vi "FPGA Beam Scanning V3.vi"(1 "Detectors":T1, 3 "Image Acquisition Parameters":T2={"Scan Type"=enum."Sample Scanning", "Scan Mode"=enum."XY", "Fast Axis Frequency (Hz)"=100.0, "Image Format"=128, "Line Accumulations"=1, "Frames Per Capture"=1, "Frames Accumulations"=1, "Image Dimension (um)"=[], "Number of Z Steps"=1, "Z Steps Size (um)"=1.0, "Pixel Size (nm)"=[], "Customized Image Format"=[]} {"Z Steps Size (um)" min=0.0; "Number of Z Steps" min=1; "Frames Accumulations" min=1; "Frames Per Capture" min=1; "Line Accumulations" min=1; "Image Format" items=["64 x 64"=64, "128 x 128"=128, "256 x 256"=256, "512 x 512"=512, "1024 x 1024"=1024, "2048 x 2048"=2048, "Customized..."=0]}) -> ()   [LabVIEW 2014]
uses:
  Type Defs/Image Acquisition Parameters v2.ctl
  Detectors.ctl
  <vilib>/vision/Image Controls.llb/IMAQ Image.ctl
  FPGA-7842R-Reference.ctl
  Focus Lock/Controls/Counter Action.ctl
  <vilib>/FPGAPlugInAG/PCIe-7852R/niLvFpga_Open_PCIe-7852R.vi
  <vilib>/FPGAPlugInAG/PCIe-7852R/niLvFpga_Reset_PCIe-7852R.vi
  <vilib>/Utility/error.llb/Error Cluster From Error Code.vi
  <vilib>/rvi/errors/niLvFpgaAdjustHostInterfaceError.vi
  <vilib>/rvi/interface/common/niFpgaWaitOnOcc.vi
  <vilib>/FPGAPlugInAG/PCIe-7852R/niLvFpga_Run_PCIe-7852R.vi
  <vilib>/FPGAPlugInAG/PCIe-7852R/niLvFpga_Close_PCIe-7852R.vi
  <vilib>/rvi/interface/nirviOpenFPGA/nirviOpenFPGA.xnode
  FPGA Bitfiles/MainSTEDFPGAProj_FPGATarget2_BeamScanningCamb_cWDGwb0YZ5k.lvbitx
  FPGA Target VIs/FPGA-7852R/Beam Scanning Cambridge V1.vi
  <vilib>/rvi/interface/nirviMethod/nirviMethod.xnode
  <vilib>/rvi/interface/nirviReadWriteControl/nirviReadWriteControl.xnode
  <vilib>/rvi/interface/nirviCloseFPGA/nirviCloseFPGA.xnode
  <vilib>/rvi/errors/niLvFpgaMergeErrorWithErrorCode.vi
  <vilib>/vision/NI_Vision_Development_Module.lvlib
  NiFpgaLv.dll
  <vilib>/FPGAPlugInAG/PCIe-7852R/niLvFpga_ReadFifo_PCIe-7852R.vi
  <vilib>/FPGAPlugInAG/PCIe-7852R/niLvFpga_ConfigureFifo_PCIe-7852R.vi
  <vilib>/FPGAPlugInAG/PCIe-7852R/niLvFpga_StartFifo_PCIe-7852R.vi
panel:
  # "Fast Axis"
  # "Slow Axis"
  # "XY"
  # "Z"
  # "Length"
  # "Height"
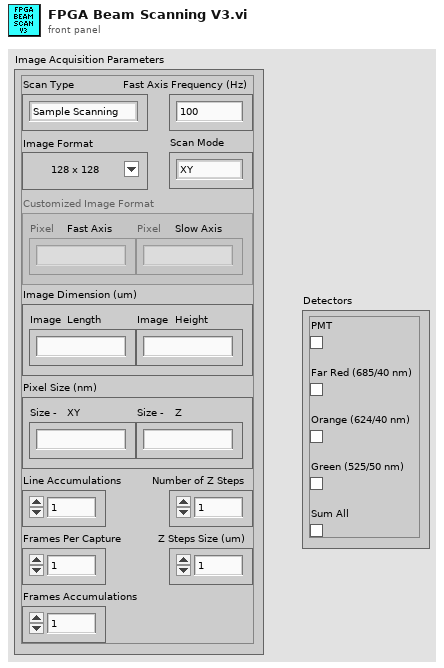
[diagram p1: front panel]
types:
  T1 = typedef "Detectors.ctl" = cluster{"PMT":bool, "Far Red (685/40 nm)":bool, "Orange (624/40 nm)":bool, "Green (525/50 nm)":bool, "Sum All":bool}
  T2 = typedef "Image Acquisition Parameters v2.ctl" = cluster{"Scan Type":enum16{"Sample Scanning", "Beam Scanning"}, "Scan Mode":enum16{"XY", "XZ", "YZ", "XYZ"}, "Fast Axis Frequency (Hz)":dbl, "Image Format":u16, "Line Accumulations":u16, "Frames Per Capture":u16, "Frames Accumulations":u16, "Image Dimension (um)":dbl[], "Number of Z Steps":u8, "Z Steps Size (um)":dbl, "Pixel Size (nm)":dbl[], "Customized Image Format":dbl[]}
  T3 = typedef "IMAQ Image.ctl" = refnum<image>
  T4 = enum16{"big-endian, network order", "native, host order", "little-endian"}
  T5 = typedef "Image Acquisition Parameters.ctl" = cluster{"Scan Type":enum16{"Sample Scanning", "Beam Scanning"}, "Scan Mode":enum16{"XY", "XZ", "YZ", "XYZ"}, "Fast Axis Frequency (Hz)":dbl, "Image Format":u16, "Line Accumulations":u16, "Frames Per Capture":u16, "Frames Accumulations":u16, "Image Dimension (um)":dbl[], "Number of Z Steps":u8, "Z Steps Size (um)":dbl, "Pixel Size (nm)":dbl[]}
  T6 = cluster{"FPGA Sampling Period (ns)":dbl, "Counting Period (us)":dbl, "Samples Per Counting Period":i32, "Start Time (us)":dbl, "Stop Time (us)":dbl, "Normalized Scan End Position":dbl, "Normalized Scan Start Position":dbl}
  T7 = typedef "Scan Parameters.ctl" = cluster{"Fast_Ax_Amp_V":dbl, "Fast_Ax_Off_V":dbl, "Slow_Ax_Amp_V":dbl, "Slow_Ax_Off_V ":dbl, "Slow_Ax_Max_V_VperS":dbl, "Slow_Ax1_Del25ns":i32, "Slow_Ax2_Del25ns":i32, "Stage_X_Off_V":dbl, "Stage_Y_Off_V":dbl, "Stage_Z_Off_V":dbl, "Galvo1_Off_V":dbl, "Galvo2_Off_V":dbl, "Last_Scan_Mode":enum16{"XY", "XZ", "YZ", "XYZ"}, "Current_Scan_Mode":enum16{"XY", "XZ", "YZ", "XYZ"}, "Fly_Back_Lines":u16, "Linear_Ramp_End":u32, "Z_Step_I16":i16, "Z_Start_I16":i16, "Laser_States _U32":u32, "590_Voltage_I16":i16, "775_AOM_Volt_I16":i16, "Blanking OFF":bool, "Unused_Axis_I16":i16}
  T8 = typedef "FPGA-7842R-Reference.ctl" = enum16{"Stage Control", "Laser Control", "Unused Axis I16", "Exit", "Set Res Mirror", "Set Galvo", "Current Frame for Capture", "Default", "Close FPGA", "Stop Waveforms", "Start Waveforms", "Shutter Control", "Initialize"}
  T9 = typedef "Counter Action.ctl" = enum16{"Zero", "Plus One", "Read"}
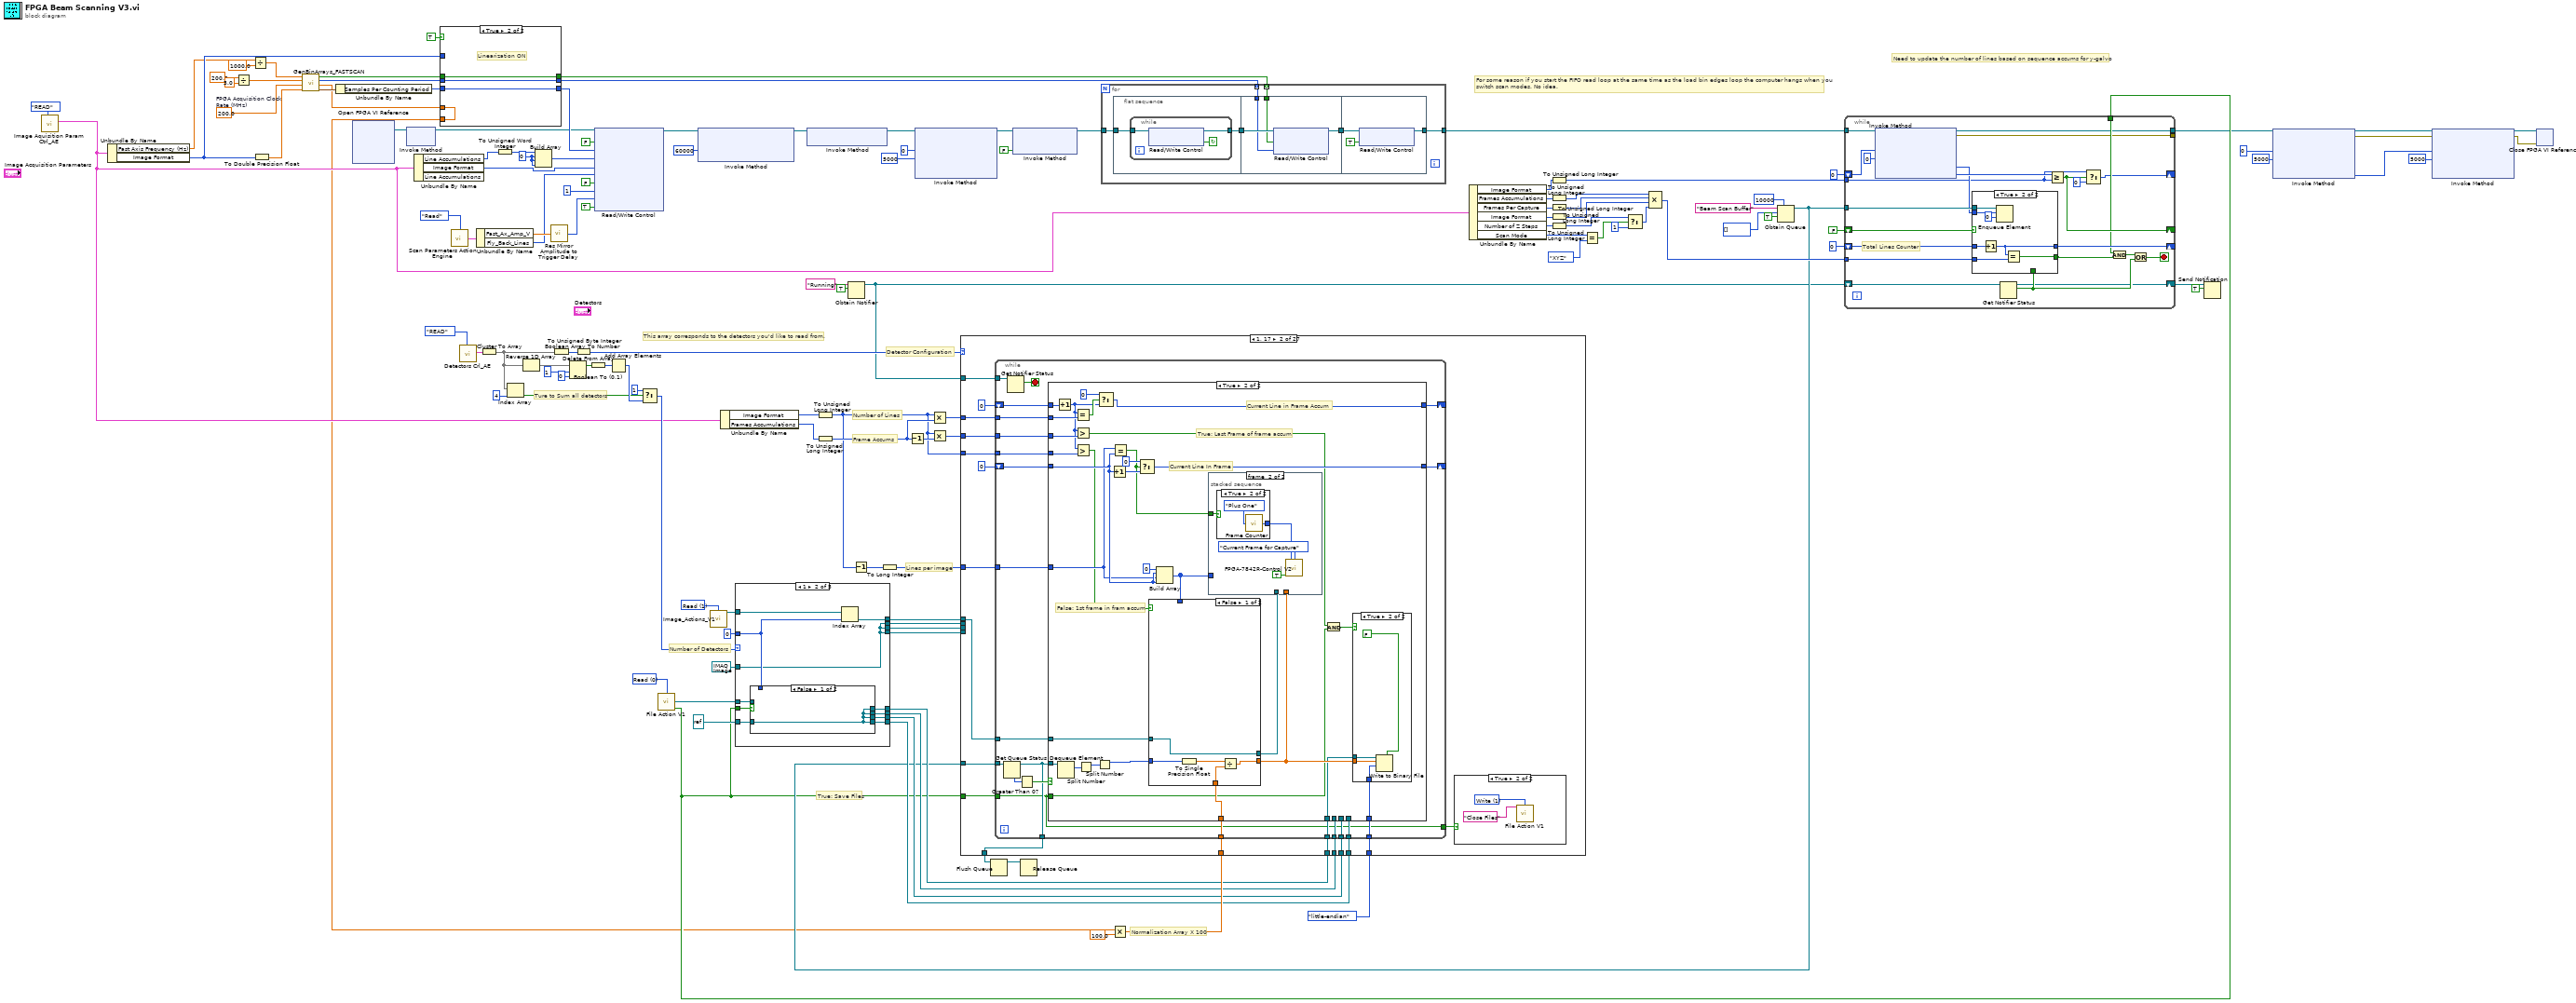
[diagram p0: block diagram]
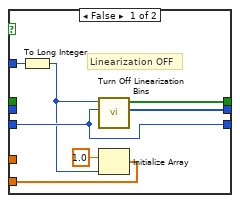
[diagram p2: hidden frame]
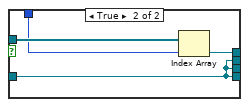
[diagram p4: hidden frame]
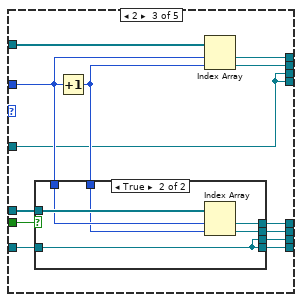
[diagram p5: hidden frame]
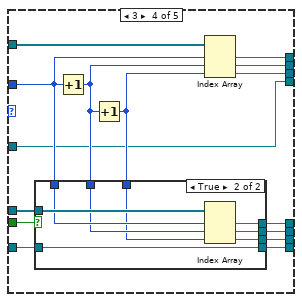
[diagram p7: hidden frame]
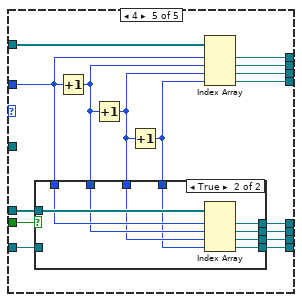
[diagram p9: hidden frame]
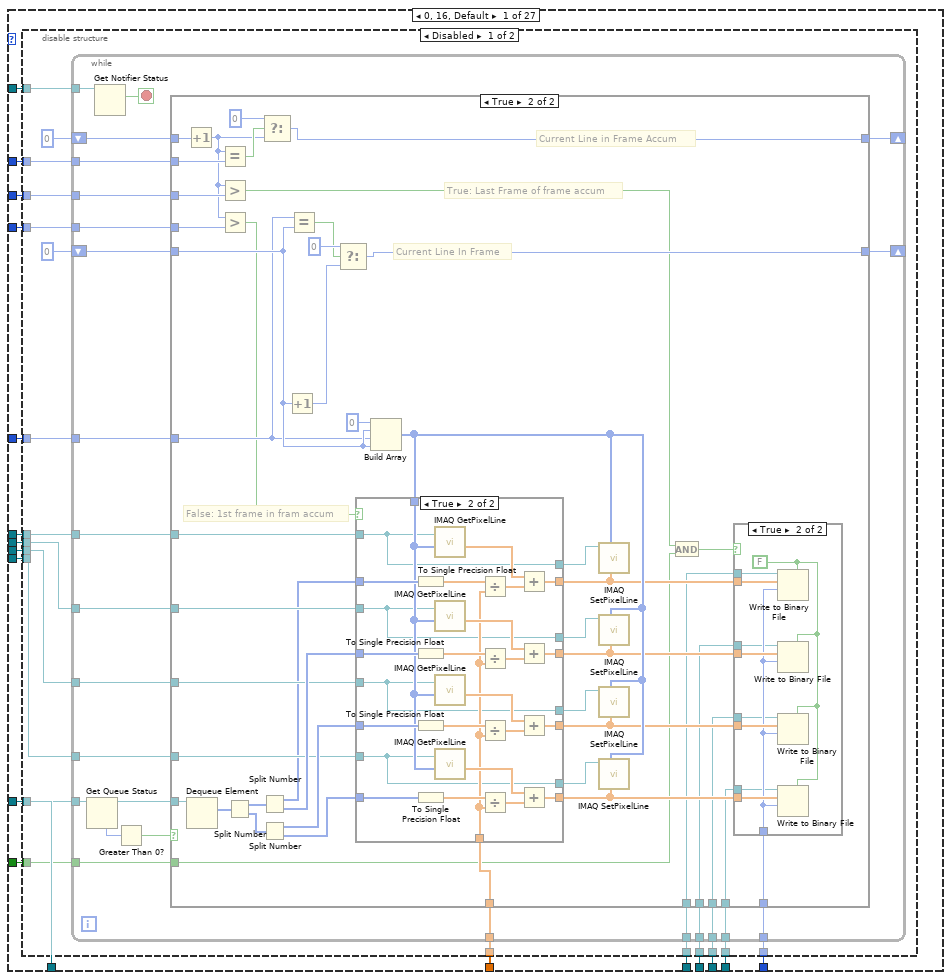
[diagram p11: hidden frame]
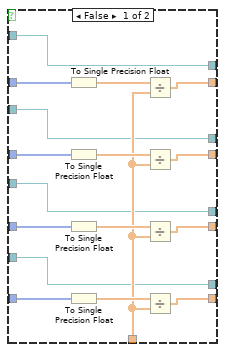
[diagram p14: hidden frame]
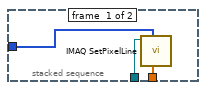
[diagram p18: hidden frame]
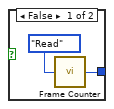
[diagram p19: hidden frame]
diagram:
  w44 = u16 0 items=["Read", "Write"] ("Mode")
  w45 = u16 0 ("element")
  w84 = u16 1 items=["Write", "Read"] ("Mode")
  w128 = 200.0  # FPGA Acquisition Clock Rate (MHz)
  # "Normalization Array X 100"
  # "This array corresponds to the detectors you'd like to read from."
  # "Ture to Sum all detectors"
  # "Number of Detectors"
  # "Detector Configuration"
  # "Frame Accums"
  # "Number of Lines"
  # "True: Save Files"
  # "Lines per image"
  # "For some reason if you start the FIFO read loop at the same time as the load bin edges loop the computer hangs when you\nswitch scan modes. No idea."
  # "Need to update the number of lines based on sequence accums for y-galvo"
  n1 = call "Image Aquisition Param Ctrl_AE.vi"("Action"=enum16{"READ", "WRITE"}."READ") -> ("Image Acquisition Parameters Out"=w33:T5)  [unwired: 10 in]
  n2 = Unbundle By Name(w33) -> ("Fast Axis Frequency (Hz)"=w18:dbl, "Image Format"=w24:u16)
  n3 = Divide(x=200.0, y=3.0) -> (x/y=w125:dbl)
  n4 = Divide(x=w18, y=1000.0) -> (x/y=w19:dbl)
  n5 = To Double Precision Float(number=w24) -> (double precision float=w111:dbl)
  n6 = call "GenBinArrays_FASTSCAN.vi"("Pixels Per Line"=w111, "FPGA Acquisition Clock Rate (MHz)"=w128, "Collection Percent (%)"=w125, "Scan Rate (kHz)"=w19) -> ("Reported Parameters"=w31:T6, "Normalization Array"=w23:sgl[], "Pre Binned Counts (x100)"=w28:u32[], "FPGA Bin Edges"=w30:bool[])
  n7 = Unbundle By Name(w31) -> ("Samples Per Counting Period"=w26:i32)
  n8 = xnode "Open FPGA VI Reference"() -> ("FPGA VI Reference Out"=w6:refnum<k20>)  [unwired: 2 in, 1 out]
  n9 = xnode "Invoke Method"("FPGA VI Reference In"=w6) -> ("FPGA VI Reference Out"=w5:refnum<k20>)  [unwired: 1 in, 1 out]
  n10 = Unbundle By Name(w33) -> ("Line Accumulations"=w53:u16, "Image Format"=w51:u16)  [unwired: 1 out]
  n11 = case shown="True" TRUE {
    tunnel: w30 -> [_ w141]
    tunnel: [w137 w141] -> w29
    tunnel: w28 -> [_ w140]
    tunnel: [w136 w140] -> w27
    tunnel: w26 -> [w135 w139]
    tunnel: [w135 w139] -> w25
    tunnel: w24 -> [w134 _]
    tunnel: w23 -> [_ w138]
    tunnel: [w131 w138] -> w22
    frame False {
      # "Linearization OFF"
      n12 = To Long Integer(number=w134) -> (32bit integer=w132:i32)
      n13 = call "Turn Off Linearization Bins.vi"("Number of Samples"=w135, "Number of Pixels"=w132) -> ("Pre Binned Values"=w136:u32[], "Equal Edges Array"=w137:bool[])  [unwired: 8 in]
      n14 = Initialize Array(sgl 1.0 ("element"), w132) -> (w131:sgl[])
    }
    frame True {
      # "Linearization ON"
    }
  }
  n15 = call "Scan Parameters Action Engine.vi"("Action"=enum16{"Read", "Write"}."Read") -> ("Scan Parameters OUT"=w49:T7)  [unwired: 14 in]
  n16 = call "Detectors Crl_AE.vi"("Action"=enum16{"READ", "WRITE"}."READ") -> ("Detectors Parameters Out"=w34:T1)  [unwired: 10 in]
  n17 = Unbundle By Name(w49) -> ("Fast_Ax_Amp_V"=w42:dbl, "Fly_Back_Lines"=w2:u16)
  n18 = Cluster To Array(cluster=w34) -> (array=w39:bool[])
  n19 = To Unsigned Word Integer(number=w53) -> (unsigned 16bit integer=w52:u16)
  n20 = Index Array(array=w39, index=4) -> (element=w37:bool)
  n21 = Reverse 1D Array(array=w39) -> (reversed array=w67:bool[])
  n22 = Build Array(w52, w45, w45, w45) -> (w8:u16[])
  n23 = call "Res Mirror Amplitude to Trigger Delay.vi"("Amplitude (V)"=w42) -> ("Trigger Delay (Ticks)"=w1:u16)
  n24 = Boolean Array To Number(Boolean array=w39) -> (number=w41:u32)
  n25 = Delete From Array(array=w67, length=1, index=0) -> (array with subset deleted=w71:bool[])  [unwired: 1 out]
  n26 = To Unsigned Byte Integer(number=w41) -> (unsigned 8bit integer=w40:u8)
  n27 = Boolean To (0,1)(Boolean=w71) -> (0, 1=w70:i16[])
  n28 = xnode "Read/Write Control"("FPGA VI Reference In"=w5, "Ready For Write"=FALSE, "FPGA Samples"=w25, "Accums Per Line"=w8, "Lines Per Image"=w51, "Dead Lines"=w2, "Line Trigger"=FALSE, "Sequences"=u8 1, "Trigger Delay (Ticks)"=w1, "Stop Acquisition"=TRUE) -> ("FPGA VI Reference Out"=w130:refnum<k20>)  [unwired: 1 in, 1 out]
  n29 = Add Array Elements(numeric array=w70) -> (sum=w69:i16)
  n30 = Select(t=i16 1, s=w37, f=w69) -> (s? t:f=w64:i16)
  n31 = call "File Action V1.vi"("Mode"=w44) -> ("File REFs"=w81:refnum<file>[], "Files Open"=w43:bool)  [unwired: 12 in, 1 out]
  n32 = xnode "Invoke Method"("FPGA VI Reference In"=w130, "Requested Depth"=u32 60000) -> ("FPGA VI Reference Out"=w109:refnum<k20>)  [unwired: 1 in, 2 out]
  n33 = call "Image_Actions_V1.vi"("Mode"=w84) -> ("Image REFs OUT"=w83:T3[])  [unwired: 13 in, 1 out]
  n34 = Unbundle By Name(w33) -> ("Image Format"=w102:u16, "Frames Accumulations"=w101:u16)
  n35 = case shown="1" w64 {
    tunnel: [w143 w144 w160 w180 w219] -> w76
    tunnel: [w143 w144 w160 w194 w218] -> w77
    tunnel: [w143 w144 w172 w193 w217] -> w78
    tunnel: [w143 w154 w171 w192 w216] -> w79
    tunnel: 0 ("Offset") -> [_ w150 w167 w188 w212]
    tunnel: w83 -> [_ w153 w170 w191 w215]
    tunnel: T3 refnum ("New Image") -> [w143 w144 w160 w180 _]
    tunnel: w81 -> [_ w151 w168 w189 w213]
    tunnel: w43 -> [_ w152 w169 w190 w214]
    tunnel: [w142 w149 w165 w185 w208] -> w75
    tunnel: [w142 w148 w164 w184 w207] -> w74
    tunnel: [w142 w147 w163 w183 w206] -> w73
    tunnel: [w142 w146 w162 w182 w205] -> w72
    tunnel: refnum<file> refnum ("element") -> [w142 w145 w161 w181 w204]
    frame 0, Default {
    }
    frame 1 {
      n36 = case shown="False" w152 {
        tunnel: w151 -> [_ w159]
        tunnel: w150 -> [_ w158]
        tunnel: [w155 w157] -> w149
        tunnel: [w155 w156] -> w148
        tunnel: [w155 w156] -> w147
        tunnel: [w155 w156] -> w146
        tunnel: w145 -> [w155 w156]
        frame False {
        }
        frame True {
          n37 = Index Array(array=w159, index=w158) -> (element=w157:refnum<file>)
        }
      }
      n38 = Index Array(array=w153, index=w150) -> (element=w154:T3)
    }
    frame 2 {
      n39 = Increment(x=w167) -> (x+1=w166:i32)
      n40 = case shown="True" w169 {
        tunnel: w168 -> [_ w179]
        tunnel: w167 -> [_ w178]
        tunnel: w166 -> [_ w177]
        tunnel: [w173 w176] -> w165
        tunnel: [w173 w175] -> w164
        tunnel: [w173 w174] -> w163
        tunnel: [w173 w174] -> w162
        tunnel: w161 -> [w173 w174]
        frame False {
        }
        frame True {
          n41 = Index Array(array=w179, index #1=w178, index #2=w177) -> (element #1=w176:refnum<file>, element #2=w175:refnum<file>)
        }
      }
      n42 = Index Array(array=w170, index #1=w167, index #2=w166) -> (element #1=w171:T3, element #2=w172:T3)
    }
    frame 3 {
      n43 = Increment(x=w188) -> (x+1=w187:i32)
      n44 = Increment(x=w187) -> (x+1=w186:i32)
      n45 = case shown="True" w190 {
        tunnel: w189 -> [_ w203]
        tunnel: w188 -> [_ w202]
        tunnel: w187 -> [_ w201]
        tunnel: w186 -> [_ w200]
        tunnel: [w195 w199] -> w185
        tunnel: [w195 w198] -> w184
        tunnel: [w195 w197] -> w183
        tunnel: [w195 w196] -> w182
        tunnel: w181 -> [w195 w196]
        frame False {
        }
        frame True {
          n46 = Index Array(array=w203, index #1=w202, index #2=w201, index #3=w200) -> (element #1=w199:refnum<file>, element #2=w198:refnum<file>, element #3=w197:refnum<file>)
        }
      }
      n47 = Index Array(array=w191, index #1=w188, index #2=w187, index #3=w186) -> (element #1=w192:T3, element #2=w193:T3, element #3=w194:T3)
    }
    frame 4 {
      n48 = Increment(x=w212) -> (x+1=w211:i32)
      n49 = Increment(x=w211) -> (x+1=w210:i32)
      n50 = Increment(x=w210) -> (x+1=w209:i32)
      n51 = case shown="True" w214 {
        tunnel: w213 -> [_ w229]
        tunnel: w212 -> [_ w228]
        tunnel: w211 -> [_ w227]
        tunnel: w210 -> [_ w226]
        tunnel: w209 -> [_ w225]
        tunnel: [w220 w224] -> w208
        tunnel: [w220 w223] -> w207
        tunnel: [w220 w222] -> w206
        tunnel: [w220 w221] -> w205
        tunnel: w204 -> [w220 _]
        frame False {
        }
        frame True {
          n52 = Index Array(array=w229, index #1=w228, index #2=w227, index #3=w226, index #4=w225) -> (element #1=w224:refnum<file>, element #2=w223:refnum<file>, element #3=w222:refnum<file>, element #4=w221:refnum<file>)
        }
      }
      n53 = Index Array(array=w215, index #1=w212, index #2=w211, index #3=w210, index #4=w209) -> (element #1=w216:T3, element #2=w217:T3, element #3=w218:T3, element #4=w219:T3)
    }
  }
  n54 = xnode "Invoke Method"("FPGA VI Reference In"=w109) -> ("FPGA VI Reference Out"=w110:refnum<k20>)  [unwired: 1 in, 1 out]
  n55 = To Unsigned Long Integer(number=w102) -> (unsigned 32bit integer=w87:u32)
  n56 = To Unsigned Long Integer(number=w101) -> (unsigned 32bit integer=w88:u32)
  n57 = Obtain Notifier(name (unnamed)="Running", notification data type=TRUE) -> (notifier out=w32:refnum<notifier>)  [unwired: 2 in, 2 out]
  n58 = Decrement(x=w87) -> (x-1=w85:u32)
  n59 = To Long Integer(number=w85) -> (32bit integer=w93:i32)
  n60 = Decrement(x=w88) -> (x-1=w91:u32)
  n61 = xnode "Invoke Method"("FPGA VI Reference In"=w110, "Number of Elements"=u32 0, "Timeout (ms)"=5000) -> ("FPGA VI Reference Out"=w129:refnum<k20>)  [unwired: 1 in, 3 out]
  n62 = Multiply(x=w87, y=w88) -> (x*y=w89:u32)
  n63 = Multiply(x=w87, y=w91) -> (x*y=w90:u32)
  n64 = xnode "Invoke Method"("FPGA VI Reference In"=w129, "Wait Until Done (F)"=FALSE) -> ("FPGA VI Reference Out"=w124:refnum<k20>)  [unwired: 1 in, 1 out]
  n65 = for {
    tunnel: [w233] -> w99
    tunnel: w124 -> [w232]
    tunnel: w29 -> [w231] mode=indexing
    tunnel: w27 -> [w230] mode=indexing
    n66 = flat-sequence {
      tunnel: [w237] -> w235
      tunnel: w232 -> [w236]
      tunnel: w235 -> [w244]
      tunnel: [w243] -> w234
      tunnel: w231 -> [w242]
      tunnel: w230 -> [w241]
      tunnel: w234 -> [w247]
      tunnel: [w246] -> w233
      frame #0 {
        n67 = while {
          tunnel: [w240] -> w237
          tunnel: w236 -> [w239]
          stop <- w238 continue-if-true
          n68 = xnode "Read/Write Control"("FPGA VI Reference In"=w239) -> ("FPGA VI Reference Out"=w240:refnum<k20>, "Ready For Write"=w238:bool)  [unwired: 1 in, 1 out]
        }
      }
      frame #1 {
        n69 = xnode "Read/Write Control"("FPGA VI Reference In"=w244, "BinEdge"=w242, "PreBinnedValue"=w241) -> ("FPGA VI Reference Out"=w243:refnum<k20>)  [unwired: 1 in, 1 out]
      }
      frame #2 {
        n70 = xnode "Read/Write Control"("FPGA VI Reference In"=w247, "Ready For Write"=TRUE) -> ("FPGA VI Reference Out"=w246:refnum<k20>)  [unwired: 1 in, 1 out]
      }
    }
  }
  n71 = Multiply(x=w22, y=sgl 100.0) -> (x*y=w100:sgl[])
  n72 = Unbundle By Name(w33) -> ("Image Format"=w116:u16, "Frames Accumulations"=w61:u16, "Frames Per Capture"=w117:u16, "Image Format"=w62:u16, "Number of Z Steps"=w58:u8, "Scan Mode"=w59:enum16{"XY", "XZ", "YZ", "XYZ"})
  n73 = To Unsigned Long Integer(number=w116) -> (unsigned 32bit integer=w123:u32)
  n74 = To Unsigned Long Integer(number=w61) -> (unsigned 32bit integer=w57:u32)
  n75 = To Unsigned Long Integer(number=w117) -> (unsigned 32bit integer=w56:u32)
  n76 = To Unsigned Long Integer(number=w62) -> (unsigned 32bit integer=w55:u32)
  n77 = To Unsigned Long Integer(number=w58) -> (unsigned 32bit integer=w54:u32)
  n78 = Equal?(x=w59, y=enum16{"XY", "XZ", "YZ", "XYZ"}."XYZ") -> (x = y?=w105:bool)
  n79 = Select(t=w54, s=w105, f=u32 1) -> (s? t:f=w104:u32)
  n80 = Compound Arithmetic op=MULTIPLY(w57, w56, w55, w104) -> (w118:u32)
  n81 = Obtain Queue(max queue size (-1, unlimited)=10000, name (unnamed)="Beam Scan Buffer", element data type=u64[] [], create if not found? (T)=TRUE) -> (queue out=w47:refnum<queue>)  [unwired: 1 in, 2 out]
  n82 = case shown="1, 17" w40 {
    tunnel: w93 -> [w264 w426 w526 w626 w743 w842 w961 w1081 w1217 w1316 w1435 w1555 w1692 w1811 w1949 w2088 w2242 w2342 w2443 w2544 w2647 w2748 w2849 w2952 w3052 w3155 w3258]
    tunnel: w43 -> [w261 w423 w523 w623 w740 w839 w958 w1078 w1214 w1313 w1432 w1552 w1689 w1808 w1946 w2085 w2239 w2339 w2440 w2541 w2644 w2745 w2846 w2949 w3049 w3152 w3255]
    tunnel: T4."little-endian" ("byte order (0:big-endian, network order)") -> [w263 w425 w525 w625 w742 w841 w960 w1080 w1216 w1315 w1434 w1554 w1691 w1810 w1948 w2087 w2241 w2341 w2442 w2543 w2646 w2747 w2848 w2951 w3051 w3154 w3257]
    tunnel: w100 -> [w262 w424 w524 w624 w741 w840 w959 w1079 w1215 w1314 w1433 w1553 w1690 w1809 w1947 w2086 w2240 w2340 w2441 w2542 w2645 w2746 w2847 w2950 w3050 w3153 w3256]
    tunnel: w90 -> [w260 w421 w521 w621 w738 w837 w956 w1076 w1212 w1311 w1430 w1550 w1687 w1806 w1944 w2083 w2237 w2337 w2438 w2539 w2642 w2743 w2844 w2947 w3047 w3150 w3253]
    tunnel: w89 -> [w259 w420 w520 w620 w737 w836 w955 w1075 w1211 w1310 w1429 w1549 w1686 w1805 w1943 w2082 w2236 w2336 w2437 w2538 w2641 w2742 w2843 w2946 w3046 w3149 w3252]
    tunnel: w87 -> [w258 w419 w519 w619 w736 w835 w954 w1074 w1210 w1309 w1428 w1548 w1685 w1804 w1942 w2081 w2235 w2335 w2436 w2537 w2640 w2741 w2842 w2945 w3045 w3148 w3251]
    tunnel: w47 -> [w257 w418 w518 w612 w735 w834 w953 w1073 w1209 w1308 w1427 w1547 w1684 w1803 w1941 w2080 w2234 w2334 w2435 w2536 w2639 w2740 w2841 w2944 w3044 w3147 w3250]
    tunnel: w79 -> [w252 w413 w513 w614 w730 w829 w948 w1068 w1204 w1303 w1422 w1542 w1679 w1798 w1936 w2075 w2229 w2329 w2430 w2531 w2634 w2735 w2836 w2939 w3039 w3142 w3245]
    tunnel: w78 -> [w251 _ _ w613 _ w828 w947 w1067 _ w1302 w1421 w1541 w1678 w1797 w1935 w2074 _ _ _ _ _ _ _ _ _ _ _]
    tunnel: w77 -> [w250 _ _ _ _ _ _ w1066 _ _ _ w1540 _ w1796 w1934 w2073 _ _ _ _ _ _ _ _ _ _ _]
    tunnel: w76 -> [w249 _ _ _ _ _ _ _ _ _ _ _ _ _ _ w2072 _ _ _ _ _ _ _ _ _ _ _]
    tunnel: [w257 w412 w518 w611 w735 w834 w953 w1073 w1209 w1308 w1427 w1547 w1684 w1803 w1941 w2080 w2234 w2334 w2435 w2536 w2639 w2740 w2841 w2944 w3044 w3147 w3250] -> w46
    tunnel: w75 -> [w256 w417 w517 w618 w734 w833 w952 w1072 w1208 w1307 w1426 w1546 w1683 w1802 w1940 w2079 w2233 w2333 w2434 w2535 w2638 w2739 w2840 w2943 w3043 w3146 w3249]
    tunnel: w74 -> [w255 w416 w516 w617 w733 w832 w951 w1071 w1207 w1306 w1425 w1545 w1682 w1801 w1939 w2078 w2232 w2332 w2433 w2534 w2637 w2738 w2839 w2942 w3042 w3145 w3248]
    tunnel: w73 -> [w254 w415 w515 w616 w732 w831 w950 w1070 w1206 w1305 w1424 w1544 w1681 w1800 w1938 w2077 w2231 w2331 w2432 w2533 w2636 w2737 w2838 w2941 w3041 w3144 w3247]
    tunnel: w72 -> [w253 w414 w514 w615 w731 w830 w949 w1069 w1205 w1304 w1423 w1543 w1680 w1799 w1937 w2076 w2230 w2330 w2431 w2532 w2635 w2736 w2837 w2940 w3040 w3143 w3246]
    tunnel: w32 -> [w248 w410 w512 w610 w729 w827 w946 w1065 w1203 w1301 w1420 w1539 w1677 w1795 w1933 w2071 w2228 w2328 w2429 w2530 w2633 w2734 w2835 w2938 w3038 w3141 w3244]
    frame 0, 16, Default {
      n83 = disable-structure shown="Disabled" {
        disable-tunnel: w264 -> [w282 _]
        disable-tunnel: w263 -> [w281 _]
        disable-tunnel: w262 -> [w280 _]
        disable-tunnel: w261 -> [w279 _]
        disable-tunnel: w248 -> [w278 _]
        disable-tunnel: w260 -> [w276 _]
        disable-tunnel: w259 -> [w275 _]
        disable-tunnel: w258 -> [w274 _]
        disable-tunnel: w257 -> [w273 _]
        disable-tunnel: w256 -> [w272 _]
        disable-tunnel: w255 -> [w271 _]
        disable-tunnel: w254 -> [w270 _]
        disable-tunnel: w253 -> [w269 _]
        disable-tunnel: w252 -> [w268 _]
        disable-tunnel: w251 -> [w267 _]
        disable-tunnel: w250 -> [w266 _]
        disable-tunnel: w249 -> [w265 _]
        frame Disabled {
          n84 = while {
            shift-right: [w306] -> _
            shift-left: 0 -> [w307]
            tunnel: w282 -> [w308]
            tunnel: w281 -> [w305]
            tunnel: w280 -> [w304]
            tunnel: w279 -> [w303]
            tunnel: w278 -> [w299]
            shift-right: [w296] -> _
            shift-left: u32 0 -> [w297]
            tunnel: w276 -> [w295]
            tunnel: w275 -> [w294]
            tunnel: w274 -> [w293]
            tunnel: w273 -> [w292]
            tunnel: w268 -> [w291]
            tunnel: w267 -> [w290]
            tunnel: w266 -> [w289]
            tunnel: w265 -> [w288]
            tunnel: w272 -> [w287]
            tunnel: w271 -> [w286]
            tunnel: w270 -> [w285]
            tunnel: w269 -> [w284]
            stop <- w298 stop-if-true
            n85 = Get Queue Status(queue=w292) -> (queue out=w300:refnum<queue>, # elements in queue=w302:i32)  [unwired: 2 in, 6 out]
            n86 = Get Notifier Status(notifier=w299) -> (current notification=w298:bool)  [unwired: 1 in, 4 out]
            n87 = Greater Than 0?(x=w302) -> (x > 0?=w301:bool)
            n88 = case shown="True" w301 {
              tunnel: w308 -> [_ w345]
              tunnel: w307 -> [w310 w346]
              tunnel: [w310 w344] -> w306
              tunnel: w305 -> [_ w338]
              tunnel: w304 -> [_ w337]
              tunnel: w303 -> [_ w327]
              tunnel: w300 -> [_ w336]
              tunnel: w297 -> [w309 w333]
              tunnel: [w309 w332] -> w296
              tunnel: w295 -> [_ w331]
              tunnel: w294 -> [_ w330]
              tunnel: w293 -> [_ w325]
              tunnel: w291 -> [_ w323]
              tunnel: w290 -> [_ w322]
              tunnel: w289 -> [_ w321]
              tunnel: w288 -> [_ w320]
              tunnel: w287 -> [_ w314]
              tunnel: w286 -> [_ w313]
              tunnel: w285 -> [_ w312]
              tunnel: w284 -> [_ w311]
              frame False {
              }
              frame True {
                # "False: 1st frame in fram accum"
                # "True: Last Frame of frame accum"
                # "Current Line in Frame Accum"
                # "Current Line In Frame"
                n89 = Increment(x=w333) -> (x+1=w326:u32)
                n90 = Dequeue Element(queue=w336) -> (element=w355:u64[])  [unwired: 2 in, 3 out]
                n91 = Equal?(x=w326, y=w330) -> (x = y?=w335:bool)
                n92 = Greater?(x=w326, y=w331) -> (0:w328:bool)
                n93 = Greater?(x=w326, y=w325) -> (0:w324:bool)
                n94 = Split Number(x=w355) -> (hi(x)=w356:u32[], lo(x)=w354:u32[])
                n95 = Split Number(x=w356) -> (hi(x)=w315:u16[], lo(x)=w353:u16[])
                n96 = Split Number(x=w354) -> (hi(x)=w352:u16[], lo(x)=w351:u16[])
                n97 = Select(t=u32 0, s=w335, f=w326) -> (s? t:f=w332:u32)
                n98 = Increment(x=w346) -> (x+1=w348:i32)
                n99 = Equal?(x=w345, y=w346) -> (x = y?=w347:bool)
                n100 = Select(t=0, s=w347, f=w348) -> (s? t:f=w344:i32)
                n101 = Build Array(0, w346, w345, w346) -> (w343:i32[])
                n102 = case shown="True" w324 {
                  tunnel: w315 -> [w382 w409]
                  tunnel: w353 -> [w377 w408]
                  tunnel: w352 -> [w376 w407]
                  tunnel: w351 -> [w375 w406]
                  tunnel: [w373 w398] -> w340
                  tunnel: [w374 w397] -> w341
                  tunnel: [w381 w396] -> w342
                  tunnel: [w372 w395] -> w339
                  tunnel: w343 -> [_ w390]
                  tunnel: w337 -> [w371 w388]
                  tunnel: w323 -> [w370 w385]
                  tunnel: w322 -> [w369 w386]
                  tunnel: w321 -> [w368 w387]
                  tunnel: w320 -> [w367 w384]
                  tunnel: [w368 w387] -> w317
                  tunnel: [w369 w386] -> w318
                  tunnel: [w370 w385] -> w319
                  tunnel: [w367 w384] -> w316
                  frame False {
                    n103 = To Single Precision Float(number=w382) -> (single precision float=w383:sgl[])
                    n104 = To Single Precision Float(number=w377) -> (single precision float=w380:sgl[])
                    n105 = To Single Precision Float(number=w376) -> (single precision float=w379:sgl[])
                    n106 = To Single Precision Float(number=w375) -> (single precision float=w378:sgl[])
                    n107 = Divide(x=w383, y=w371) -> (x/y=w381:sgl[])
                    n108 = Divide(x=w380, y=w371) -> (x/y=w374:sgl[])
                    n109 = Divide(x=w379, y=w371) -> (x/y=w373:sgl[])
                    n110 = Divide(x=w378, y=w371) -> (x/y=w372:sgl[])
                  }
                  frame True {
                    n111 = To Single Precision Float(number=w409) -> (single precision float=w389:sgl[])
                    n112 = To Single Precision Float(number=w408) -> (single precision float=w405:sgl[])
                    n113 = To Single Precision Float(number=w407) -> (single precision float=w404:sgl[])
                    n114 = To Single Precision Float(number=w406) -> (single precision float=w403:sgl[])
                    n115 = call "IMAQ GetPixelLine"("Line Coordinates"=w390, "Image"=w385) -> ("Pixels Line (Float)"=w394:sgl[])  [unwired: 2 in, 4 out]
                    n116 = call "IMAQ GetPixelLine"("Line Coordinates"=w390, "Image"=w386) -> ("Pixels Line (Float)"=w393:sgl[])  [unwired: 2 in, 4 out]
                    n117 = call "IMAQ GetPixelLine"("Line Coordinates"=w390, "Image"=w387) -> ("Pixels Line (Float)"=w392:sgl[])  [unwired: 2 in, 4 out]
                    n118 = call "IMAQ GetPixelLine"("Line Coordinates"=w390, "Image"=w384) -> ("Pixels Line (Float)"=w391:sgl[])  [unwired: 2 in, 4 out]
                    n119 = Divide(x=w389, y=w388) -> (x/y=w402:sgl[])
                    n120 = Divide(x=w405, y=w388) -> (x/y=w401:sgl[])
                    n121 = Divide(x=w404, y=w388) -> (x/y=w400:sgl[])
                    n122 = Divide(x=w403, y=w388) -> (x/y=w399:sgl[])
                    n123 = Add(x=w394, y=w402) -> (x+y=w396:sgl[])
                    n124 = Add(x=w393, y=w401) -> (x+y=w397:sgl[])
                    n125 = Add(x=w392, y=w400) -> (x+y=w398:sgl[])
                    n126 = Add(x=w391, y=w399) -> (x+y=w395:sgl[])
                  }
                }
                n127 = call "IMAQ SetPixelLine"("Pixels Line (Float)"=w342, "Line Coordinates"=w343, "Image"=w319) -> ()  [unwired: 7 in, 2 out]
                n128 = call "IMAQ SetPixelLine"("Pixels Line (Float)"=w341, "Line Coordinates"=w343, "Image"=w318) -> ()  [unwired: 7 in, 2 out]
                n129 = call "IMAQ SetPixelLine"("Pixels Line (Float)"=w340, "Line Coordinates"=w343, "Image"=w317) -> ()  [unwired: 7 in, 2 out]
                n130 = call "IMAQ SetPixelLine"("Pixels Line (Float)"=w339, "Line Coordinates"=w343, "Image"=w316) -> ()  [unwired: 7 in, 2 out]
                n131 = And(x=w328, y=w327) -> (x .and. y?=w329:bool)
                n132 = case shown="True" w329 {
                  tunnel: w342 -> [_ w366]
                  tunnel: w341 -> [_ w365]
                  tunnel: w340 -> [_ w364]
                  tunnel: w339 -> [_ w363]
                  tunnel: w338 -> [_ w361]
                  tunnel: w314 -> [_ w360]
                  tunnel: w313 -> [_ w359]
                  tunnel: w312 -> [_ w358]
                  tunnel: w311 -> [_ w357]
                  frame False {
                  }
                  frame True {
                    w362 = FALSE ("prepend array or string size? (T)")
                    n133 = Write to Binary File(file (use dialog)=w360, data=w366, 5:w362, 9:w361) -> ()  [unwired: 2 in, 3 out]
                    n134 = Write to Binary File(file (use dialog)=w359, data=w365, 5:w362, 9:w361) -> ()  [unwired: 2 in, 3 out]
                    n135 = Write to Binary File(file (use dialog)=w358, data=w364, 5:w362, 9:w361) -> ()  [unwired: 2 in, 3 out]
                    n136 = Write to Binary File(file (use dialog)=w357, data=w363, 5:w362, 9:w361) -> ()  [unwired: 2 in, 3 out]
                  }
                }
              }
            }
          }
        }
        frame Enabled {
        }
      }
    }
    frame 1, 17 {
      n137 = while {
        shift-right: [w449] -> _
        shift-left: 0 -> [w450]
        tunnel: w426 -> [w451]
        tunnel: w425 -> [w448]
        tunnel: w424 -> [w447]
        tunnel: w423 -> [w430]
        tunnel: w410 -> [w444]
        shift-right: [w441] -> _
        shift-left: u32 0 -> [w442]
        tunnel: w421 -> [w440]
        tunnel: w420 -> [w439]
        tunnel: w419 -> [w438]
        tunnel: w418 -> [w437]
        tunnel: w413 -> [w436]
        tunnel: w417 -> [w435]
        tunnel: w416 -> [w434]
        tunnel: w415 -> [w433]
        tunnel: w414 -> [w432]
        tunnel: [w431] -> w412
        tunnel: [w430] -> w411
        stop <- w443 stop-if-true
        n138 = Get Queue Status(queue=w437) -> (queue out=w431:refnum<queue>, # elements in queue=w446:i32)  [unwired: 2 in, 6 out]
        n139 = Get Notifier Status(notifier=w444) -> (current notification=w443:bool)  [unwired: 1 in, 4 out]
        n140 = Greater Than 0?(x=w446) -> (x > 0?=w445:bool)
        n141 = case shown="True" w445 {
          tunnel: w451 -> [_ w479]
          tunnel: w450 -> [w453 w480]
          tunnel: [w453 w478] -> w449
          tunnel: w448 -> [_ w475]
          tunnel: w447 -> [_ w474]
          tunnel: w430 -> [_ w457]
          tunnel: w431 -> [_ w473]
          tunnel: w442 -> [w452 w470]
          tunnel: [w452 w469] -> w441
          tunnel: w440 -> [_ w468]
          tunnel: w439 -> [_ w467]
          tunnel: w438 -> [_ w463]
          tunnel: w436 -> [_ w461]
          tunnel: w435 -> [_ w459]
          tunnel: w434 -> [_ _]
          tunnel: w433 -> [_ _]
          tunnel: w432 -> [_ _]
          frame False {
          }
          frame True {
            # "False: 1st frame in fram accum"
            # "True: Last Frame of frame accum"
            # "Current Line in Frame Accum"
            # "Current Line In Frame"
            n142 = Increment(x=w470) -> (x+1=w464:u32)
            n143 = Dequeue Element(queue=w473) -> (element=w482:u64[])  [unwired: 2 in, 3 out]
            n144 = Equal?(x=w464, y=w467) -> (x = y?=w472:bool)
            n145 = Greater?(x=w464, y=w468) -> (0:w465:bool)
            n146 = Greater?(x=w464, y=w463) -> (0:w462:bool)
            n147 = Split Number(x=w482) -> (hi(x)=w483:u32[])  [unwired: 1 out]
            n148 = Split Number(x=w483) -> (hi(x)=w458:u16[])  [unwired: 1 out]
            n149 = Select(t=u32 0, s=w472, f=w464) -> (s? t:f=w469:u32)
            n150 = Increment(x=w480) -> (x+1=w456:i32)
            n151 = Equal?(x=w479, y=w480) -> (x = y?=w454:bool)
            n152 = Select(t=0, s=w454, f=w456) -> (s? t:f=w478:i32)
            n153 = Build Array(0, w480, w479, w480) -> (w477:i32[])
            n154 = case shown="False" w462 {
              tunnel: w458 -> [w502 w511]
              tunnel: [w501 w508] -> w476
              tunnel: w477 -> [_ w506]
              tunnel: w474 -> [w500 w505]
              tunnel: w461 -> [w499 w504]
              tunnel: [w499 w504] -> w460
              frame False {
                n155 = To Single Precision Float(number=w502) -> (single precision float=w503:sgl[])
                n156 = Divide(x=w503, y=w500) -> (x/y=w501:sgl[])
              }
              frame True {
                n157 = To Single Precision Float(number=w511) -> (single precision float=w510:sgl[])
                n158 = call "IMAQ GetPixelLine"("Line Coordinates"=w506, "Image"=w504) -> ("Pixels Line (Float)"=w507:sgl[])  [unwired: 2 in, 4 out]
                n159 = Divide(x=w510, y=w505) -> (x/y=w509:sgl[])
                n160 = Add(x=w507, y=w509) -> (x+y=w508:sgl[])
              }
            }
            n161 = stacked-sequence {
              tunnel: w477 -> [w486 _]
              tunnel: w476 -> [w485 _]
              tunnel: w460 -> [w484 _]
              tunnel: w454 -> [_ w490]
              frame #0 {
                n162 = call "IMAQ SetPixelLine"("Pixels Line (Float)"=w485, "Line Coordinates"=w486, "Image"=w484) -> ()  [unwired: 7 in, 2 out]
              }
              frame #1 {
                n163 = case shown="True" w490 {
                  tunnel: [w491 w493] -> w488
                  frame False {
                    n164 = call "Frame Counter.vi"("Action"=Counter_Action."Read") -> ("Num"=w491:i32)
                  }
                  frame True {
                    n165 = call "Frame Counter.vi"("Action"=Counter_Action."Plus One") -> ("Num"=w493:i32)
                  }
                }
                n166 = call "FPGA-7842R-Control V2.vi"("Current Frame"=w488, "Action"=FPGA-7842R-Reference."Current Frame for Capture", "Initialize"=TRUE) -> ()  [unwired: 11 in, 2 out]
              }
            }
            n167 = And(x=w465, y=w457) -> (x .and. y?=w466:bool)
            n168 = case shown="True" w466 {
              tunnel: w476 -> [_ w498]
              tunnel: w475 -> [_ w496]
              tunnel: w459 -> [_ w495]
              frame False {
              }
              frame True {
                n169 = Write to Binary File(file (use dialog)=w495, data=w498, 5:FALSE ("prepend array or string size? (T)"), 9:w496) -> ()  [unwired: 2 in, 3 out]
              }
            }
          }
        }
      }
      n170 = case shown="True" w411 {
        frame False {
        }
        frame True {
          w429 = u16 1 items=["Read", "Write"] ("Mode")
          n171 = call "File Action V1.vi"("Action"="Close Files", "Mode"=w429) -> ()  [unwired: 11 in, 3 out]
        }
      }
    }
    frame 2, 18 {
      n172 = while {
        shift-right: [w547] -> _
        shift-left: 0 -> [w548]
        tunnel: w526 -> [w549]
        tunnel: w525 -> [w546]
        tunnel: w524 -> [w545]
        tunnel: w523 -> [w544]
        tunnel: w512 -> [w540]
        shift-right: [w537] -> _
        shift-left: u32 0 -> [w538]
        tunnel: w521 -> [w536]
        tunnel: w520 -> [w535]
        tunnel: w519 -> [w534]
        tunnel: w518 -> [w533]
        tunnel: w513 -> [w532]
        tunnel: w517 -> [w531]
        tunnel: w516 -> [w530]
        tunnel: w515 -> [w529]
        tunnel: w514 -> [w528]
        stop <- w539 stop-if-true
        n173 = Get Queue Status(queue=w533) -> (queue out=w541:refnum<queue>, # elements in queue=w543:i32)  [unwired: 2 in, 6 out]
        n174 = Get Notifier Status(notifier=w540) -> (current notification=w539:bool)  [unwired: 1 in, 4 out]
        n175 = Greater Than 0?(x=w543) -> (x > 0?=w542:bool)
        n176 = case shown="True" w542 {
          tunnel: w549 -> [_ w576]
          tunnel: w548 -> [w551 w577]
          tunnel: [w551 w575] -> w547
          tunnel: w546 -> [_ w574]
          tunnel: w545 -> [_ w573]
          tunnel: w544 -> [_ w563]
          tunnel: w541 -> [_ w572]
          tunnel: w538 -> [w550 w569]
          tunnel: [w550 w568] -> w537
          tunnel: w536 -> [_ w567]
          tunnel: w535 -> [_ w566]
          tunnel: w534 -> [_ w561]
          tunnel: w532 -> [_ w559]
          tunnel: w531 -> [_ w558]
          tunnel: w530 -> [_ _]
          tunnel: w529 -> [_ _]
          tunnel: w528 -> [_ _]
          frame False {
          }
          frame True {
            # "False: 1st frame in fram accum"
            # "True: Last Frame of frame accum"
            # "Current Line in Frame Accum"
            # "Current Line In Frame"
            n177 = Increment(x=w569) -> (x+1=w562:u32)
            n178 = Dequeue Element(queue=w572) -> (element=w580:u64[])  [unwired: 2 in, 3 out]
            n179 = Equal?(x=w562, y=w566) -> (x = y?=w571:bool)
            n180 = Greater?(x=w562, y=w567) -> (0:w564:bool)
            n181 = Greater?(x=w562, y=w561) -> (0:w560:bool)
            n182 = Split Number(x=w580) -> (hi(x)=w581:u32[])  [unwired: 1 out]
            n183 = Split Number(x=w581) -> (lo(x)=w557:u16[])  [unwired: 1 out]
            n184 = Select(t=u32 0, s=w571, f=w562) -> (s? t:f=w568:u32)
            n185 = Increment(x=w577) -> (x+1=w578:i32)
            n186 = Equal?(x=w576, y=w577) -> (x = y?=w552:bool)
            n187 = Select(t=0, s=w552, f=w578) -> (s? t:f=w575:i32)
            n188 = Build Array(0, w577, w576, w577) -> (w555:i32[])
            n189 = case shown="True" w560 {
              tunnel: w557 -> [w600 w609]
              tunnel: [w599 w606] -> w553
              tunnel: w555 -> [_ w604]
              tunnel: w573 -> [w598 w603]
              tunnel: w559 -> [w597 w602]
              tunnel: [w597 w602] -> w554
              frame False {
                n190 = To Single Precision Float(number=w600) -> (single precision float=w601:sgl[])
                n191 = Divide(x=w601, y=w598) -> (x/y=w599:sgl[])
              }
              frame True {
                n192 = To Single Precision Float(number=w609) -> (single precision float=w608:sgl[])
                n193 = call "IMAQ GetPixelLine"("Line Coordinates"=w604, "Image"=w602) -> ("Pixels Line (Float)"=w605:sgl[])  [unwired: 2 in, 4 out]
                n194 = Divide(x=w608, y=w603) -> (x/y=w607:sgl[])
                n195 = Add(x=w605, y=w607) -> (x+y=w606:sgl[])
              }
            }
            n196 = stacked-sequence {
              tunnel: w555 -> [w584 _]
              tunnel: w553 -> [w583 _]
              tunnel: w554 -> [w582 _]
              tunnel: w552 -> [_ w588]
              frame #0 {
                n197 = call "IMAQ SetPixelLine"("Pixels Line (Float)"=w583, "Line Coordinates"=w584, "Image"=w582) -> ()  [unwired: 7 in, 2 out]
              }
              frame #1 {
                n198 = case shown="True" w588 {
                  tunnel: [w589 w591] -> w586
                  frame False {
                    n199 = call "Frame Counter.vi"("Action"=Counter_Action."Read") -> ("Num"=w589:i32)
                  }
                  frame True {
                    n200 = call "Frame Counter.vi"("Action"=Counter_Action."Plus One") -> ("Num"=w591:i32)
                  }
                }
                n201 = call "FPGA-7842R-Control V2.vi"("Current Frame"=w586, "Action"=FPGA-7842R-Reference."Current Frame for Capture", "Initialize"=TRUE) -> ()  [unwired: 11 in, 2 out]
              }
            }
            n202 = And(x=w564, y=w563) -> (x .and. y?=w565:bool)
            n203 = case shown="True" w565 {
              tunnel: w553 -> [_ w596]
              tunnel: w574 -> [_ w594]
              tunnel: w558 -> [_ w593]
              frame False {
              }
              frame True {
                n204 = Write to Binary File(file (use dialog)=w593, data=w596, 5:FALSE ("prepend array or string size? (T)"), 9:w594) -> ()  [unwired: 2 in, 3 out]
              }
            }
          }
        }
      }
    }
    frame 3 {
      n205 = while {
        shift-right: [w648] -> _
        shift-left: 0 -> [w649]
        tunnel: w626 -> [w650]
        tunnel: w625 -> [w647]
        tunnel: w624 -> [w646]
        tunnel: w623 -> [w645]
        tunnel: w610 -> [w642]
        shift-right: [w639] -> _
        shift-left: u32 0 -> [w640]
        tunnel: w621 -> [w638]
        tunnel: w620 -> [w637]
        tunnel: w619 -> [w636]
        tunnel: w612 -> [w635]
        tunnel: w614 -> [w634]
        tunnel: w613 -> [w633]
        tunnel: w618 -> [w632]
        tunnel: w617 -> [w631]
        tunnel: w616 -> [w630]
        tunnel: w615 -> [w629]
        tunnel: [w628] -> w611
        stop <- w641 stop-if-true
        n206 = Get Queue Status(queue=w635) -> (queue out=w628:refnum<queue>, # elements in queue=w644:i32)  [unwired: 2 in, 6 out]
        n207 = Get Notifier Status(notifier=w642) -> (current notification=w641:bool)  [unwired: 1 in, 4 out]
        n208 = Greater Than 0?(x=w644) -> (x > 0?=w643:bool)
        n209 = case shown="True" w643 {
          tunnel: w650 -> [_ w682]
          tunnel: w649 -> [w652 w683]
          tunnel: [w652 w681] -> w648
          tunnel: w647 -> [_ w679]
          tunnel: w646 -> [_ w678]
          tunnel: w645 -> [_ w668]
          tunnel: w628 -> [_ w677]
          tunnel: w640 -> [w651 w674]
          tunnel: [w651 w673] -> w639
          tunnel: w638 -> [_ w672]
          tunnel: w637 -> [_ w671]
          tunnel: w636 -> [_ w666]
          tunnel: w634 -> [_ w664]
          tunnel: w633 -> [_ w663]
          tunnel: w632 -> [_ w661]
          tunnel: w631 -> [_ w660]
          tunnel: w630 -> [_ _]
          tunnel: w629 -> [_ _]
          frame False {
          }
          frame True {
            # "False: 1st frame in fram accum"
            # "True: Last Frame of frame accum"
            # "Current Line in Frame Accum"
            # "Current Line In Frame"
            n210 = Increment(x=w674) -> (x+1=w667:u32)
            n211 = Dequeue Element(queue=w677) -> (element=w687:u64[])  [unwired: 2 in, 3 out]
            n212 = Equal?(x=w667, y=w671) -> (x = y?=w676:bool)
            n213 = Greater?(x=w667, y=w672) -> (0:w669:bool)
            n214 = Greater?(x=w667, y=w666) -> (0:w665:bool)
            n215 = Split Number(x=w687) -> (hi(x)=w688:u32[])  [unwired: 1 out]
            n216 = Split Number(x=w688) -> (hi(x)=w659:u16[], lo(x)=w658:u16[])
            n217 = Select(t=u32 0, s=w676, f=w667) -> (s? t:f=w673:u32)
            n218 = Increment(x=w683) -> (x+1=w684:i32)
            n219 = Equal?(x=w682, y=w683) -> (x = y?=w653:bool)
            n220 = Select(t=0, s=w653, f=w684) -> (s? t:f=w681:i32)
            n221 = Build Array(0, w683, w682, w683) -> (w657:i32[])
            n222 = case shown="True" w665 {
              tunnel: w659 -> [w712 w728]
              tunnel: w658 -> [w711 w727]
              tunnel: [w709 w722] -> w680
              tunnel: [w710 w721] -> w654
              tunnel: w657 -> [_ w718]
              tunnel: w678 -> [w708 w717]
              tunnel: w664 -> [w707 w715]
              tunnel: w663 -> [w706 w716]
              tunnel: [w706 w716] -> w662
              tunnel: [w707 w715] -> w655
              frame False {
                n223 = To Single Precision Float(number=w712) -> (single precision float=w714:sgl[])
                n224 = To Single Precision Float(number=w711) -> (single precision float=w713:sgl[])
                n225 = Divide(x=w714, y=w708) -> (x/y=w710:sgl[])
                n226 = Divide(x=w713, y=w708) -> (x/y=w709:sgl[])
              }
              frame True {
                n227 = To Single Precision Float(number=w728) -> (single precision float=w726:sgl[])
                n228 = To Single Precision Float(number=w727) -> (single precision float=w725:sgl[])
                n229 = call "IMAQ GetPixelLine"("Line Coordinates"=w718, "Image"=w715) -> ("Pixels Line (Float)"=w720:sgl[])  [unwired: 2 in, 4 out]
                n230 = call "IMAQ GetPixelLine"("Line Coordinates"=w718, "Image"=w716) -> ("Pixels Line (Float)"=w719:sgl[])  [unwired: 2 in, 4 out]
                n231 = Divide(x=w726, y=w717) -> (x/y=w724:sgl[])
                n232 = Divide(x=w725, y=w717) -> (x/y=w723:sgl[])
                n233 = Add(x=w720, y=w724) -> (x+y=w721:sgl[])
                n234 = Add(x=w719, y=w723) -> (x+y=w722:sgl[])
              }
            }
            n235 = stacked-sequence {
              tunnel: w657 -> [w689 _]
              tunnel: w654 -> [w691 _]
              tunnel: w655 -> [w690 _]
              tunnel: w653 -> [_ w695]
              tunnel: [w689 _] -> w656
              frame #0 {
                n236 = call "IMAQ SetPixelLine"("Pixels Line (Float)"=w691, "Line Coordinates"=w689, "Image"=w690) -> ()  [unwired: 7 in, 2 out]
              }
              frame #1 {
                n237 = case shown="True" w695 {
                  tunnel: [w696 w698] -> w693
                  frame False {
                    n238 = call "Frame Counter.vi"("Action"=Counter_Action."Read") -> ("Num"=w696:i32)
                  }
                  frame True {
                    n239 = call "Frame Counter.vi"("Action"=Counter_Action."Plus One") -> ("Num"=w698:i32)
                  }
                }
                n240 = call "FPGA-7842R-Control V2.vi"("Current Frame"=w693, "Action"=FPGA-7842R-Reference."Current Frame for Capture", "Initialize"=TRUE) -> ()  [unwired: 11 in, 2 out]
              }
            }
            n241 = call "IMAQ SetPixelLine"("Pixels Line (Float)"=w680, "Line Coordinates"=w656, "Image"=w662) -> ()  [unwired: 7 in, 2 out]
            n242 = And(x=w669, y=w668) -> (x .and. y?=w670:bool)
            n243 = case shown="False" w670 {
              tunnel: w654 -> [_ w705]
              tunnel: w680 -> [_ w704]
              tunnel: w679 -> [_ w702]
              tunnel: w661 -> [_ w701]
              tunnel: w660 -> [_ w700]
              frame False {
              }
              frame True {
                w703 = FALSE ("prepend array or string size? (T)")
                n244 = Write to Binary File(file (use dialog)=w701, data=w705, 5:w703, 9:w702) -> ()  [unwired: 2 in, 3 out]
                n245 = Write to Binary File(file (use dialog)=w700, data=w704, 5:w703, 9:w702) -> ()  [unwired: 2 in, 3 out]
              }
            }
          }
        }
      }
    }
    frame 4, 20 {
      n246 = while {
        shift-right: [w764] -> _
        shift-left: 0 -> [w765]
        tunnel: w743 -> [w766]
        tunnel: w742 -> [w763]
        tunnel: w741 -> [w762]
        tunnel: w740 -> [w761]
        tunnel: w729 -> [w757]
        shift-right: [w754] -> _
        shift-left: u32 0 -> [w755]
        tunnel: w738 -> [w753]
        tunnel: w737 -> [w752]
        tunnel: w736 -> [w751]
        tunnel: w735 -> [w750]
        tunnel: w730 -> [w749]
        tunnel: w734 -> [w748]
        tunnel: w733 -> [w747]
        tunnel: w732 -> [w746]
        tunnel: w731 -> [w745]
        stop <- w756 stop-if-true
        n247 = Get Queue Status(queue=w750) -> (queue out=w758:refnum<queue>, # elements in queue=w760:i32)  [unwired: 2 in, 6 out]
        n248 = Get Notifier Status(notifier=w757) -> (current notification=w756:bool)  [unwired: 1 in, 4 out]
        n249 = Greater Than 0?(x=w760) -> (x > 0?=w759:bool)
        n250 = case shown="True" w759 {
          tunnel: w766 -> [_ w792]
          tunnel: w765 -> [w768 w793]
          tunnel: [w768 w791] -> w764
          tunnel: w763 -> [_ w790]
          tunnel: w762 -> [_ w789]
          tunnel: w761 -> [_ w779]
          tunnel: w758 -> [_ w788]
          tunnel: w755 -> [w767 w785]
          tunnel: [w767 w784] -> w754
          tunnel: w753 -> [_ w783]
          tunnel: w752 -> [_ w782]
          tunnel: w751 -> [_ w777]
          tunnel: w749 -> [_ w775]
          tunnel: w748 -> [_ w774]
          tunnel: w747 -> [_ _]
          tunnel: w746 -> [_ _]
          tunnel: w745 -> [_ _]
          frame False {
          }
          frame True {
            # "False: 1st frame in fram accum"
            # "True: Last Frame of frame accum"
            # "Current Line in Frame Accum"
            # "Current Line In Frame"
            n251 = Increment(x=w785) -> (x+1=w778:u32)
            n252 = Dequeue Element(queue=w788) -> (element=w798:u64[])  [unwired: 2 in, 3 out]
            n253 = Equal?(x=w778, y=w782) -> (x = y?=w787:bool)
            n254 = Greater?(x=w778, y=w783) -> (0:w780:bool)
            n255 = Greater?(x=w778, y=w777) -> (0:w776:bool)
            n256 = Split Number(x=w798) -> (lo(x)=w797:u32[])  [unwired: 1 out]
            n257 = Split Number(x=w797) -> (hi(x)=w773:u16[])  [unwired: 1 out]
            n258 = Select(t=u32 0, s=w787, f=w778) -> (s? t:f=w784:u32)
            n259 = Increment(x=w793) -> (x+1=w794:i32)
            n260 = Equal?(x=w792, y=w793) -> (x = y?=w772:bool)
            n261 = Select(t=0, s=w772, f=w794) -> (s? t:f=w791:i32)
            n262 = Build Array(0, w793, w792, w793) -> (w771:i32[])
            n263 = case shown="True" w776 {
              tunnel: w773 -> [w817 w826]
              tunnel: [w816 w823] -> w769
              tunnel: w771 -> [_ w821]
              tunnel: w789 -> [w815 w820]
              tunnel: w775 -> [w814 w819]
              tunnel: [w814 w819] -> w770
              frame False {
                n264 = To Single Precision Float(number=w817) -> (single precision float=w818:sgl[])
                n265 = Divide(x=w818, y=w815) -> (x/y=w816:sgl[])
              }
              frame True {
                n266 = To Single Precision Float(number=w826) -> (single precision float=w825:sgl[])
                n267 = call "IMAQ GetPixelLine"("Line Coordinates"=w821, "Image"=w819) -> ("Pixels Line (Float)"=w822:sgl[])  [unwired: 2 in, 4 out]
                n268 = Divide(x=w825, y=w820) -> (x/y=w824:sgl[])
                n269 = Add(x=w822, y=w824) -> (x+y=w823:sgl[])
              }
            }
            n270 = stacked-sequence {
              tunnel: w771 -> [w801 _]
              tunnel: w769 -> [w800 _]
              tunnel: w770 -> [w799 _]
              tunnel: w772 -> [_ w805]
              frame #0 {
                n271 = call "IMAQ SetPixelLine"("Pixels Line (Float)"=w800, "Line Coordinates"=w801, "Image"=w799) -> ()  [unwired: 7 in, 2 out]
              }
              frame #1 {
                n272 = case shown="True" w805 {
                  tunnel: [w806 w808] -> w803
                  frame False {
                    n273 = call "Frame Counter.vi"("Action"=Counter_Action."Read") -> ("Num"=w806:i32)
                  }
                  frame True {
                    n274 = call "Frame Counter.vi"("Action"=Counter_Action."Plus One") -> ("Num"=w808:i32)
                  }
                }
                n275 = call "FPGA-7842R-Control V2.vi"("Current Frame"=w803, "Action"=FPGA-7842R-Reference."Current Frame for Capture", "Initialize"=TRUE) -> ()  [unwired: 11 in, 2 out]
              }
            }
            n276 = And(x=w780, y=w779) -> (x .and. y?=w781:bool)
            n277 = case shown="True" w781 {
              tunnel: w769 -> [_ w813]
              tunnel: w790 -> [_ w811]
              tunnel: w774 -> [_ w810]
              frame False {
              }
              frame True {
                n278 = Write to Binary File(file (use dialog)=w810, data=w813, 5:FALSE ("prepend array or string size? (T)"), 9:w811) -> ()  [unwired: 2 in, 3 out]
              }
            }
          }
        }
      }
    }
    frame 5 {
      n279 = while {
        shift-right: [w864] -> _
        shift-left: 0 -> [w865]
        tunnel: w842 -> [w866]
        tunnel: w841 -> [w863]
        tunnel: w840 -> [w862]
        tunnel: w839 -> [w861]
        tunnel: w827 -> [w857]
        shift-right: [w854] -> _
        shift-left: u32 0 -> [w855]
        tunnel: w837 -> [w853]
        tunnel: w836 -> [w852]
        tunnel: w835 -> [w851]
        tunnel: w834 -> [w850]
        tunnel: w829 -> [w849]
        tunnel: w828 -> [w848]
        tunnel: w833 -> [w847]
        tunnel: w832 -> [w846]
        tunnel: w831 -> [w845]
        tunnel: w830 -> [w844]
        stop <- w856 stop-if-true
        n280 = Get Queue Status(queue=w850) -> (queue out=w858:refnum<queue>, # elements in queue=w860:i32)  [unwired: 2 in, 6 out]
        n281 = Get Notifier Status(notifier=w857) -> (current notification=w856:bool)  [unwired: 1 in, 4 out]
        n282 = Greater Than 0?(x=w860) -> (x > 0?=w859:bool)
        n283 = case shown="True" w859 {
          tunnel: w866 -> [_ w897]
          tunnel: w865 -> [w868 w898]
          tunnel: [w868 w896] -> w864
          tunnel: w863 -> [_ w894]
          tunnel: w862 -> [_ w893]
          tunnel: w861 -> [_ w883]
          tunnel: w858 -> [_ w892]
          tunnel: w855 -> [w867 w889]
          tunnel: [w867 w888] -> w854
          tunnel: w853 -> [_ w887]
          tunnel: w852 -> [_ w886]
          tunnel: w851 -> [_ w881]
          tunnel: w849 -> [_ w879]
          tunnel: w848 -> [_ w878]
          tunnel: w847 -> [_ w875]
          tunnel: w846 -> [_ w874]
          tunnel: w845 -> [_ _]
          tunnel: w844 -> [_ _]
          frame False {
          }
          frame True {
            # "False: 1st frame in fram accum"
            # "True: Last Frame of frame accum"
            # "Current Line in Frame Accum"
            # "Current Line In Frame"
            n284 = Increment(x=w889) -> (x+1=w882:u32)
            n285 = Dequeue Element(queue=w892) -> (element=w904:u64[])  [unwired: 2 in, 3 out]
            n286 = Equal?(x=w882, y=w886) -> (x = y?=w891:bool)
            n287 = Greater?(x=w882, y=w887) -> (0:w884:bool)
            n288 = Greater?(x=w882, y=w881) -> (0:w880:bool)
            n289 = Split Number(x=w904) -> (hi(x)=w905:u32[], lo(x)=w903:u32[])
            n290 = Split Number(x=w905) -> (hi(x)=w876:u16[])  [unwired: 1 out]
            n291 = Split Number(x=w903) -> (hi(x)=w902:u16[])  [unwired: 1 out]
            n292 = Select(t=u32 0, s=w891, f=w882) -> (s? t:f=w888:u32)
            n293 = Increment(x=w898) -> (x+1=w899:i32)
            n294 = Equal?(x=w897, y=w898) -> (x = y?=w869:bool)
            n295 = Select(t=0, s=w869, f=w899) -> (s? t:f=w896:i32)
            n296 = Build Array(0, w898, w897, w898) -> (w873:i32[])
            n297 = case shown="False" w880 {
              tunnel: w876 -> [w930 w945]
              tunnel: w902 -> [w927 w944]
              tunnel: [w926 w940] -> w895
              tunnel: [w929 w939] -> w871
              tunnel: w873 -> [_ w936]
              tunnel: w893 -> [w925 w934]
              tunnel: w879 -> [w924 w932]
              tunnel: w878 -> [w923 w933]
              tunnel: [w923 w933] -> w877
              tunnel: [w924 w932] -> w872
              frame False {
                n298 = To Single Precision Float(number=w930) -> (single precision float=w931:sgl[])
                n299 = To Single Precision Float(number=w927) -> (single precision float=w928:sgl[])
                n300 = Divide(x=w931, y=w925) -> (x/y=w929:sgl[])
                n301 = Divide(x=w928, y=w925) -> (x/y=w926:sgl[])
              }
              frame True {
                n302 = To Single Precision Float(number=w945) -> (single precision float=w935:sgl[])
                n303 = To Single Precision Float(number=w944) -> (single precision float=w943:sgl[])
                n304 = call "IMAQ GetPixelLine"("Line Coordinates"=w936, "Image"=w932) -> ("Pixels Line (Float)"=w938:sgl[])  [unwired: 2 in, 4 out]
                n305 = call "IMAQ GetPixelLine"("Line Coordinates"=w936, "Image"=w933) -> ("Pixels Line (Float)"=w937:sgl[])  [unwired: 2 in, 4 out]
                n306 = Divide(x=w935, y=w934) -> (x/y=w942:sgl[])
                n307 = Divide(x=w943, y=w934) -> (x/y=w941:sgl[])
                n308 = Add(x=w938, y=w942) -> (x+y=w939:sgl[])
                n309 = Add(x=w937, y=w941) -> (x+y=w940:sgl[])
              }
            }
            n310 = stacked-sequence {
              tunnel: w873 -> [w906 _]
              tunnel: w871 -> [w908 _]
              tunnel: w872 -> [w907 _]
              tunnel: w869 -> [_ w912]
              tunnel: [w906 _] -> w870
              frame #0 {
                n311 = call "IMAQ SetPixelLine"("Pixels Line (Float)"=w908, "Line Coordinates"=w906, "Image"=w907) -> ()  [unwired: 7 in, 2 out]
              }
              frame #1 {
                n312 = case shown="True" w912 {
                  tunnel: [w913 w915] -> w910
                  frame False {
                    n313 = call "Frame Counter.vi"("Action"=Counter_Action."Read") -> ("Num"=w913:i32)
                  }
                  frame True {
                    n314 = call "Frame Counter.vi"("Action"=Counter_Action."Plus One") -> ("Num"=w915:i32)
                  }
                }
                n315 = call "FPGA-7842R-Control V2.vi"("Current Frame"=w910, "Action"=FPGA-7842R-Reference."Current Frame for Capture", "Initialize"=TRUE) -> ()  [unwired: 11 in, 2 out]
              }
            }
            n316 = call "IMAQ SetPixelLine"("Pixels Line (Float)"=w895, "Line Coordinates"=w870, "Image"=w877) -> ()  [unwired: 7 in, 2 out]
            n317 = And(x=w884, y=w883) -> (x .and. y?=w885:bool)
            n318 = case shown="True" w885 {
              tunnel: w871 -> [_ w922]
              tunnel: w895 -> [_ w921]
              tunnel: w894 -> [_ w919]
              tunnel: w875 -> [_ w918]
              tunnel: w874 -> [_ w917]
              frame False {
              }
              frame True {
                w920 = FALSE ("prepend array or string size? (T)")
                n319 = Write to Binary File(file (use dialog)=w918, data=w922, 5:w920, 9:w919) -> ()  [unwired: 2 in, 3 out]
                n320 = Write to Binary File(file (use dialog)=w917, data=w921, 5:w920, 9:w919) -> ()  [unwired: 2 in, 3 out]
              }
            }
          }
        }
      }
    }
    frame 6 {
      n321 = while {
        shift-right: [w983] -> _
        shift-left: 0 -> [w984]
        tunnel: w961 -> [w985]
        tunnel: w960 -> [w982]
        tunnel: w959 -> [w981]
        tunnel: w958 -> [w980]
        tunnel: w946 -> [w976]
        shift-right: [w973] -> _
        shift-left: u32 0 -> [w974]
        tunnel: w956 -> [w972]
        tunnel: w955 -> [w971]
        tunnel: w954 -> [w970]
        tunnel: w953 -> [w969]
        tunnel: w948 -> [w968]
        tunnel: w947 -> [w967]
        tunnel: w952 -> [w966]
        tunnel: w951 -> [w965]
        tunnel: w950 -> [w964]
        tunnel: w949 -> [w963]
        stop <- w975 stop-if-true
        n322 = Get Queue Status(queue=w969) -> (queue out=w977:refnum<queue>, # elements in queue=w979:i32)  [unwired: 2 in, 6 out]
        n323 = Get Notifier Status(notifier=w976) -> (current notification=w975:bool)  [unwired: 1 in, 4 out]
        n324 = Greater Than 0?(x=w979) -> (x > 0?=w978:bool)
        n325 = case shown="True" w978 {
          tunnel: w985 -> [_ w1015]
          tunnel: w984 -> [w987 w1016]
          tunnel: [w987 w1014] -> w983
          tunnel: w982 -> [_ w1012]
          tunnel: w981 -> [_ w1011]
          tunnel: w980 -> [_ w1001]
          tunnel: w977 -> [_ w1010]
          tunnel: w974 -> [w986 w1007]
          tunnel: [w986 w1006] -> w973
          tunnel: w972 -> [_ w1005]
          tunnel: w971 -> [_ w1004]
          tunnel: w970 -> [_ w999]
          tunnel: w968 -> [_ w997]
          tunnel: w967 -> [_ w996]
          tunnel: w966 -> [_ w994]
          tunnel: w965 -> [_ w993]
          tunnel: w964 -> [_ _]
          tunnel: w963 -> [_ _]
          frame False {
          }
          frame True {
            # "False: 1st frame in fram accum"
            # "True: Last Frame of frame accum"
            # "Current Line in Frame Accum"
            # "Current Line In Frame"
            n326 = Increment(x=w1007) -> (x+1=w1000:u32)
            n327 = Dequeue Element(queue=w1010) -> (element=w1023:u64[])  [unwired: 2 in, 3 out]
            n328 = Equal?(x=w1000, y=w1004) -> (x = y?=w1009:bool)
            n329 = Greater?(x=w1000, y=w1005) -> (0:w1002:bool)
            n330 = Greater?(x=w1000, y=w999) -> (0:w998:bool)
            n331 = Split Number(x=w1023) -> (hi(x)=w1024:u32[], lo(x)=w1022:u32[])
            n332 = Split Number(x=w1024) -> (lo(x)=w1021:u16[])  [unwired: 1 out]
            n333 = Split Number(x=w1022) -> (hi(x)=w1020:u16[])  [unwired: 1 out]
            n334 = Select(t=u32 0, s=w1009, f=w1000) -> (s? t:f=w1006:u32)
            n335 = Increment(x=w1016) -> (x+1=w1017:i32)
            n336 = Equal?(x=w1015, y=w1016) -> (x = y?=w992:bool)
            n337 = Select(t=0, s=w992, f=w1017) -> (s? t:f=w1014:i32)
            n338 = Build Array(0, w1016, w1015, w1016) -> (w991:i32[])
            n339 = case shown="False" w998 {
              tunnel: w1021 -> [w1048 w1064]
              tunnel: w1020 -> [w1047 w1063]
              tunnel: [w1045 w1058] -> w1013
              tunnel: [w1046 w1057] -> w989
              tunnel: w991 -> [_ w1054]
              tunnel: w1011 -> [w1044 w1053]
              tunnel: w997 -> [w1043 w1051]
              tunnel: w996 -> [w1042 w1052]
              tunnel: [w1042 w1052] -> w995
              tunnel: [w1043 w1051] -> w990
              frame False {
                n340 = To Single Precision Float(number=w1048) -> (single precision float=w1050:sgl[])
                n341 = To Single Precision Float(number=w1047) -> (single precision float=w1049:sgl[])
                n342 = Divide(x=w1050, y=w1044) -> (x/y=w1046:sgl[])
                n343 = Divide(x=w1049, y=w1044) -> (x/y=w1045:sgl[])
              }
              frame True {
                n344 = To Single Precision Float(number=w1064) -> (single precision float=w1062:sgl[])
                n345 = To Single Precision Float(number=w1063) -> (single precision float=w1061:sgl[])
                n346 = call "IMAQ GetPixelLine"("Line Coordinates"=w1054, "Image"=w1051) -> ("Pixels Line (Float)"=w1056:sgl[])  [unwired: 2 in, 4 out]
                n347 = call "IMAQ GetPixelLine"("Line Coordinates"=w1054, "Image"=w1052) -> ("Pixels Line (Float)"=w1055:sgl[])  [unwired: 2 in, 4 out]
                n348 = Divide(x=w1062, y=w1053) -> (x/y=w1060:sgl[])
                n349 = Divide(x=w1061, y=w1053) -> (x/y=w1059:sgl[])
                n350 = Add(x=w1056, y=w1060) -> (x+y=w1057:sgl[])
                n351 = Add(x=w1055, y=w1059) -> (x+y=w1058:sgl[])
              }
            }
            n352 = stacked-sequence {
              tunnel: w991 -> [w1025 _]
              tunnel: w989 -> [w1027 _]
              tunnel: w990 -> [w1026 _]
              tunnel: w992 -> [_ w1031]
              tunnel: [w1025 _] -> w988
              frame #0 {
                n353 = call "IMAQ SetPixelLine"("Pixels Line (Float)"=w1027, "Line Coordinates"=w1025, "Image"=w1026) -> ()  [unwired: 7 in, 2 out]
              }
              frame #1 {
                n354 = case shown="True" w1031 {
                  tunnel: [w1032 w1034] -> w1029
                  frame False {
                    n355 = call "Frame Counter.vi"("Action"=Counter_Action."Read") -> ("Num"=w1032:i32)
                  }
                  frame True {
                    n356 = call "Frame Counter.vi"("Action"=Counter_Action."Plus One") -> ("Num"=w1034:i32)
                  }
                }
                n357 = call "FPGA-7842R-Control V2.vi"("Current Frame"=w1029, "Action"=FPGA-7842R-Reference."Current Frame for Capture", "Initialize"=TRUE) -> ()  [unwired: 11 in, 2 out]
              }
            }
            n358 = call "IMAQ SetPixelLine"("Pixels Line (Float)"=w1013, "Line Coordinates"=w988, "Image"=w995) -> ()  [unwired: 7 in, 2 out]
            n359 = And(x=w1002, y=w1001) -> (x .and. y?=w1003:bool)
            n360 = case shown="True" w1003 {
              tunnel: w989 -> [_ w1041]
              tunnel: w1013 -> [_ w1040]
              tunnel: w1012 -> [_ w1038]
              tunnel: w994 -> [_ w1037]
              tunnel: w993 -> [_ w1036]
              frame False {
              }
              frame True {
                w1039 = FALSE ("prepend array or string size? (T)")
                n361 = Write to Binary File(file (use dialog)=w1037, data=w1041, 5:w1039, 9:w1038) -> ()  [unwired: 2 in, 3 out]
                n362 = Write to Binary File(file (use dialog)=w1036, data=w1040, 5:w1039, 9:w1038) -> ()  [unwired: 2 in, 3 out]
              }
            }
          }
        }
      }
    }
    frame 7 {
      n363 = while {
        shift-right: [w1104] -> _
        shift-left: 0 -> [w1105]
        tunnel: w1081 -> [w1106]
        tunnel: w1080 -> [w1103]
        tunnel: w1079 -> [w1102]
        tunnel: w1078 -> [w1101]
        tunnel: w1065 -> [w1097]
        shift-right: [w1094] -> _
        shift-left: u32 0 -> [w1095]
        tunnel: w1076 -> [w1093]
        tunnel: w1075 -> [w1092]
        tunnel: w1074 -> [w1091]
        tunnel: w1073 -> [w1090]
        tunnel: w1068 -> [w1089]
        tunnel: w1067 -> [w1088]
        tunnel: w1066 -> [w1087]
        tunnel: w1072 -> [w1086]
        tunnel: w1071 -> [w1085]
        tunnel: w1070 -> [w1084]
        tunnel: w1069 -> [w1083]
        stop <- w1096 stop-if-true
        n364 = Get Queue Status(queue=w1090) -> (queue out=w1098:refnum<queue>, # elements in queue=w1100:i32)  [unwired: 2 in, 6 out]
        n365 = Get Notifier Status(notifier=w1097) -> (current notification=w1096:bool)  [unwired: 1 in, 4 out]
        n366 = Greater Than 0?(x=w1100) -> (x > 0?=w1099:bool)
        n367 = case shown="True" w1099 {
          tunnel: w1106 -> [_ w1141]
          tunnel: w1105 -> [w1108 w1142]
          tunnel: [w1108 w1140] -> w1104
          tunnel: w1103 -> [_ w1137]
          tunnel: w1102 -> [_ w1136]
          tunnel: w1101 -> [_ w1126]
          tunnel: w1098 -> [_ w1135]
          tunnel: w1095 -> [w1107 w1132]
          tunnel: [w1107 w1131] -> w1094
          tunnel: w1093 -> [_ w1130]
          tunnel: w1092 -> [_ w1129]
          tunnel: w1091 -> [_ w1124]
          tunnel: w1089 -> [_ w1122]
          tunnel: w1088 -> [_ w1121]
          tunnel: w1087 -> [_ w1120]
          tunnel: w1086 -> [_ w1116]
          tunnel: w1085 -> [_ w1115]
          tunnel: w1084 -> [_ w1114]
          tunnel: w1083 -> [_ _]
          frame False {
          }
          frame True {
            # "False: 1st frame in fram accum"
            # "True: Last Frame of frame accum"
            # "Current Line in Frame Accum"
            # "Current Line In Frame"
            n368 = Increment(x=w1132) -> (x+1=w1125:u32)
            n369 = Dequeue Element(queue=w1135) -> (element=w1149:u64[])  [unwired: 2 in, 3 out]
            n370 = Equal?(x=w1125, y=w1129) -> (x = y?=w1134:bool)
            n371 = Greater?(x=w1125, y=w1130) -> (0:w1127:bool)
            n372 = Greater?(x=w1125, y=w1124) -> (0:w1123:bool)
            n373 = Split Number(x=w1149) -> (hi(x)=w1150:u32[], lo(x)=w1148:u32[])
            n374 = Split Number(x=w1150) -> (hi(x)=w1117:u16[], lo(x)=w1147:u16[])
            n375 = Split Number(x=w1148) -> (hi(x)=w1146:u16[])  [unwired: 1 out]
            n376 = Select(t=u32 0, s=w1134, f=w1125) -> (s? t:f=w1131:u32)
            n377 = Increment(x=w1142) -> (x+1=w1143:i32)
            n378 = Equal?(x=w1141, y=w1142) -> (x = y?=w1113:bool)
            n379 = Select(t=0, s=w1113, f=w1143) -> (s? t:f=w1140:i32)
            n380 = Build Array(0, w1142, w1141, w1142) -> (w1112:i32[])
            n381 = case shown="False" w1123 {
              tunnel: w1117 -> [w1181 w1202]
              tunnel: w1147 -> [w1177 w1201]
              tunnel: w1146 -> [w1176 w1200]
              tunnel: [w1174 w1194] -> w1138
              tunnel: [w1175 w1193] -> w1139
              tunnel: [w1180 w1192] -> w1110
              tunnel: w1112 -> [_ w1188]
              tunnel: w1136 -> [w1173 w1186]
              tunnel: w1122 -> [w1172 w1183]
              tunnel: w1121 -> [w1171 w1184]
              tunnel: w1120 -> [w1170 w1185]
              tunnel: [w1170 w1185] -> w1118
              tunnel: [w1171 w1184] -> w1119
              tunnel: [w1172 w1183] -> w1111
              frame False {
                n382 = To Single Precision Float(number=w1181) -> (single precision float=w1182:sgl[])
                n383 = To Single Precision Float(number=w1177) -> (single precision float=w1179:sgl[])
                n384 = To Single Precision Float(number=w1176) -> (single precision float=w1178:sgl[])
                n385 = Divide(x=w1182, y=w1173) -> (x/y=w1180:sgl[])
                n386 = Divide(x=w1179, y=w1173) -> (x/y=w1175:sgl[])
                n387 = Divide(x=w1178, y=w1173) -> (x/y=w1174:sgl[])
              }
              frame True {
                n388 = To Single Precision Float(number=w1202) -> (single precision float=w1187:sgl[])
                n389 = To Single Precision Float(number=w1201) -> (single precision float=w1199:sgl[])
                n390 = To Single Precision Float(number=w1200) -> (single precision float=w1198:sgl[])
                n391 = call "IMAQ GetPixelLine"("Line Coordinates"=w1188, "Image"=w1183) -> ("Pixels Line (Float)"=w1191:sgl[])  [unwired: 2 in, 4 out]
                n392 = call "IMAQ GetPixelLine"("Line Coordinates"=w1188, "Image"=w1184) -> ("Pixels Line (Float)"=w1190:sgl[])  [unwired: 2 in, 4 out]
                n393 = call "IMAQ GetPixelLine"("Line Coordinates"=w1188, "Image"=w1185) -> ("Pixels Line (Float)"=w1189:sgl[])  [unwired: 2 in, 4 out]
                n394 = Divide(x=w1187, y=w1186) -> (x/y=w1197:sgl[])
                n395 = Divide(x=w1199, y=w1186) -> (x/y=w1196:sgl[])
                n396 = Divide(x=w1198, y=w1186) -> (x/y=w1195:sgl[])
                n397 = Add(x=w1191, y=w1197) -> (x+y=w1192:sgl[])
                n398 = Add(x=w1190, y=w1196) -> (x+y=w1193:sgl[])
                n399 = Add(x=w1189, y=w1195) -> (x+y=w1194:sgl[])
              }
            }
            n400 = stacked-sequence {
              tunnel: w1112 -> [w1151 _]
              tunnel: w1110 -> [w1153 _]
              tunnel: w1111 -> [w1152 _]
              tunnel: w1113 -> [_ w1157]
              tunnel: [w1151 _] -> w1109
              frame #0 {
                n401 = call "IMAQ SetPixelLine"("Pixels Line (Float)"=w1153, "Line Coordinates"=w1151, "Image"=w1152) -> ()  [unwired: 7 in, 2 out]
              }
              frame #1 {
                n402 = case shown="True" w1157 {
                  tunnel: [w1158 w1160] -> w1155
                  frame False {
                    n403 = call "Frame Counter.vi"("Action"=Counter_Action."Read") -> ("Num"=w1158:i32)
                  }
                  frame True {
                    n404 = call "Frame Counter.vi"("Action"=Counter_Action."Plus One") -> ("Num"=w1160:i32)
                  }
                }
                n405 = call "FPGA-7842R-Control V2.vi"("Current Frame"=w1155, "Action"=FPGA-7842R-Reference."Current Frame for Capture", "Initialize"=TRUE) -> ()  [unwired: 11 in, 2 out]
              }
            }
            n406 = call "IMAQ SetPixelLine"("Pixels Line (Float)"=w1139, "Line Coordinates"=w1109, "Image"=w1119) -> ()  [unwired: 7 in, 2 out]
            n407 = call "IMAQ SetPixelLine"("Pixels Line (Float)"=w1138, "Line Coordinates"=w1109, "Image"=w1118) -> ()  [unwired: 7 in, 2 out]
            n408 = And(x=w1127, y=w1126) -> (x .and. y?=w1128:bool)
            n409 = case shown="True" w1128 {
              tunnel: w1110 -> [_ w1169]
              tunnel: w1139 -> [_ w1168]
              tunnel: w1138 -> [_ w1167]
              tunnel: w1137 -> [_ w1165]
              tunnel: w1116 -> [_ w1164]
              tunnel: w1115 -> [_ w1163]
              tunnel: w1114 -> [_ w1162]
              frame False {
              }
              frame True {
                w1166 = FALSE ("prepend array or string size? (T)")
                n410 = Write to Binary File(file (use dialog)=w1164, data=w1169, 5:w1166, 9:w1165) -> ()  [unwired: 2 in, 3 out]
                n411 = Write to Binary File(file (use dialog)=w1163, data=w1168, 5:w1166, 9:w1165) -> ()  [unwired: 2 in, 3 out]
                n412 = Write to Binary File(file (use dialog)=w1162, data=w1167, 5:w1166, 9:w1165) -> ()  [unwired: 2 in, 3 out]
              }
            }
          }
        }
      }
    }
    frame 8, 24 {
      n413 = while {
        shift-right: [w1238] -> _
        shift-left: 0 -> [w1239]
        tunnel: w1217 -> [w1240]
        tunnel: w1216 -> [w1237]
        tunnel: w1215 -> [w1236]
        tunnel: w1214 -> [w1235]
        tunnel: w1203 -> [w1231]
        shift-right: [w1228] -> _
        shift-left: u32 0 -> [w1229]
        tunnel: w1212 -> [w1227]
        tunnel: w1211 -> [w1226]
        tunnel: w1210 -> [w1225]
        tunnel: w1209 -> [w1224]
        tunnel: w1204 -> [w1223]
        tunnel: w1208 -> [w1222]
        tunnel: w1207 -> [w1221]
        tunnel: w1206 -> [w1220]
        tunnel: w1205 -> [w1219]
        stop <- w1230 stop-if-true
        n414 = Get Queue Status(queue=w1224) -> (queue out=w1232:refnum<queue>, # elements in queue=w1234:i32)  [unwired: 2 in, 6 out]
        n415 = Get Notifier Status(notifier=w1231) -> (current notification=w1230:bool)  [unwired: 1 in, 4 out]
        n416 = Greater Than 0?(x=w1234) -> (x > 0?=w1233:bool)
        n417 = case shown="True" w1233 {
          tunnel: w1240 -> [_ w1265]
          tunnel: w1239 -> [w1242 w1266]
          tunnel: [w1242 w1264] -> w1238
          tunnel: w1237 -> [_ w1263]
          tunnel: w1236 -> [_ w1262]
          tunnel: w1235 -> [_ w1252]
          tunnel: w1232 -> [_ w1261]
          tunnel: w1229 -> [w1241 w1258]
          tunnel: [w1241 w1257] -> w1228
          tunnel: w1227 -> [_ w1256]
          tunnel: w1226 -> [_ w1255]
          tunnel: w1225 -> [_ w1250]
          tunnel: w1223 -> [_ w1248]
          tunnel: w1222 -> [_ w1247]
          tunnel: w1221 -> [_ _]
          tunnel: w1220 -> [_ _]
          tunnel: w1219 -> [_ _]
          frame False {
          }
          frame True {
            # "False: 1st frame in fram accum"
            # "True: Last Frame of frame accum"
            # "Current Line in Frame Accum"
            # "Current Line In Frame"
            n418 = Increment(x=w1258) -> (x+1=w1251:u32)
            n419 = Dequeue Element(queue=w1261) -> (element=w1272:u64[])  [unwired: 2 in, 3 out]
            n420 = Equal?(x=w1251, y=w1255) -> (x = y?=w1260:bool)
            n421 = Greater?(x=w1251, y=w1256) -> (0:w1253:bool)
            n422 = Greater?(x=w1251, y=w1250) -> (0:w1249:bool)
            n423 = Split Number(x=w1272) -> (lo(x)=w1271:u32[])  [unwired: 1 out]
            n424 = Split Number(x=w1271) -> (lo(x)=w1270:u16[])  [unwired: 1 out]
            n425 = Select(t=u32 0, s=w1260, f=w1251) -> (s? t:f=w1257:u32)
            n426 = Increment(x=w1266) -> (x+1=w1267:i32)
            n427 = Equal?(x=w1265, y=w1266) -> (x = y?=w1246:bool)
            n428 = Select(t=0, s=w1246, f=w1267) -> (s? t:f=w1264:i32)
            n429 = Build Array(0, w1266, w1265, w1266) -> (w1245:i32[])
            n430 = case shown="True" w1249 {
              tunnel: w1270 -> [w1291 w1300]
              tunnel: [w1290 w1297] -> w1243
              tunnel: w1245 -> [_ w1295]
              tunnel: w1262 -> [w1289 w1294]
              tunnel: w1248 -> [w1288 w1293]
              tunnel: [w1288 w1293] -> w1244
              frame False {
                n431 = To Single Precision Float(number=w1291) -> (single precision float=w1292:sgl[])
                n432 = Divide(x=w1292, y=w1289) -> (x/y=w1290:sgl[])
              }
              frame True {
                n433 = To Single Precision Float(number=w1300) -> (single precision float=w1299:sgl[])
                n434 = call "IMAQ GetPixelLine"("Line Coordinates"=w1295, "Image"=w1293) -> ("Pixels Line (Float)"=w1296:sgl[])  [unwired: 2 in, 4 out]
                n435 = Divide(x=w1299, y=w1294) -> (x/y=w1298:sgl[])
                n436 = Add(x=w1296, y=w1298) -> (x+y=w1297:sgl[])
              }
            }
            n437 = stacked-sequence {
              tunnel: w1245 -> [w1275 _]
              tunnel: w1243 -> [w1274 _]
              tunnel: w1244 -> [w1273 _]
              tunnel: w1246 -> [_ w1279]
              frame #0 {
                n438 = call "IMAQ SetPixelLine"("Pixels Line (Float)"=w1274, "Line Coordinates"=w1275, "Image"=w1273) -> ()  [unwired: 7 in, 2 out]
              }
              frame #1 {
                n439 = case shown="True" w1279 {
                  tunnel: [w1280 w1282] -> w1277
                  frame False {
                    n440 = call "Frame Counter.vi"("Action"=Counter_Action."Read") -> ("Num"=w1280:i32)
                  }
                  frame True {
                    n441 = call "Frame Counter.vi"("Action"=Counter_Action."Plus One") -> ("Num"=w1282:i32)
                  }
                }
                n442 = call "FPGA-7842R-Control V2.vi"("Current Frame"=w1277, "Action"=FPGA-7842R-Reference."Current Frame for Capture", "Initialize"=TRUE) -> ()  [unwired: 11 in, 2 out]
              }
            }
            n443 = And(x=w1253, y=w1252) -> (x .and. y?=w1254:bool)
            n444 = case shown="True" w1254 {
              tunnel: w1243 -> [_ w1287]
              tunnel: w1263 -> [_ w1285]
              tunnel: w1247 -> [_ w1284]
              frame False {
              }
              frame True {
                n445 = Write to Binary File(file (use dialog)=w1284, data=w1287, 5:FALSE ("prepend array or string size? (T)"), 9:w1285) -> ()  [unwired: 2 in, 3 out]
              }
            }
          }
        }
      }
    }
    frame 9 {
      n446 = while {
        shift-right: [w1338] -> _
        shift-left: 0 -> [w1339]
        tunnel: w1316 -> [w1340]
        tunnel: w1315 -> [w1337]
        tunnel: w1314 -> [w1336]
        tunnel: w1313 -> [w1335]
        tunnel: w1301 -> [w1331]
        shift-right: [w1328] -> _
        shift-left: u32 0 -> [w1329]
        tunnel: w1311 -> [w1327]
        tunnel: w1310 -> [w1326]
        tunnel: w1309 -> [w1325]
        tunnel: w1308 -> [w1324]
        tunnel: w1303 -> [w1323]
        tunnel: w1302 -> [w1322]
        tunnel: w1307 -> [w1321]
        tunnel: w1306 -> [w1320]
        tunnel: w1305 -> [w1319]
        tunnel: w1304 -> [w1318]
        stop <- w1330 stop-if-true
        n447 = Get Queue Status(queue=w1324) -> (queue out=w1332:refnum<queue>, # elements in queue=w1334:i32)  [unwired: 2 in, 6 out]
        n448 = Get Notifier Status(notifier=w1331) -> (current notification=w1330:bool)  [unwired: 1 in, 4 out]
        n449 = Greater Than 0?(x=w1334) -> (x > 0?=w1333:bool)
        n450 = case shown="True" w1333 {
          tunnel: w1340 -> [_ w1371]
          tunnel: w1339 -> [w1342 w1372]
          tunnel: [w1342 w1370] -> w1338
          tunnel: w1337 -> [_ w1368]
          tunnel: w1336 -> [_ w1367]
          tunnel: w1335 -> [_ w1357]
          tunnel: w1332 -> [_ w1366]
          tunnel: w1329 -> [w1341 w1363]
          tunnel: [w1341 w1362] -> w1328
          tunnel: w1327 -> [_ w1361]
          tunnel: w1326 -> [_ w1360]
          tunnel: w1325 -> [_ w1355]
          tunnel: w1323 -> [_ w1353]
          tunnel: w1322 -> [_ w1352]
          tunnel: w1321 -> [_ w1349]
          tunnel: w1320 -> [_ w1348]
          tunnel: w1319 -> [_ _]
          tunnel: w1318 -> [_ _]
          frame False {
          }
          frame True {
            # "False: 1st frame in fram accum"
            # "True: Last Frame of frame accum"
            # "Current Line in Frame Accum"
            # "Current Line In Frame"
            n451 = Increment(x=w1363) -> (x+1=w1356:u32)
            n452 = Dequeue Element(queue=w1366) -> (element=w1378:u64[])  [unwired: 2 in, 3 out]
            n453 = Equal?(x=w1356, y=w1360) -> (x = y?=w1365:bool)
            n454 = Greater?(x=w1356, y=w1361) -> (0:w1358:bool)
            n455 = Greater?(x=w1356, y=w1355) -> (0:w1354:bool)
            n456 = Split Number(x=w1378) -> (hi(x)=w1379:u32[], lo(x)=w1377:u32[])
            n457 = Split Number(x=w1379) -> (hi(x)=w1350:u16[])  [unwired: 1 out]
            n458 = Split Number(x=w1377) -> (lo(x)=w1376:u16[])  [unwired: 1 out]
            n459 = Select(t=u32 0, s=w1365, f=w1356) -> (s? t:f=w1362:u32)
            n460 = Increment(x=w1372) -> (x+1=w1373:i32)
            n461 = Equal?(x=w1371, y=w1372) -> (x = y?=w1347:bool)
            n462 = Select(t=0, s=w1347, f=w1373) -> (s? t:f=w1370:i32)
            n463 = Build Array(0, w1372, w1371, w1372) -> (w1344:i32[])
            n464 = case shown="True" w1354 {
              tunnel: w1350 -> [w1404 w1419]
              tunnel: w1376 -> [w1401 w1418]
              tunnel: [w1403 w1414] -> w1345
              tunnel: [w1400 w1413] -> w1369
              tunnel: w1344 -> [_ w1410]
              tunnel: w1367 -> [w1399 w1408]
              tunnel: w1353 -> [w1398 w1407]
              tunnel: w1352 -> [w1397 w1406]
              tunnel: [w1398 w1407] -> w1346
              tunnel: [w1397 w1406] -> w1351
              frame False {
                n465 = To Single Precision Float(number=w1404) -> (single precision float=w1405:sgl[])
                n466 = To Single Precision Float(number=w1401) -> (single precision float=w1402:sgl[])
                n467 = Divide(x=w1405, y=w1399) -> (x/y=w1403:sgl[])
                n468 = Divide(x=w1402, y=w1399) -> (x/y=w1400:sgl[])
              }
              frame True {
                n469 = To Single Precision Float(number=w1419) -> (single precision float=w1409:sgl[])
                n470 = To Single Precision Float(number=w1418) -> (single precision float=w1417:sgl[])
                n471 = call "IMAQ GetPixelLine"("Line Coordinates"=w1410, "Image"=w1407) -> ("Pixels Line (Float)"=w1412:sgl[])  [unwired: 2 in, 4 out]
                n472 = call "IMAQ GetPixelLine"("Line Coordinates"=w1410, "Image"=w1406) -> ("Pixels Line (Float)"=w1411:sgl[])  [unwired: 2 in, 4 out]
                n473 = Divide(x=w1409, y=w1408) -> (x/y=w1416:sgl[])
                n474 = Divide(x=w1417, y=w1408) -> (x/y=w1415:sgl[])
                n475 = Add(x=w1412, y=w1416) -> (x+y=w1414:sgl[])
                n476 = Add(x=w1411, y=w1415) -> (x+y=w1413:sgl[])
              }
            }
            n477 = stacked-sequence {
              tunnel: w1344 -> [w1380 _]
              tunnel: w1345 -> [w1382 _]
              tunnel: w1346 -> [w1381 _]
              tunnel: w1347 -> [_ w1386]
              tunnel: [w1380 _] -> w1343
              frame #0 {
                n478 = call "IMAQ SetPixelLine"("Pixels Line (Float)"=w1382, "Line Coordinates"=w1380, "Image"=w1381) -> ()  [unwired: 7 in, 2 out]
              }
              frame #1 {
                n479 = case shown="True" w1386 {
                  tunnel: [w1387 w1389] -> w1384
                  frame False {
                    n480 = call "Frame Counter.vi"("Action"=Counter_Action."Read") -> ("Num"=w1387:i32)
                  }
                  frame True {
                    n481 = call "Frame Counter.vi"("Action"=Counter_Action."Plus One") -> ("Num"=w1389:i32)
                  }
                }
                n482 = call "FPGA-7842R-Control V2.vi"("Current Frame"=w1384, "Action"=FPGA-7842R-Reference."Current Frame for Capture", "Initialize"=TRUE) -> ()  [unwired: 11 in, 2 out]
              }
            }
            n483 = call "IMAQ SetPixelLine"("Pixels Line (Float)"=w1369, "Line Coordinates"=w1343, "Image"=w1351) -> ()  [unwired: 7 in, 2 out]
            n484 = And(x=w1358, y=w1357) -> (x .and. y?=w1359:bool)
            n485 = case shown="True" w1359 {
              tunnel: w1345 -> [_ w1396]
              tunnel: w1369 -> [_ w1395]
              tunnel: w1368 -> [_ w1393]
              tunnel: w1349 -> [_ w1392]
              tunnel: w1348 -> [_ w1391]
              frame False {
              }
              frame True {
                w1394 = FALSE ("prepend array or string size? (T)")
                n486 = Write to Binary File(file (use dialog)=w1392, data=w1396, 5:w1394, 9:w1393) -> ()  [unwired: 2 in, 3 out]
                n487 = Write to Binary File(file (use dialog)=w1391, data=w1395, 5:w1394, 9:w1393) -> ()  [unwired: 2 in, 3 out]
              }
            }
          }
        }
      }
    }
    frame 10 {
      n488 = while {
        shift-right: [w1457] -> _
        shift-left: 0 -> [w1458]
        tunnel: w1435 -> [w1459]
        tunnel: w1434 -> [w1456]
        tunnel: w1433 -> [w1455]
        tunnel: w1432 -> [w1454]
        tunnel: w1420 -> [w1450]
        shift-right: [w1447] -> _
        shift-left: u32 0 -> [w1448]
        tunnel: w1430 -> [w1446]
        tunnel: w1429 -> [w1445]
        tunnel: w1428 -> [w1444]
        tunnel: w1427 -> [w1443]
        tunnel: w1422 -> [w1442]
        tunnel: w1421 -> [w1441]
        tunnel: w1426 -> [w1440]
        tunnel: w1425 -> [w1439]
        tunnel: w1424 -> [w1438]
        tunnel: w1423 -> [w1437]
        stop <- w1449 stop-if-true
        n489 = Get Queue Status(queue=w1443) -> (queue out=w1451:refnum<queue>, # elements in queue=w1453:i32)  [unwired: 2 in, 6 out]
        n490 = Get Notifier Status(notifier=w1450) -> (current notification=w1449:bool)  [unwired: 1 in, 4 out]
        n491 = Greater Than 0?(x=w1453) -> (x > 0?=w1452:bool)
        n492 = case shown="True" w1452 {
          tunnel: w1459 -> [_ w1489]
          tunnel: w1458 -> [w1461 w1490]
          tunnel: [w1461 w1488] -> w1457
          tunnel: w1456 -> [_ w1486]
          tunnel: w1455 -> [_ w1485]
          tunnel: w1454 -> [_ w1475]
          tunnel: w1451 -> [_ w1484]
          tunnel: w1448 -> [w1460 w1481]
          tunnel: [w1460 w1480] -> w1447
          tunnel: w1446 -> [_ w1479]
          tunnel: w1445 -> [_ w1478]
          tunnel: w1444 -> [_ w1473]
          tunnel: w1442 -> [_ w1471]
          tunnel: w1441 -> [_ w1470]
          tunnel: w1440 -> [_ w1468]
          tunnel: w1439 -> [_ w1467]
          tunnel: w1438 -> [_ _]
          tunnel: w1437 -> [_ _]
          frame False {
          }
          frame True {
            # "False: 1st frame in fram accum"
            # "True: Last Frame of frame accum"
            # "Current Line in Frame Accum"
            # "Current Line In Frame"
            n493 = Increment(x=w1481) -> (x+1=w1474:u32)
            n494 = Dequeue Element(queue=w1484) -> (element=w1497:u64[])  [unwired: 2 in, 3 out]
            n495 = Equal?(x=w1474, y=w1478) -> (x = y?=w1483:bool)
            n496 = Greater?(x=w1474, y=w1479) -> (0:w1476:bool)
            n497 = Greater?(x=w1474, y=w1473) -> (0:w1472:bool)
            n498 = Split Number(x=w1497) -> (hi(x)=w1498:u32[], lo(x)=w1496:u32[])
            n499 = Split Number(x=w1498) -> (lo(x)=w1495:u16[])  [unwired: 1 out]
            n500 = Split Number(x=w1496) -> (lo(x)=w1494:u16[])  [unwired: 1 out]
            n501 = Select(t=u32 0, s=w1483, f=w1474) -> (s? t:f=w1480:u32)
            n502 = Increment(x=w1490) -> (x+1=w1491:i32)
            n503 = Equal?(x=w1489, y=w1490) -> (x = y?=w1466:bool)
            n504 = Select(t=0, s=w1466, f=w1491) -> (s? t:f=w1488:i32)
            n505 = Build Array(0, w1490, w1489, w1490) -> (w1465:i32[])
            n506 = case shown="True" w1472 {
              tunnel: w1495 -> [w1522 w1538]
              tunnel: w1494 -> [w1521 w1537]
              tunnel: [w1520 w1532] -> w1462
              tunnel: [w1519 w1531] -> w1487
              tunnel: w1465 -> [_ w1528]
              tunnel: w1485 -> [w1518 w1527]
              tunnel: w1471 -> [w1517 w1526]
              tunnel: w1470 -> [w1516 w1525]
              tunnel: [w1517 w1526] -> w1464
              tunnel: [w1516 w1525] -> w1469
              frame False {
                n507 = To Single Precision Float(number=w1522) -> (single precision float=w1524:sgl[])
                n508 = To Single Precision Float(number=w1521) -> (single precision float=w1523:sgl[])
                n509 = Divide(x=w1524, y=w1518) -> (x/y=w1520:sgl[])
                n510 = Divide(x=w1523, y=w1518) -> (x/y=w1519:sgl[])
              }
              frame True {
                n511 = To Single Precision Float(number=w1538) -> (single precision float=w1536:sgl[])
                n512 = To Single Precision Float(number=w1537) -> (single precision float=w1535:sgl[])
                n513 = call "IMAQ GetPixelLine"("Line Coordinates"=w1528, "Image"=w1526) -> ("Pixels Line (Float)"=w1530:sgl[])  [unwired: 2 in, 4 out]
                n514 = call "IMAQ GetPixelLine"("Line Coordinates"=w1528, "Image"=w1525) -> ("Pixels Line (Float)"=w1529:sgl[])  [unwired: 2 in, 4 out]
                n515 = Divide(x=w1536, y=w1527) -> (x/y=w1534:sgl[])
                n516 = Divide(x=w1535, y=w1527) -> (x/y=w1533:sgl[])
                n517 = Add(x=w1530, y=w1534) -> (x+y=w1532:sgl[])
                n518 = Add(x=w1529, y=w1533) -> (x+y=w1531:sgl[])
              }
            }
            n519 = stacked-sequence {
              tunnel: w1465 -> [w1499 _]
              tunnel: w1462 -> [w1501 _]
              tunnel: w1464 -> [w1500 _]
              tunnel: w1466 -> [_ w1505]
              tunnel: [w1499 _] -> w1463
              frame #0 {
                n520 = call "IMAQ SetPixelLine"("Pixels Line (Float)"=w1501, "Line Coordinates"=w1499, "Image"=w1500) -> ()  [unwired: 7 in, 2 out]
              }
              frame #1 {
                n521 = case shown="True" w1505 {
                  tunnel: [w1506 w1508] -> w1503
                  frame False {
                    n522 = call "Frame Counter.vi"("Action"=Counter_Action."Read") -> ("Num"=w1506:i32)
                  }
                  frame True {
                    n523 = call "Frame Counter.vi"("Action"=Counter_Action."Plus One") -> ("Num"=w1508:i32)
                  }
                }
                n524 = call "FPGA-7842R-Control V2.vi"("Current Frame"=w1503, "Action"=FPGA-7842R-Reference."Current Frame for Capture", "Initialize"=TRUE) -> ()  [unwired: 11 in, 2 out]
              }
            }
            n525 = call "IMAQ SetPixelLine"("Pixels Line (Float)"=w1487, "Line Coordinates"=w1463, "Image"=w1469) -> ()  [unwired: 7 in, 2 out]
            n526 = And(x=w1476, y=w1475) -> (x .and. y?=w1477:bool)
            n527 = case shown="True" w1477 {
              tunnel: w1462 -> [_ w1515]
              tunnel: w1487 -> [_ w1514]
              tunnel: w1486 -> [_ w1512]
              tunnel: w1468 -> [_ w1511]
              tunnel: w1467 -> [_ w1510]
              frame False {
              }
              frame True {
                w1513 = FALSE ("prepend array or string size? (T)")
                n528 = Write to Binary File(file (use dialog)=w1511, data=w1515, 5:w1513, 9:w1512) -> ()  [unwired: 2 in, 3 out]
                n529 = Write to Binary File(file (use dialog)=w1510, data=w1514, 5:w1513, 9:w1512) -> ()  [unwired: 2 in, 3 out]
              }
            }
          }
        }
      }
    }
    frame 11 {
      n530 = while {
        shift-right: [w1578] -> _
        shift-left: 0 -> [w1579]
        tunnel: w1555 -> [w1580]
        tunnel: w1554 -> [w1577]
        tunnel: w1553 -> [w1576]
        tunnel: w1552 -> [w1575]
        tunnel: w1539 -> [w1571]
        shift-right: [w1568] -> _
        shift-left: u32 0 -> [w1569]
        tunnel: w1550 -> [w1567]
        tunnel: w1549 -> [w1566]
        tunnel: w1548 -> [w1565]
        tunnel: w1547 -> [w1564]
        tunnel: w1542 -> [w1563]
        tunnel: w1541 -> [w1562]
        tunnel: w1540 -> [w1561]
        tunnel: w1546 -> [w1560]
        tunnel: w1545 -> [w1559]
        tunnel: w1544 -> [w1558]
        tunnel: w1543 -> [w1557]
        stop <- w1570 stop-if-true
        n531 = Get Queue Status(queue=w1564) -> (queue out=w1572:refnum<queue>, # elements in queue=w1574:i32)  [unwired: 2 in, 6 out]
        n532 = Get Notifier Status(notifier=w1571) -> (current notification=w1570:bool)  [unwired: 1 in, 4 out]
        n533 = Greater Than 0?(x=w1574) -> (x > 0?=w1573:bool)
        n534 = case shown="True" w1573 {
          tunnel: w1580 -> [_ w1615]
          tunnel: w1579 -> [w1582 w1616]
          tunnel: [w1582 w1614] -> w1578
          tunnel: w1577 -> [_ w1611]
          tunnel: w1576 -> [_ w1610]
          tunnel: w1575 -> [_ w1600]
          tunnel: w1572 -> [_ w1609]
          tunnel: w1569 -> [w1581 w1606]
          tunnel: [w1581 w1605] -> w1568
          tunnel: w1567 -> [_ w1604]
          tunnel: w1566 -> [_ w1603]
          tunnel: w1565 -> [_ w1598]
          tunnel: w1563 -> [_ w1596]
          tunnel: w1562 -> [_ w1595]
          tunnel: w1561 -> [_ w1594]
          tunnel: w1560 -> [_ w1590]
          tunnel: w1559 -> [_ w1589]
          tunnel: w1558 -> [_ w1588]
          tunnel: w1557 -> [_ _]
          frame False {
          }
          frame True {
            # "False: 1st frame in fram accum"
            # "True: Last Frame of frame accum"
            # "Current Line in Frame Accum"
            # "Current Line In Frame"
            n535 = Increment(x=w1606) -> (x+1=w1599:u32)
            n536 = Dequeue Element(queue=w1609) -> (element=w1623:u64[])  [unwired: 2 in, 3 out]
            n537 = Equal?(x=w1599, y=w1603) -> (x = y?=w1608:bool)
            n538 = Greater?(x=w1599, y=w1604) -> (0:w1601:bool)
            n539 = Greater?(x=w1599, y=w1598) -> (0:w1597:bool)
            n540 = Split Number(x=w1623) -> (hi(x)=w1624:u32[], lo(x)=w1622:u32[])
            n541 = Split Number(x=w1624) -> (hi(x)=w1591:u16[], lo(x)=w1621:u16[])
            n542 = Split Number(x=w1622) -> (lo(x)=w1620:u16[])  [unwired: 1 out]
            n543 = Select(t=u32 0, s=w1608, f=w1599) -> (s? t:f=w1605:u32)
            n544 = Increment(x=w1616) -> (x+1=w1617:i32)
            n545 = Equal?(x=w1615, y=w1616) -> (x = y?=w1587:bool)
            n546 = Select(t=0, s=w1587, f=w1617) -> (s? t:f=w1614:i32)
            n547 = Build Array(0, w1616, w1615, w1616) -> (w1585:i32[])
            n548 = case shown="False" w1597 {
              tunnel: w1591 -> [w1655 w1676]
              tunnel: w1621 -> [w1651 w1675]
              tunnel: w1620 -> [w1650 w1674]
              tunnel: [w1649 w1668] -> w1613
              tunnel: [w1654 w1667] -> w1583
              tunnel: [w1648 w1666] -> w1612
              tunnel: w1585 -> [_ w1662]
              tunnel: w1610 -> [w1647 w1660]
              tunnel: w1596 -> [w1646 w1658]
              tunnel: w1595 -> [w1645 w1659]
              tunnel: w1594 -> [w1644 w1657]
              tunnel: [w1645 w1659] -> w1593
              tunnel: [w1646 w1658] -> w1586
              tunnel: [w1644 w1657] -> w1592
              frame False {
                n549 = To Single Precision Float(number=w1655) -> (single precision float=w1656:sgl[])
                n550 = To Single Precision Float(number=w1651) -> (single precision float=w1653:sgl[])
                n551 = To Single Precision Float(number=w1650) -> (single precision float=w1652:sgl[])
                n552 = Divide(x=w1656, y=w1647) -> (x/y=w1654:sgl[])
                n553 = Divide(x=w1653, y=w1647) -> (x/y=w1649:sgl[])
                n554 = Divide(x=w1652, y=w1647) -> (x/y=w1648:sgl[])
              }
              frame True {
                n555 = To Single Precision Float(number=w1676) -> (single precision float=w1661:sgl[])
                n556 = To Single Precision Float(number=w1675) -> (single precision float=w1673:sgl[])
                n557 = To Single Precision Float(number=w1674) -> (single precision float=w1672:sgl[])
                n558 = call "IMAQ GetPixelLine"("Line Coordinates"=w1662, "Image"=w1658) -> ("Pixels Line (Float)"=w1665:sgl[])  [unwired: 2 in, 4 out]
                n559 = call "IMAQ GetPixelLine"("Line Coordinates"=w1662, "Image"=w1659) -> ("Pixels Line (Float)"=w1664:sgl[])  [unwired: 2 in, 4 out]
                n560 = call "IMAQ GetPixelLine"("Line Coordinates"=w1662, "Image"=w1657) -> ("Pixels Line (Float)"=w1663:sgl[])  [unwired: 2 in, 4 out]
                n561 = Divide(x=w1661, y=w1660) -> (x/y=w1671:sgl[])
                n562 = Divide(x=w1673, y=w1660) -> (x/y=w1670:sgl[])
                n563 = Divide(x=w1672, y=w1660) -> (x/y=w1669:sgl[])
                n564 = Add(x=w1665, y=w1671) -> (x+y=w1667:sgl[])
                n565 = Add(x=w1664, y=w1670) -> (x+y=w1668:sgl[])
                n566 = Add(x=w1663, y=w1669) -> (x+y=w1666:sgl[])
              }
            }
            n567 = stacked-sequence {
              tunnel: w1585 -> [w1625 _]
              tunnel: w1583 -> [w1627 _]
              tunnel: w1586 -> [w1626 _]
              tunnel: w1587 -> [_ w1631]
              tunnel: [w1625 _] -> w1584
              frame #0 {
                n568 = call "IMAQ SetPixelLine"("Pixels Line (Float)"=w1627, "Line Coordinates"=w1625, "Image"=w1626) -> ()  [unwired: 7 in, 2 out]
              }
              frame #1 {
                n569 = case shown="True" w1631 {
                  tunnel: [w1632 w1634] -> w1629
                  frame False {
                    n570 = call "Frame Counter.vi"("Action"=Counter_Action."Read") -> ("Num"=w1632:i32)
                  }
                  frame True {
                    n571 = call "Frame Counter.vi"("Action"=Counter_Action."Plus One") -> ("Num"=w1634:i32)
                  }
                }
                n572 = call "FPGA-7842R-Control V2.vi"("Current Frame"=w1629, "Action"=FPGA-7842R-Reference."Current Frame for Capture", "Initialize"=TRUE) -> ()  [unwired: 11 in, 2 out]
              }
            }
            n573 = call "IMAQ SetPixelLine"("Pixels Line (Float)"=w1613, "Line Coordinates"=w1584, "Image"=w1593) -> ()  [unwired: 7 in, 2 out]
            n574 = call "IMAQ SetPixelLine"("Pixels Line (Float)"=w1612, "Line Coordinates"=w1584, "Image"=w1592) -> ()  [unwired: 7 in, 2 out]
            n575 = And(x=w1601, y=w1600) -> (x .and. y?=w1602:bool)
            n576 = case shown="True" w1602 {
              tunnel: w1583 -> [_ w1643]
              tunnel: w1613 -> [_ w1642]
              tunnel: w1612 -> [_ w1641]
              tunnel: w1611 -> [_ w1639]
              tunnel: w1590 -> [_ w1638]
              tunnel: w1589 -> [_ w1637]
              tunnel: w1588 -> [_ w1636]
              frame False {
              }
              frame True {
                w1640 = FALSE ("prepend array or string size? (T)")
                n577 = Write to Binary File(file (use dialog)=w1638, data=w1643, 5:w1640, 9:w1639) -> ()  [unwired: 2 in, 3 out]
                n578 = Write to Binary File(file (use dialog)=w1637, data=w1642, 5:w1640, 9:w1639) -> ()  [unwired: 2 in, 3 out]
                n579 = Write to Binary File(file (use dialog)=w1636, data=w1641, 5:w1640, 9:w1639) -> ()  [unwired: 2 in, 3 out]
              }
            }
          }
        }
      }
    }
    frame 12 {
      n580 = while {
        shift-right: [w1714] -> _
        shift-left: 0 -> [w1715]
        tunnel: w1692 -> [w1716]
        tunnel: w1691 -> [w1713]
        tunnel: w1690 -> [w1712]
        tunnel: w1689 -> [w1711]
        tunnel: w1677 -> [w1707]
        shift-right: [w1704] -> _
        shift-left: u32 0 -> [w1705]
        tunnel: w1687 -> [w1703]
        tunnel: w1686 -> [w1702]
        tunnel: w1685 -> [w1701]
        tunnel: w1684 -> [w1700]
        tunnel: w1679 -> [w1699]
        tunnel: w1678 -> [w1698]
        tunnel: w1683 -> [w1697]
        tunnel: w1682 -> [w1696]
        tunnel: w1681 -> [w1695]
        tunnel: w1680 -> [w1694]
        stop <- w1706 stop-if-true
        n581 = Get Queue Status(queue=w1700) -> (queue out=w1708:refnum<queue>, # elements in queue=w1710:i32)  [unwired: 2 in, 6 out]
        n582 = Get Notifier Status(notifier=w1707) -> (current notification=w1706:bool)  [unwired: 1 in, 4 out]
        n583 = Greater Than 0?(x=w1710) -> (x > 0?=w1709:bool)
        n584 = case shown="True" w1709 {
          tunnel: w1716 -> [_ w1747]
          tunnel: w1715 -> [w1718 w1748]
          tunnel: [w1718 w1746] -> w1714
          tunnel: w1713 -> [_ w1744]
          tunnel: w1712 -> [_ w1743]
          tunnel: w1711 -> [_ w1733]
          tunnel: w1708 -> [_ w1742]
          tunnel: w1705 -> [w1717 w1739]
          tunnel: [w1717 w1738] -> w1704
          tunnel: w1703 -> [_ w1737]
          tunnel: w1702 -> [_ w1736]
          tunnel: w1701 -> [_ w1731]
          tunnel: w1699 -> [_ w1729]
          tunnel: w1698 -> [_ w1728]
          tunnel: w1697 -> [_ w1726]
          tunnel: w1696 -> [_ w1725]
          tunnel: w1695 -> [_ _]
          tunnel: w1694 -> [_ _]
          frame False {
          }
          frame True {
            # "False: 1st frame in fram accum"
            # "True: Last Frame of frame accum"
            # "Current Line in Frame Accum"
            # "Current Line In Frame"
            n585 = Increment(x=w1739) -> (x+1=w1732:u32)
            n586 = Dequeue Element(queue=w1742) -> (element=w1754:u64[])  [unwired: 2 in, 3 out]
            n587 = Equal?(x=w1732, y=w1736) -> (x = y?=w1741:bool)
            n588 = Greater?(x=w1732, y=w1737) -> (0:w1734:bool)
            n589 = Greater?(x=w1732, y=w1731) -> (0:w1730:bool)
            n590 = Split Number(x=w1754) -> (lo(x)=w1753:u32[])  [unwired: 1 out]
            n591 = Split Number(x=w1753) -> (hi(x)=w1724:u16[], lo(x)=w1752:u16[])
            n592 = Select(t=u32 0, s=w1741, f=w1732) -> (s? t:f=w1738:u32)
            n593 = Increment(x=w1748) -> (x+1=w1749:i32)
            n594 = Equal?(x=w1747, y=w1748) -> (x = y?=w1723:bool)
            n595 = Select(t=0, s=w1723, f=w1749) -> (s? t:f=w1746:i32)
            n596 = Build Array(0, w1748, w1747, w1748) -> (w1721:i32[])
            n597 = case shown="True" w1730 {
              tunnel: w1724 -> [w1779 w1794]
              tunnel: w1752 -> [w1776 w1793]
              tunnel: [w1778 w1789] -> w1719
              tunnel: [w1775 w1788] -> w1745
              tunnel: w1721 -> [_ w1785]
              tunnel: w1743 -> [w1774 w1783]
              tunnel: w1729 -> [w1773 w1782]
              tunnel: w1728 -> [w1772 w1781]
              tunnel: [w1773 w1782] -> w1722
              tunnel: [w1772 w1781] -> w1727
              frame False {
                n598 = To Single Precision Float(number=w1779) -> (single precision float=w1780:sgl[])
                n599 = To Single Precision Float(number=w1776) -> (single precision float=w1777:sgl[])
                n600 = Divide(x=w1780, y=w1774) -> (x/y=w1778:sgl[])
                n601 = Divide(x=w1777, y=w1774) -> (x/y=w1775:sgl[])
              }
              frame True {
                n602 = To Single Precision Float(number=w1794) -> (single precision float=w1784:sgl[])
                n603 = To Single Precision Float(number=w1793) -> (single precision float=w1792:sgl[])
                n604 = call "IMAQ GetPixelLine"("Line Coordinates"=w1785, "Image"=w1782) -> ("Pixels Line (Float)"=w1787:sgl[])  [unwired: 2 in, 4 out]
                n605 = call "IMAQ GetPixelLine"("Line Coordinates"=w1785, "Image"=w1781) -> ("Pixels Line (Float)"=w1786:sgl[])  [unwired: 2 in, 4 out]
                n606 = Divide(x=w1784, y=w1783) -> (x/y=w1791:sgl[])
                n607 = Divide(x=w1792, y=w1783) -> (x/y=w1790:sgl[])
                n608 = Add(x=w1787, y=w1791) -> (x+y=w1789:sgl[])
                n609 = Add(x=w1786, y=w1790) -> (x+y=w1788:sgl[])
              }
            }
            n610 = stacked-sequence {
              tunnel: w1721 -> [w1755 _]
              tunnel: w1719 -> [w1757 _]
              tunnel: w1722 -> [w1756 _]
              tunnel: w1723 -> [_ w1761]
              tunnel: [w1755 _] -> w1720
              frame #0 {
                n611 = call "IMAQ SetPixelLine"("Pixels Line (Float)"=w1757, "Line Coordinates"=w1755, "Image"=w1756) -> ()  [unwired: 7 in, 2 out]
              }
              frame #1 {
                n612 = case shown="True" w1761 {
                  tunnel: [w1762 w1764] -> w1759
                  frame False {
                    n613 = call "Frame Counter.vi"("Action"=Counter_Action."Read") -> ("Num"=w1762:i32)
                  }
                  frame True {
                    n614 = call "Frame Counter.vi"("Action"=Counter_Action."Plus One") -> ("Num"=w1764:i32)
                  }
                }
                n615 = call "FPGA-7842R-Control V2.vi"("Current Frame"=w1759, "Action"=FPGA-7842R-Reference."Current Frame for Capture", "Initialize"=TRUE) -> ()  [unwired: 11 in, 2 out]
              }
            }
            n616 = call "IMAQ SetPixelLine"("Pixels Line (Float)"=w1745, "Line Coordinates"=w1720, "Image"=w1727) -> ()  [unwired: 7 in, 2 out]
            n617 = And(x=w1734, y=w1733) -> (x .and. y?=w1735:bool)
            n618 = case shown="True" w1735 {
              tunnel: w1719 -> [_ w1771]
              tunnel: w1745 -> [_ w1770]
              tunnel: w1744 -> [_ w1768]
              tunnel: w1726 -> [_ w1767]
              tunnel: w1725 -> [_ w1766]
              frame False {
              }
              frame True {
                w1769 = FALSE ("prepend array or string size? (T)")
                n619 = Write to Binary File(file (use dialog)=w1767, data=w1771, 5:w1769, 9:w1768) -> ()  [unwired: 2 in, 3 out]
                n620 = Write to Binary File(file (use dialog)=w1766, data=w1770, 5:w1769, 9:w1768) -> ()  [unwired: 2 in, 3 out]
              }
            }
          }
        }
      }
    }
    frame 13 {
      n621 = while {
        shift-right: [w1834] -> _
        shift-left: 0 -> [w1835]
        tunnel: w1811 -> [w1836]
        tunnel: w1810 -> [w1833]
        tunnel: w1809 -> [w1832]
        tunnel: w1808 -> [w1831]
        tunnel: w1795 -> [w1827]
        shift-right: [w1824] -> _
        shift-left: u32 0 -> [w1825]
        tunnel: w1806 -> [w1823]
        tunnel: w1805 -> [w1822]
        tunnel: w1804 -> [w1821]
        tunnel: w1803 -> [w1820]
        tunnel: w1798 -> [w1819]
        tunnel: w1797 -> [w1818]
        tunnel: w1796 -> [w1817]
        tunnel: w1802 -> [w1816]
        tunnel: w1801 -> [w1815]
        tunnel: w1800 -> [w1814]
        tunnel: w1799 -> [w1813]
        stop <- w1826 stop-if-true
        n622 = Get Queue Status(queue=w1820) -> (queue out=w1828:refnum<queue>, # elements in queue=w1830:i32)  [unwired: 2 in, 6 out]
        n623 = Get Notifier Status(notifier=w1827) -> (current notification=w1826:bool)  [unwired: 1 in, 4 out]
        n624 = Greater Than 0?(x=w1830) -> (x > 0?=w1829:bool)
        n625 = case shown="True" w1829 {
          tunnel: w1836 -> [_ w1871]
          tunnel: w1835 -> [w1838 w1872]
          tunnel: [w1838 w1870] -> w1834
          tunnel: w1833 -> [_ w1867]
          tunnel: w1832 -> [_ w1866]
          tunnel: w1831 -> [_ w1856]
          tunnel: w1828 -> [_ w1865]
          tunnel: w1825 -> [w1837 w1862]
          tunnel: [w1837 w1861] -> w1824
          tunnel: w1823 -> [_ w1860]
          tunnel: w1822 -> [_ w1859]
          tunnel: w1821 -> [_ w1854]
          tunnel: w1819 -> [_ w1852]
          tunnel: w1818 -> [_ w1851]
          tunnel: w1817 -> [_ w1850]
          tunnel: w1816 -> [_ w1846]
          tunnel: w1815 -> [_ w1845]
          tunnel: w1814 -> [_ w1844]
          tunnel: w1813 -> [_ _]
          frame False {
          }
          frame True {
            # "False: 1st frame in fram accum"
            # "True: Last Frame of frame accum"
            # "Current Line in Frame Accum"
            # "Current Line In Frame"
            n626 = Increment(x=w1862) -> (x+1=w1855:u32)
            n627 = Dequeue Element(queue=w1865) -> (element=w1879:u64[])  [unwired: 2 in, 3 out]
            n628 = Equal?(x=w1855, y=w1859) -> (x = y?=w1864:bool)
            n629 = Greater?(x=w1855, y=w1860) -> (0:w1857:bool)
            n630 = Greater?(x=w1855, y=w1854) -> (0:w1853:bool)
            n631 = Split Number(x=w1879) -> (hi(x)=w1880:u32[], lo(x)=w1878:u32[])
            n632 = Split Number(x=w1880) -> (hi(x)=w1847:u16[])  [unwired: 1 out]
            n633 = Split Number(x=w1878) -> (hi(x)=w1877:u16[], lo(x)=w1876:u16[])
            n634 = Select(t=u32 0, s=w1864, f=w1855) -> (s? t:f=w1861:u32)
            n635 = Increment(x=w1872) -> (x+1=w1873:i32)
            n636 = Equal?(x=w1871, y=w1872) -> (x = y?=w1843:bool)
            n637 = Select(t=0, s=w1843, f=w1873) -> (s? t:f=w1870:i32)
            n638 = Build Array(0, w1872, w1871, w1872) -> (w1840:i32[])
            n639 = case shown="True" w1853 {
              tunnel: w1847 -> [w1911 w1932]
              tunnel: w1877 -> [w1907 w1931]
              tunnel: w1876 -> [w1906 w1930]
              tunnel: [w1905 w1924] -> w1869
              tunnel: [w1910 w1923] -> w1841
              tunnel: [w1904 w1922] -> w1868
              tunnel: w1840 -> [_ w1918]
              tunnel: w1866 -> [w1903 w1916]
              tunnel: w1852 -> [w1902 w1914]
              tunnel: w1851 -> [w1901 w1915]
              tunnel: w1850 -> [w1900 w1913]
              tunnel: [w1901 w1915] -> w1849
              tunnel: [w1902 w1914] -> w1842
              tunnel: [w1900 w1913] -> w1848
              frame False {
                n640 = To Single Precision Float(number=w1911) -> (single precision float=w1912:sgl[])
                n641 = To Single Precision Float(number=w1907) -> (single precision float=w1909:sgl[])
                n642 = To Single Precision Float(number=w1906) -> (single precision float=w1908:sgl[])
                n643 = Divide(x=w1912, y=w1903) -> (x/y=w1910:sgl[])
                n644 = Divide(x=w1909, y=w1903) -> (x/y=w1905:sgl[])
                n645 = Divide(x=w1908, y=w1903) -> (x/y=w1904:sgl[])
              }
              frame True {
                n646 = To Single Precision Float(number=w1932) -> (single precision float=w1917:sgl[])
                n647 = To Single Precision Float(number=w1931) -> (single precision float=w1929:sgl[])
                n648 = To Single Precision Float(number=w1930) -> (single precision float=w1928:sgl[])
                n649 = call "IMAQ GetPixelLine"("Line Coordinates"=w1918, "Image"=w1914) -> ("Pixels Line (Float)"=w1921:sgl[])  [unwired: 2 in, 4 out]
                n650 = call "IMAQ GetPixelLine"("Line Coordinates"=w1918, "Image"=w1915) -> ("Pixels Line (Float)"=w1920:sgl[])  [unwired: 2 in, 4 out]
                n651 = call "IMAQ GetPixelLine"("Line Coordinates"=w1918, "Image"=w1913) -> ("Pixels Line (Float)"=w1919:sgl[])  [unwired: 2 in, 4 out]
                n652 = Divide(x=w1917, y=w1916) -> (x/y=w1927:sgl[])
                n653 = Divide(x=w1929, y=w1916) -> (x/y=w1926:sgl[])
                n654 = Divide(x=w1928, y=w1916) -> (x/y=w1925:sgl[])
                n655 = Add(x=w1921, y=w1927) -> (x+y=w1923:sgl[])
                n656 = Add(x=w1920, y=w1926) -> (x+y=w1924:sgl[])
                n657 = Add(x=w1919, y=w1925) -> (x+y=w1922:sgl[])
              }
            }
            n658 = stacked-sequence {
              tunnel: w1840 -> [w1881 _]
              tunnel: w1841 -> [w1883 _]
              tunnel: w1842 -> [w1882 _]
              tunnel: w1843 -> [_ w1887]
              tunnel: [w1881 _] -> w1839
              frame #0 {
                n659 = call "IMAQ SetPixelLine"("Pixels Line (Float)"=w1883, "Line Coordinates"=w1881, "Image"=w1882) -> ()  [unwired: 7 in, 2 out]
              }
              frame #1 {
                n660 = case shown="True" w1887 {
                  tunnel: [w1888 w1890] -> w1885
                  frame False {
                    n661 = call "Frame Counter.vi"("Action"=Counter_Action."Read") -> ("Num"=w1888:i32)
                  }
                  frame True {
                    n662 = call "Frame Counter.vi"("Action"=Counter_Action."Plus One") -> ("Num"=w1890:i32)
                  }
                }
                n663 = call "FPGA-7842R-Control V2.vi"("Current Frame"=w1885, "Action"=FPGA-7842R-Reference."Current Frame for Capture", "Initialize"=TRUE) -> ()  [unwired: 11 in, 2 out]
              }
            }
            n664 = call "IMAQ SetPixelLine"("Pixels Line (Float)"=w1869, "Line Coordinates"=w1839, "Image"=w1849) -> ()  [unwired: 7 in, 2 out]
            n665 = call "IMAQ SetPixelLine"("Pixels Line (Float)"=w1868, "Line Coordinates"=w1839, "Image"=w1848) -> ()  [unwired: 7 in, 2 out]
            n666 = And(x=w1857, y=w1856) -> (x .and. y?=w1858:bool)
            n667 = case shown="True" w1858 {
              tunnel: w1841 -> [_ w1899]
              tunnel: w1869 -> [_ w1898]
              tunnel: w1868 -> [_ w1897]
              tunnel: w1867 -> [_ w1895]
              tunnel: w1846 -> [_ w1894]
              tunnel: w1845 -> [_ w1893]
              tunnel: w1844 -> [_ w1892]
              frame False {
              }
              frame True {
                w1896 = FALSE ("prepend array or string size? (T)")
                n668 = Write to Binary File(file (use dialog)=w1894, data=w1899, 5:w1896, 9:w1895) -> ()  [unwired: 2 in, 3 out]
                n669 = Write to Binary File(file (use dialog)=w1893, data=w1898, 5:w1896, 9:w1895) -> ()  [unwired: 2 in, 3 out]
                n670 = Write to Binary File(file (use dialog)=w1892, data=w1897, 5:w1896, 9:w1895) -> ()  [unwired: 2 in, 3 out]
              }
            }
          }
        }
      }
    }
    frame 14 {
      n671 = while {
        shift-right: [w1972] -> _
        shift-left: 0 -> [w1973]
        tunnel: w1949 -> [w1974]
        tunnel: w1948 -> [w1971]
        tunnel: w1947 -> [w1970]
        tunnel: w1946 -> [w1969]
        tunnel: w1933 -> [w1965]
        shift-right: [w1962] -> _
        shift-left: u32 0 -> [w1963]
        tunnel: w1944 -> [w1961]
        tunnel: w1943 -> [w1960]
        tunnel: w1942 -> [w1959]
        tunnel: w1941 -> [w1958]
        tunnel: w1936 -> [w1953]
        tunnel: w1935 -> [w1952]
        tunnel: w1934 -> [w1951]
        tunnel: w1940 -> [w1957]
        tunnel: w1939 -> [w1956]
        tunnel: w1938 -> [w1955]
        tunnel: w1937 -> [w1954]
        stop <- w1964 stop-if-true
        n672 = Get Queue Status(queue=w1958) -> (queue out=w1966:refnum<queue>, # elements in queue=w1968:i32)  [unwired: 2 in, 6 out]
        n673 = Get Notifier Status(notifier=w1965) -> (current notification=w1964:bool)  [unwired: 1 in, 4 out]
        n674 = Greater Than 0?(x=w1968) -> (x > 0?=w1967:bool)
        n675 = case shown="True" w1967 {
          tunnel: w1974 -> [_ w2008]
          tunnel: w1973 -> [w1976 w2009]
          tunnel: [w1976 w2007] -> w1972
          tunnel: w1971 -> [_ w2004]
          tunnel: w1970 -> [_ w2003]
          tunnel: w1969 -> [_ w1993]
          tunnel: w1966 -> [_ w2002]
          tunnel: w1963 -> [w1975 w1999]
          tunnel: [w1975 w1998] -> w1962
          tunnel: w1961 -> [_ w1997]
          tunnel: w1960 -> [_ w1996]
          tunnel: w1959 -> [_ w1991]
          tunnel: w1953 -> [_ w1989]
          tunnel: w1952 -> [_ w1988]
          tunnel: w1951 -> [_ w1987]
          tunnel: w1957 -> [_ w1984]
          tunnel: w1956 -> [_ w1983]
          tunnel: w1955 -> [_ w1982]
          tunnel: w1954 -> [_ _]
          frame False {
          }
          frame True {
            # "False: 1st frame in fram accum"
            # "True: Last Frame of frame accum"
            # "Current Line in Frame Accum"
            # "Current Line In Frame"
            n676 = Increment(x=w1999) -> (x+1=w1992:u32)
            n677 = Dequeue Element(queue=w2002) -> (element=w2017:u64[])  [unwired: 2 in, 3 out]
            n678 = Equal?(x=w1992, y=w1996) -> (x = y?=w2001:bool)
            n679 = Greater?(x=w1992, y=w1997) -> (0:w1994:bool)
            n680 = Greater?(x=w1992, y=w1991) -> (0:w1990:bool)
            n681 = Split Number(x=w2017) -> (hi(x)=w2018:u32[], lo(x)=w2016:u32[])
            n682 = Split Number(x=w2018) -> (lo(x)=w2015:u16[])  [unwired: 1 out]
            n683 = Split Number(x=w2016) -> (hi(x)=w2014:u16[], lo(x)=w2013:u16[])
            n684 = Select(t=u32 0, s=w2001, f=w1992) -> (s? t:f=w1998:u32)
            n685 = Increment(x=w2009) -> (x+1=w2010:i32)
            n686 = Equal?(x=w2008, y=w2009) -> (x = y?=w1981:bool)
            n687 = Select(t=0, s=w1981, f=w2010) -> (s? t:f=w2007:i32)
            n688 = Build Array(0, w2009, w2008, w2009) -> (w1978:i32[])
            n689 = case shown="True" w1990 {
              tunnel: w2015 -> [w2047 w2070]
              tunnel: w2014 -> [w2046 w2069]
              tunnel: w2013 -> [w2045 w2068]
              tunnel: [w2043 w2061] -> w2006
              tunnel: [w2044 w2060] -> w1979
              tunnel: [w2042 w2059] -> w2005
              tunnel: w1978 -> [_ w2055]
              tunnel: w2003 -> [w2041 w2054]
              tunnel: w1989 -> [w2040 w2052]
              tunnel: w1988 -> [w2039 w2053]
              tunnel: w1987 -> [w2038 w2051]
              tunnel: [w2039 w2053] -> w1986
              tunnel: [w2040 w2052] -> w1980
              tunnel: [w2038 w2051] -> w1985
              frame False {
                n690 = To Single Precision Float(number=w2047) -> (single precision float=w2050:sgl[])
                n691 = To Single Precision Float(number=w2046) -> (single precision float=w2049:sgl[])
                n692 = To Single Precision Float(number=w2045) -> (single precision float=w2048:sgl[])
                n693 = Divide(x=w2050, y=w2041) -> (x/y=w2044:sgl[])
                n694 = Divide(x=w2049, y=w2041) -> (x/y=w2043:sgl[])
                n695 = Divide(x=w2048, y=w2041) -> (x/y=w2042:sgl[])
              }
              frame True {
                n696 = To Single Precision Float(number=w2070) -> (single precision float=w2067:sgl[])
                n697 = To Single Precision Float(number=w2069) -> (single precision float=w2066:sgl[])
                n698 = To Single Precision Float(number=w2068) -> (single precision float=w2065:sgl[])
                n699 = call "IMAQ GetPixelLine"("Line Coordinates"=w2055, "Image"=w2052) -> ("Pixels Line (Float)"=w2058:sgl[])  [unwired: 2 in, 4 out]
                n700 = call "IMAQ GetPixelLine"("Line Coordinates"=w2055, "Image"=w2053) -> ("Pixels Line (Float)"=w2057:sgl[])  [unwired: 2 in, 4 out]
                n701 = call "IMAQ GetPixelLine"("Line Coordinates"=w2055, "Image"=w2051) -> ("Pixels Line (Float)"=w2056:sgl[])  [unwired: 2 in, 4 out]
                n702 = Divide(x=w2067, y=w2054) -> (x/y=w2064:sgl[])
                n703 = Divide(x=w2066, y=w2054) -> (x/y=w2063:sgl[])
                n704 = Divide(x=w2065, y=w2054) -> (x/y=w2062:sgl[])
                n705 = Add(x=w2058, y=w2064) -> (x+y=w2060:sgl[])
                n706 = Add(x=w2057, y=w2063) -> (x+y=w2061:sgl[])
                n707 = Add(x=w2056, y=w2062) -> (x+y=w2059:sgl[])
              }
            }
            n708 = stacked-sequence {
              tunnel: w1978 -> [w2019 _]
              tunnel: w1979 -> [w2021 _]
              tunnel: w1980 -> [w2020 _]
              tunnel: w1981 -> [_ w2025]
              tunnel: [w2019 _] -> w1977
              frame #0 {
                n709 = call "IMAQ SetPixelLine"("Pixels Line (Float)"=w2021, "Line Coordinates"=w2019, "Image"=w2020) -> ()  [unwired: 7 in, 2 out]
              }
              frame #1 {
                n710 = case shown="True" w2025 {
                  tunnel: [w2026 w2028] -> w2023
                  frame False {
                    n711 = call "Frame Counter.vi"("Action"=Counter_Action."Read") -> ("Num"=w2026:i32)
                  }
                  frame True {
                    n712 = call "Frame Counter.vi"("Action"=Counter_Action."Plus One") -> ("Num"=w2028:i32)
                  }
                }
                n713 = call "FPGA-7842R-Control V2.vi"("Current Frame"=w2023, "Action"=FPGA-7842R-Reference."Current Frame for Capture", "Initialize"=TRUE) -> ()  [unwired: 11 in, 2 out]
              }
            }
            n714 = call "IMAQ SetPixelLine"("Pixels Line (Float)"=w2006, "Line Coordinates"=w1977, "Image"=w1986) -> ()  [unwired: 7 in, 2 out]
            n715 = call "IMAQ SetPixelLine"("Pixels Line (Float)"=w2005, "Line Coordinates"=w1977, "Image"=w1985) -> ()  [unwired: 7 in, 2 out]
            n716 = And(x=w1994, y=w1993) -> (x .and. y?=w1995:bool)
            n717 = case shown="True" w1995 {
              tunnel: w1979 -> [_ w2037]
              tunnel: w2006 -> [_ w2036]
              tunnel: w2005 -> [_ w2035]
              tunnel: w2004 -> [_ w2033]
              tunnel: w1984 -> [_ w2032]
              tunnel: w1983 -> [_ w2031]
              tunnel: w1982 -> [_ w2030]
              frame False {
              }
              frame True {
                w2034 = FALSE ("prepend array or string size? (T)")
                n718 = Write to Binary File(file (use dialog)=w2032, data=w2037, 5:w2034, 9:w2033) -> ()  [unwired: 2 in, 3 out]
                n719 = Write to Binary File(file (use dialog)=w2031, data=w2036, 5:w2034, 9:w2033) -> ()  [unwired: 2 in, 3 out]
                n720 = Write to Binary File(file (use dialog)=w2030, data=w2035, 5:w2034, 9:w2033) -> ()  [unwired: 2 in, 3 out]
              }
            }
          }
        }
      }
    }
    frame 15 {
      n721 = while {
        shift-right: [w2112] -> _
        shift-left: 0 -> [w2113]
        tunnel: w2088 -> [w2114]
        tunnel: w2087 -> [w2111]
        tunnel: w2086 -> [w2110]
        tunnel: w2085 -> [w2109]
        tunnel: w2071 -> [w2105]
        shift-right: [w2102] -> _
        shift-left: u32 0 -> [w2103]
        tunnel: w2083 -> [w2101]
        tunnel: w2082 -> [w2100]
        tunnel: w2081 -> [w2099]
        tunnel: w2080 -> [w2098]
        tunnel: w2075 -> [w2097]
        tunnel: w2074 -> [w2096]
        tunnel: w2073 -> [w2095]
        tunnel: w2072 -> [w2094]
        tunnel: w2079 -> [w2093]
        tunnel: w2078 -> [w2092]
        tunnel: w2077 -> [w2091]
        tunnel: w2076 -> [w2090]
        stop <- w2104 stop-if-true
        n722 = Get Queue Status(queue=w2098) -> (queue out=w2106:refnum<queue>, # elements in queue=w2108:i32)  [unwired: 2 in, 6 out]
        n723 = Get Notifier Status(notifier=w2105) -> (current notification=w2104:bool)  [unwired: 1 in, 4 out]
        n724 = Greater Than 0?(x=w2108) -> (x > 0?=w2107:bool)
        n725 = case shown="True" w2107 {
          tunnel: w2114 -> [_ w2153]
          tunnel: w2113 -> [w2116 w2154]
          tunnel: [w2116 w2152] -> w2112
          tunnel: w2111 -> [_ w2148]
          tunnel: w2110 -> [_ w2147]
          tunnel: w2109 -> [_ w2137]
          tunnel: w2106 -> [_ w2146]
          tunnel: w2103 -> [w2115 w2143]
          tunnel: [w2115 w2142] -> w2102
          tunnel: w2101 -> [_ w2141]
          tunnel: w2100 -> [_ w2140]
          tunnel: w2099 -> [_ w2135]
          tunnel: w2097 -> [_ w2133]
          tunnel: w2096 -> [_ w2132]
          tunnel: w2095 -> [_ w2131]
          tunnel: w2094 -> [_ w2130]
          tunnel: w2093 -> [_ w2125]
          tunnel: w2092 -> [_ w2124]
          tunnel: w2091 -> [_ w2123]
          tunnel: w2090 -> [_ w2122]
          frame False {
          }
          frame True {
            # "False: 1st frame in fram accum"
            # "True: Last Frame of frame accum"
            # "Current Line in Frame Accum"
            # "Current Line In Frame"
            n726 = Increment(x=w2143) -> (x+1=w2136:u32)
            n727 = Dequeue Element(queue=w2146) -> (element=w2162:u64[])  [unwired: 2 in, 3 out]
            n728 = Equal?(x=w2136, y=w2140) -> (x = y?=w2145:bool)
            n729 = Greater?(x=w2136, y=w2141) -> (0:w2138:bool)
            n730 = Greater?(x=w2136, y=w2135) -> (0:w2134:bool)
            n731 = Split Number(x=w2162) -> (hi(x)=w2163:u32[], lo(x)=w2161:u32[])
            n732 = Split Number(x=w2163) -> (hi(x)=w2126:u16[], lo(x)=w2160:u16[])
            n733 = Split Number(x=w2161) -> (hi(x)=w2159:u16[], lo(x)=w2158:u16[])
            n734 = Select(t=u32 0, s=w2145, f=w2136) -> (s? t:f=w2142:u32)
            n735 = Increment(x=w2154) -> (x+1=w2155:i32)
            n736 = Equal?(x=w2153, y=w2154) -> (x = y?=w2121:bool)
            n737 = Select(t=0, s=w2121, f=w2155) -> (s? t:f=w2152:i32)
            n738 = Build Array(0, w2154, w2153, w2154) -> (w2120:i32[])
            n739 = case shown="True" w2134 {
              tunnel: w2126 -> [w2200 w2227]
              tunnel: w2160 -> [w2195 w2226]
              tunnel: w2159 -> [w2194 w2225]
              tunnel: w2158 -> [w2193 w2224]
              tunnel: [w2191 w2216] -> w2150
              tunnel: [w2192 w2215] -> w2151
              tunnel: [w2199 w2214] -> w2118
              tunnel: [w2190 w2213] -> w2149
              tunnel: w2120 -> [_ w2208]
              tunnel: w2147 -> [w2189 w2206]
              tunnel: w2133 -> [w2188 w2203]
              tunnel: w2132 -> [w2187 w2204]
              tunnel: w2131 -> [w2186 w2205]
              tunnel: w2130 -> [w2185 w2202]
              tunnel: [w2186 w2205] -> w2128
              tunnel: [w2187 w2204] -> w2129
              tunnel: [w2188 w2203] -> w2119
              tunnel: [w2185 w2202] -> w2127
              frame False {
                n740 = To Single Precision Float(number=w2200) -> (single precision float=w2201:sgl[])
                n741 = To Single Precision Float(number=w2195) -> (single precision float=w2198:sgl[])
                n742 = To Single Precision Float(number=w2194) -> (single precision float=w2197:sgl[])
                n743 = To Single Precision Float(number=w2193) -> (single precision float=w2196:sgl[])
                n744 = Divide(x=w2201, y=w2189) -> (x/y=w2199:sgl[])
                n745 = Divide(x=w2198, y=w2189) -> (x/y=w2192:sgl[])
                n746 = Divide(x=w2197, y=w2189) -> (x/y=w2191:sgl[])
                n747 = Divide(x=w2196, y=w2189) -> (x/y=w2190:sgl[])
              }
              frame True {
                n748 = To Single Precision Float(number=w2227) -> (single precision float=w2207:sgl[])
                n749 = To Single Precision Float(number=w2226) -> (single precision float=w2223:sgl[])
                n750 = To Single Precision Float(number=w2225) -> (single precision float=w2222:sgl[])
                n751 = To Single Precision Float(number=w2224) -> (single precision float=w2221:sgl[])
                n752 = call "IMAQ GetPixelLine"("Line Coordinates"=w2208, "Image"=w2203) -> ("Pixels Line (Float)"=w2212:sgl[])  [unwired: 2 in, 4 out]
                n753 = call "IMAQ GetPixelLine"("Line Coordinates"=w2208, "Image"=w2204) -> ("Pixels Line (Float)"=w2211:sgl[])  [unwired: 2 in, 4 out]
                n754 = call "IMAQ GetPixelLine"("Line Coordinates"=w2208, "Image"=w2205) -> ("Pixels Line (Float)"=w2210:sgl[])  [unwired: 2 in, 4 out]
                n755 = call "IMAQ GetPixelLine"("Line Coordinates"=w2208, "Image"=w2202) -> ("Pixels Line (Float)"=w2209:sgl[])  [unwired: 2 in, 4 out]
                n756 = Divide(x=w2207, y=w2206) -> (x/y=w2220:sgl[])
                n757 = Divide(x=w2223, y=w2206) -> (x/y=w2219:sgl[])
                n758 = Divide(x=w2222, y=w2206) -> (x/y=w2218:sgl[])
                n759 = Divide(x=w2221, y=w2206) -> (x/y=w2217:sgl[])
                n760 = Add(x=w2212, y=w2220) -> (x+y=w2214:sgl[])
                n761 = Add(x=w2211, y=w2219) -> (x+y=w2215:sgl[])
                n762 = Add(x=w2210, y=w2218) -> (x+y=w2216:sgl[])
                n763 = Add(x=w2209, y=w2217) -> (x+y=w2213:sgl[])
              }
            }
            n764 = stacked-sequence {
              tunnel: w2120 -> [w2164 _]
              tunnel: w2118 -> [w2166 _]
              tunnel: w2119 -> [w2165 _]
              tunnel: w2121 -> [_ w2170]
              tunnel: [w2164 _] -> w2117
              frame #0 {
                n765 = call "IMAQ SetPixelLine"("Pixels Line (Float)"=w2166, "Line Coordinates"=w2164, "Image"=w2165) -> ()  [unwired: 7 in, 2 out]
              }
              frame #1 {
                n766 = case shown="True" w2170 {
                  tunnel: [w2171 w2173] -> w2168
                  frame False {
                    n767 = call "Frame Counter.vi"("Action"=Counter_Action."Read") -> ("Num"=w2171:i32)
                  }
                  frame True {
                    n768 = call "Frame Counter.vi"("Action"=Counter_Action."Plus One") -> ("Num"=w2173:i32)
                  }
                }
                n769 = call "FPGA-7842R-Control V2.vi"("Current Frame"=w2168, "Action"=FPGA-7842R-Reference."Current Frame for Capture", "Initialize"=TRUE) -> ()  [unwired: 11 in, 2 out]
              }
            }
            n770 = call "IMAQ SetPixelLine"("Pixels Line (Float)"=w2151, "Line Coordinates"=w2117, "Image"=w2129) -> ()  [unwired: 7 in, 2 out]
            n771 = call "IMAQ SetPixelLine"("Pixels Line (Float)"=w2150, "Line Coordinates"=w2117, "Image"=w2128) -> ()  [unwired: 7 in, 2 out]
            n772 = call "IMAQ SetPixelLine"("Pixels Line (Float)"=w2149, "Line Coordinates"=w2117, "Image"=w2127) -> ()  [unwired: 7 in, 2 out]
            n773 = And(x=w2138, y=w2137) -> (x .and. y?=w2139:bool)
            n774 = case shown="True" w2139 {
              tunnel: w2118 -> [_ w2184]
              tunnel: w2151 -> [_ w2183]
              tunnel: w2150 -> [_ w2182]
              tunnel: w2149 -> [_ w2181]
              tunnel: w2148 -> [_ w2179]
              tunnel: w2125 -> [_ w2178]
              tunnel: w2124 -> [_ w2177]
              tunnel: w2123 -> [_ w2176]
              tunnel: w2122 -> [_ w2175]
              frame False {
              }
              frame True {
                w2180 = FALSE ("prepend array or string size? (T)")
                n775 = Write to Binary File(file (use dialog)=w2178, data=w2184, 5:w2180, 9:w2179) -> ()  [unwired: 2 in, 3 out]
                n776 = Write to Binary File(file (use dialog)=w2177, data=w2183, 5:w2180, 9:w2179) -> ()  [unwired: 2 in, 3 out]
                n777 = Write to Binary File(file (use dialog)=w2176, data=w2182, 5:w2180, 9:w2179) -> ()  [unwired: 2 in, 3 out]
                n778 = Write to Binary File(file (use dialog)=w2175, data=w2181, 5:w2180, 9:w2179) -> ()  [unwired: 2 in, 3 out]
              }
            }
          }
        }
      }
    }
    frame 19 {
      n779 = while {
        shift-right: [w2263] -> _
        shift-left: 0 -> [w2264]
        tunnel: w2242 -> [w2265]
        tunnel: w2241 -> [w2262]
        tunnel: w2240 -> [w2261]
        tunnel: w2239 -> [w2260]
        tunnel: w2228 -> [w2256]
        shift-right: [w2253] -> _
        shift-left: u32 0 -> [w2254]
        tunnel: w2237 -> [w2252]
        tunnel: w2236 -> [w2251]
        tunnel: w2235 -> [w2250]
        tunnel: w2234 -> [w2249]
        tunnel: w2229 -> [w2248]
        tunnel: w2233 -> [w2247]
        tunnel: w2232 -> [w2246]
        tunnel: w2231 -> [w2245]
        tunnel: w2230 -> [w2244]
        stop <- w2255 stop-if-true
        n780 = Get Queue Status(queue=w2249) -> (queue out=w2257:refnum<queue>, # elements in queue=w2259:i32)  [unwired: 2 in, 6 out]
        n781 = Get Notifier Status(notifier=w2256) -> (current notification=w2255:bool)  [unwired: 1 in, 4 out]
        n782 = Greater Than 0?(x=w2259) -> (x > 0?=w2258:bool)
        n783 = case shown="True" w2258 {
          tunnel: w2265 -> [_ w2295]
          tunnel: w2264 -> [w2267 w2296]
          tunnel: [w2267 w2294] -> w2263
          tunnel: w2262 -> [_ w2293]
          tunnel: w2261 -> [_ w2292]
          tunnel: w2260 -> [_ w2282]
          tunnel: w2257 -> [_ w2291]
          tunnel: w2254 -> [w2266 w2288]
          tunnel: [w2266 w2287] -> w2253
          tunnel: w2252 -> [_ w2286]
          tunnel: w2251 -> [_ w2285]
          tunnel: w2250 -> [_ w2280]
          tunnel: w2248 -> [_ w2278]
          tunnel: w2247 -> [_ w2277]
          tunnel: w2246 -> [_ _]
          tunnel: w2245 -> [_ _]
          tunnel: w2244 -> [_ _]
          frame False {
          }
          frame True {
            # "True: Last Frame of frame accum"
            # "Current Line in Frame Accum"
            # "Current Line In Frame"
            n784 = Increment(x=w2288) -> (x+1=w2281:u32)
            n785 = Dequeue Element(queue=w2291) -> (element=w2300:u64[])  [unwired: 2 in, 3 out]
            n786 = Equal?(x=w2281, y=w2285) -> (x = y?=w2290:bool)
            n787 = Greater?(x=w2281, y=w2286) -> (0:w2283:bool)
            n788 = Greater?(x=w2281, y=w2280) -> (0:w2279:bool)
            n789 = Split Number(x=w2300) -> (hi(x)=w2301:u32[])  [unwired: 1 out]
            n790 = Split Number(x=w2301) -> (hi(x)=w2276:u16[], lo(x)=w2275:u16[])
            n791 = Select(t=u32 0, s=w2290, f=w2281) -> (s? t:f=w2287:u32)
            n792 = Increment(x=w2296) -> (x+1=w2297:i32)
            n793 = Equal?(x=w2295, y=w2296) -> (x = y?=w2271:bool)
            n794 = To Single Precision Float(number=w2276) -> (single precision float=w2274:sgl[])
            n795 = To Single Precision Float(number=w2275) -> (single precision float=w2273:sgl[])
            n796 = Select(t=0, s=w2271, f=w2297) -> (s? t:f=w2294:i32)
            n797 = Add(x=w2274, y=w2273) -> (x+y=w2272:sgl[])
            n798 = Build Array(0, w2296, w2295, w2296) -> (w2270:i32[])
            n799 = case shown="True" w2279 {
              tunnel: [w2320 w2326] -> w2268
              tunnel: w2270 -> [_ w2324]
              tunnel: w2292 -> [w2319 w2323]
              tunnel: w2278 -> [w2318 w2322]
              tunnel: [w2318 w2322] -> w2269
              tunnel: w2272 -> [w2317 w2321]
              frame False {
                n800 = Divide(x=w2317, y=w2319) -> (x/y=w2320:sgl[])
              }
              frame True {
                n801 = call "IMAQ GetPixelLine"("Line Coordinates"=w2324, "Image"=w2322) -> ("Pixels Line (Float)"=w2325:sgl[])  [unwired: 2 in, 4 out]
                n802 = Divide(x=w2321, y=w2323) -> (x/y=w2327:sgl[])
                n803 = Add(x=w2325, y=w2327) -> (x+y=w2326:sgl[])
              }
            }
            n804 = stacked-sequence {
              tunnel: w2270 -> [w2304 _]
              tunnel: w2268 -> [w2303 _]
              tunnel: w2269 -> [w2302 _]
              tunnel: w2271 -> [_ w2308]
              frame #0 {
                n805 = call "IMAQ SetPixelLine"("Pixels Line (Float)"=w2303, "Line Coordinates"=w2304, "Image"=w2302) -> ()  [unwired: 7 in, 2 out]
              }
              frame #1 {
                n806 = case shown="True" w2308 {
                  tunnel: [w2309 w2311] -> w2306
                  frame False {
                    n807 = call "Frame Counter.vi"("Action"=Counter_Action."Read") -> ("Num"=w2309:i32)
                  }
                  frame True {
                    n808 = call "Frame Counter.vi"("Action"=Counter_Action."Plus One") -> ("Num"=w2311:i32)
                  }
                }
                n809 = call "FPGA-7842R-Control V2.vi"("Current Frame"=w2306, "Action"=FPGA-7842R-Reference."Current Frame for Capture", "Initialize"=TRUE) -> ()  [unwired: 11 in, 2 out]
              }
            }
            n810 = And(x=w2283, y=w2282) -> (x .and. y?=w2284:bool)
            n811 = case shown="True" w2284 {
              tunnel: w2268 -> [_ w2316]
              tunnel: w2293 -> [_ w2314]
              tunnel: w2277 -> [_ w2313]
              frame False {
              }
              frame True {
                n812 = Write to Binary File(file (use dialog)=w2313, data=w2316, 5:FALSE ("prepend array or string size? (T)"), 9:w2314) -> ()  [unwired: 2 in, 3 out]
              }
            }
          }
        }
      }
    }
    frame 21 {
      n813 = while {
        shift-right: [w2363] -> _
        shift-left: 0 -> [w2364]
        tunnel: w2342 -> [w2365]
        tunnel: w2341 -> [w2362]
        tunnel: w2340 -> [w2361]
        tunnel: w2339 -> [w2360]
        tunnel: w2328 -> [w2356]
        shift-right: [w2353] -> _
        shift-left: u32 0 -> [w2354]
        tunnel: w2337 -> [w2352]
        tunnel: w2336 -> [w2351]
        tunnel: w2335 -> [w2350]
        tunnel: w2334 -> [w2349]
        tunnel: w2329 -> [w2348]
        tunnel: w2333 -> [w2347]
        tunnel: w2332 -> [w2346]
        tunnel: w2331 -> [w2345]
        tunnel: w2330 -> [w2344]
        stop <- w2355 stop-if-true
        n814 = Get Queue Status(queue=w2349) -> (queue out=w2357:refnum<queue>, # elements in queue=w2359:i32)  [unwired: 2 in, 6 out]
        n815 = Get Notifier Status(notifier=w2356) -> (current notification=w2355:bool)  [unwired: 1 in, 4 out]
        n816 = Greater Than 0?(x=w2359) -> (x > 0?=w2358:bool)
        n817 = case shown="True" w2358 {
          tunnel: w2365 -> [_ w2395]
          tunnel: w2364 -> [w2367 w2396]
          tunnel: [w2367 w2394] -> w2363
          tunnel: w2362 -> [_ w2393]
          tunnel: w2361 -> [_ w2392]
          tunnel: w2360 -> [_ w2382]
          tunnel: w2357 -> [_ w2391]
          tunnel: w2354 -> [w2366 w2388]
          tunnel: [w2366 w2387] -> w2353
          tunnel: w2352 -> [_ w2386]
          tunnel: w2351 -> [_ w2385]
          tunnel: w2350 -> [_ w2380]
          tunnel: w2348 -> [_ w2378]
          tunnel: w2347 -> [_ w2377]
          tunnel: w2346 -> [_ _]
          tunnel: w2345 -> [_ _]
          tunnel: w2344 -> [_ _]
          frame False {
          }
          frame True {
            # "True: Last Frame of frame accum"
            # "Current Line in Frame Accum"
            # "Current Line In Frame"
            n818 = Increment(x=w2388) -> (x+1=w2381:u32)
            n819 = Dequeue Element(queue=w2391) -> (element=w2401:u64[])  [unwired: 2 in, 3 out]
            n820 = Equal?(x=w2381, y=w2385) -> (x = y?=w2390:bool)
            n821 = Greater?(x=w2381, y=w2386) -> (0:w2383:bool)
            n822 = Greater?(x=w2381, y=w2380) -> (0:w2379:bool)
            n823 = Split Number(x=w2401) -> (hi(x)=w2402:u32[], lo(x)=w2400:u32[])
            n824 = Split Number(x=w2402) -> (hi(x)=w2376:u16[])  [unwired: 1 out]
            n825 = Split Number(x=w2400) -> (hi(x)=w2372:u16[])  [unwired: 1 out]
            n826 = Select(t=u32 0, s=w2390, f=w2381) -> (s? t:f=w2387:u32)
            n827 = Increment(x=w2396) -> (x+1=w2397:i32)
            n828 = Equal?(x=w2395, y=w2396) -> (x = y?=w2371:bool)
            n829 = To Single Precision Float(number=w2376) -> (single precision float=w2375:sgl[])
            n830 = To Single Precision Float(number=w2372) -> (single precision float=w2374:sgl[])
            n831 = Select(t=0, s=w2371, f=w2397) -> (s? t:f=w2394:i32)
            n832 = Add(x=w2375, y=w2374) -> (x+y=w2373:sgl[])
            n833 = Build Array(0, w2396, w2395, w2396) -> (w2370:i32[])
            n834 = case shown="False" w2379 {
              tunnel: [w2421 w2427] -> w2368
              tunnel: w2370 -> [_ w2425]
              tunnel: w2392 -> [w2420 w2424]
              tunnel: w2378 -> [w2419 w2423]
              tunnel: [w2419 w2423] -> w2369
              tunnel: w2373 -> [w2418 w2422]
              frame False {
                n835 = Divide(x=w2418, y=w2420) -> (x/y=w2421:sgl[])
              }
              frame True {
                n836 = call "IMAQ GetPixelLine"("Line Coordinates"=w2425, "Image"=w2423) -> ("Pixels Line (Float)"=w2426:sgl[])  [unwired: 2 in, 4 out]
                n837 = Divide(x=w2422, y=w2424) -> (x/y=w2428:sgl[])
                n838 = Add(x=w2426, y=w2428) -> (x+y=w2427:sgl[])
              }
            }
            n839 = stacked-sequence {
              tunnel: w2370 -> [w2405 _]
              tunnel: w2368 -> [w2404 _]
              tunnel: w2369 -> [w2403 _]
              tunnel: w2371 -> [_ w2409]
              frame #0 {
                n840 = call "IMAQ SetPixelLine"("Pixels Line (Float)"=w2404, "Line Coordinates"=w2405, "Image"=w2403) -> ()  [unwired: 7 in, 2 out]
              }
              frame #1 {
                n841 = case shown="True" w2409 {
                  tunnel: [w2410 w2412] -> w2407
                  frame False {
                    n842 = call "Frame Counter.vi"("Action"=Counter_Action."Read") -> ("Num"=w2410:i32)
                  }
                  frame True {
                    n843 = call "Frame Counter.vi"("Action"=Counter_Action."Plus One") -> ("Num"=w2412:i32)
                  }
                }
                n844 = call "FPGA-7842R-Control V2.vi"("Current Frame"=w2407, "Action"=FPGA-7842R-Reference."Current Frame for Capture", "Initialize"=TRUE) -> ()  [unwired: 11 in, 2 out]
              }
            }
            n845 = And(x=w2383, y=w2382) -> (x .and. y?=w2384:bool)
            n846 = case shown="True" w2384 {
              tunnel: w2368 -> [_ w2417]
              tunnel: w2393 -> [_ w2415]
              tunnel: w2377 -> [_ w2414]
              frame False {
              }
              frame True {
                n847 = Write to Binary File(file (use dialog)=w2414, data=w2417, 5:FALSE ("prepend array or string size? (T)"), 9:w2415) -> ()  [unwired: 2 in, 3 out]
              }
            }
          }
        }
      }
    }
    frame 22 {
      n848 = while {
        shift-right: [w2464] -> _
        shift-left: 0 -> [w2465]
        tunnel: w2443 -> [w2466]
        tunnel: w2442 -> [w2463]
        tunnel: w2441 -> [w2462]
        tunnel: w2440 -> [w2461]
        tunnel: w2429 -> [w2457]
        shift-right: [w2454] -> _
        shift-left: u32 0 -> [w2455]
        tunnel: w2438 -> [w2453]
        tunnel: w2437 -> [w2452]
        tunnel: w2436 -> [w2451]
        tunnel: w2435 -> [w2450]
        tunnel: w2430 -> [w2449]
        tunnel: w2434 -> [w2448]
        tunnel: w2433 -> [w2447]
        tunnel: w2432 -> [w2446]
        tunnel: w2431 -> [w2445]
        stop <- w2456 stop-if-true
        n849 = Get Queue Status(queue=w2450) -> (queue out=w2458:refnum<queue>, # elements in queue=w2460:i32)  [unwired: 2 in, 6 out]
        n850 = Get Notifier Status(notifier=w2457) -> (current notification=w2456:bool)  [unwired: 1 in, 4 out]
        n851 = Greater Than 0?(x=w2460) -> (x > 0?=w2459:bool)
        n852 = case shown="True" w2459 {
          tunnel: w2466 -> [_ w2496]
          tunnel: w2465 -> [w2468 w2497]
          tunnel: [w2468 w2495] -> w2464
          tunnel: w2463 -> [_ w2494]
          tunnel: w2462 -> [_ w2493]
          tunnel: w2461 -> [_ w2483]
          tunnel: w2458 -> [_ w2492]
          tunnel: w2455 -> [w2467 w2489]
          tunnel: [w2467 w2488] -> w2454
          tunnel: w2453 -> [_ w2487]
          tunnel: w2452 -> [_ w2486]
          tunnel: w2451 -> [_ w2481]
          tunnel: w2449 -> [_ w2479]
          tunnel: w2448 -> [_ w2478]
          tunnel: w2447 -> [_ _]
          tunnel: w2446 -> [_ _]
          tunnel: w2445 -> [_ _]
          frame False {
          }
          frame True {
            # "True: Last Frame of frame accum"
            # "Current Line in Frame Accum"
            # "Current Line In Frame"
            n853 = Increment(x=w2489) -> (x+1=w2482:u32)
            n854 = Dequeue Element(queue=w2492) -> (element=w2502:u64[])  [unwired: 2 in, 3 out]
            n855 = Equal?(x=w2482, y=w2486) -> (x = y?=w2491:bool)
            n856 = Greater?(x=w2482, y=w2487) -> (0:w2484:bool)
            n857 = Greater?(x=w2482, y=w2481) -> (0:w2480:bool)
            n858 = Split Number(x=w2502) -> (hi(x)=w2503:u32[], lo(x)=w2501:u32[])
            n859 = Split Number(x=w2503) -> (lo(x)=w2473:u16[])  [unwired: 1 out]
            n860 = Split Number(x=w2501) -> (hi(x)=w2474:u16[])  [unwired: 1 out]
            n861 = Select(t=u32 0, s=w2491, f=w2482) -> (s? t:f=w2488:u32)
            n862 = Increment(x=w2497) -> (x+1=w2498:i32)
            n863 = Equal?(x=w2496, y=w2497) -> (x = y?=w2472:bool)
            n864 = To Single Precision Float(number=w2473) -> (single precision float=w2477:sgl[])
            n865 = To Single Precision Float(number=w2474) -> (single precision float=w2476:sgl[])
            n866 = Select(t=0, s=w2472, f=w2498) -> (s? t:f=w2495:i32)
            n867 = Add(x=w2477, y=w2476) -> (x+y=w2475:sgl[])
            n868 = Build Array(0, w2497, w2496, w2497) -> (w2469:i32[])
            n869 = case shown="False" w2480 {
              tunnel: [w2522 w2528] -> w2470
              tunnel: w2469 -> [_ w2526]
              tunnel: w2493 -> [w2521 w2525]
              tunnel: w2479 -> [w2520 w2524]
              tunnel: [w2520 w2524] -> w2471
              tunnel: w2475 -> [w2519 w2523]
              frame False {
                n870 = Divide(x=w2519, y=w2521) -> (x/y=w2522:sgl[])
              }
              frame True {
                n871 = call "IMAQ GetPixelLine"("Line Coordinates"=w2526, "Image"=w2524) -> ("Pixels Line (Float)"=w2527:sgl[])  [unwired: 2 in, 4 out]
                n872 = Divide(x=w2523, y=w2525) -> (x/y=w2529:sgl[])
                n873 = Add(x=w2527, y=w2529) -> (x+y=w2528:sgl[])
              }
            }
            n874 = stacked-sequence {
              tunnel: w2469 -> [w2506 _]
              tunnel: w2470 -> [w2505 _]
              tunnel: w2471 -> [w2504 _]
              tunnel: w2472 -> [_ w2510]
              frame #0 {
                n875 = call "IMAQ SetPixelLine"("Pixels Line (Float)"=w2505, "Line Coordinates"=w2506, "Image"=w2504) -> ()  [unwired: 7 in, 2 out]
              }
              frame #1 {
                n876 = case shown="True" w2510 {
                  tunnel: [w2511 w2513] -> w2508
                  frame False {
                    n877 = call "Frame Counter.vi"("Action"=Counter_Action."Read") -> ("Num"=w2511:i32)
                  }
                  frame True {
                    n878 = call "Frame Counter.vi"("Action"=Counter_Action."Plus One") -> ("Num"=w2513:i32)
                  }
                }
                n879 = call "FPGA-7842R-Control V2.vi"("Current Frame"=w2508, "Action"=FPGA-7842R-Reference."Current Frame for Capture", "Initialize"=TRUE) -> ()  [unwired: 11 in, 2 out]
              }
            }
            n880 = And(x=w2484, y=w2483) -> (x .and. y?=w2485:bool)
            n881 = case shown="True" w2485 {
              tunnel: w2470 -> [_ w2518]
              tunnel: w2494 -> [_ w2516]
              tunnel: w2478 -> [_ w2515]
              frame False {
              }
              frame True {
                n882 = Write to Binary File(file (use dialog)=w2515, data=w2518, 5:FALSE ("prepend array or string size? (T)"), 9:w2516) -> ()  [unwired: 2 in, 3 out]
              }
            }
          }
        }
      }
    }
    frame 23 {
      n883 = while {
        shift-right: [w2565] -> _
        shift-left: 0 -> [w2566]
        tunnel: w2544 -> [w2567]
        tunnel: w2543 -> [w2564]
        tunnel: w2542 -> [w2563]
        tunnel: w2541 -> [w2562]
        tunnel: w2530 -> [w2558]
        shift-right: [w2555] -> _
        shift-left: u32 0 -> [w2556]
        tunnel: w2539 -> [w2554]
        tunnel: w2538 -> [w2553]
        tunnel: w2537 -> [w2552]
        tunnel: w2536 -> [w2551]
        tunnel: w2531 -> [w2550]
        tunnel: w2535 -> [w2549]
        tunnel: w2534 -> [w2548]
        tunnel: w2533 -> [w2547]
        tunnel: w2532 -> [w2546]
        stop <- w2557 stop-if-true
        n884 = Get Queue Status(queue=w2551) -> (queue out=w2559:refnum<queue>, # elements in queue=w2561:i32)  [unwired: 2 in, 6 out]
        n885 = Get Notifier Status(notifier=w2558) -> (current notification=w2557:bool)  [unwired: 1 in, 4 out]
        n886 = Greater Than 0?(x=w2561) -> (x > 0?=w2560:bool)
        n887 = case shown="True" w2560 {
          tunnel: w2567 -> [_ w2599]
          tunnel: w2566 -> [w2569 w2600]
          tunnel: [w2569 w2598] -> w2565
          tunnel: w2564 -> [_ w2597]
          tunnel: w2563 -> [_ w2596]
          tunnel: w2562 -> [_ w2586]
          tunnel: w2559 -> [_ w2595]
          tunnel: w2556 -> [w2568 w2592]
          tunnel: [w2568 w2591] -> w2555
          tunnel: w2554 -> [_ w2590]
          tunnel: w2553 -> [_ w2589]
          tunnel: w2552 -> [_ w2584]
          tunnel: w2550 -> [_ w2582]
          tunnel: w2549 -> [_ w2581]
          tunnel: w2548 -> [_ _]
          tunnel: w2547 -> [_ _]
          tunnel: w2546 -> [_ _]
          frame False {
          }
          frame True {
            # "True: Last Frame of frame accum"
            # "Current Line in Frame Accum"
            # "Current Line In Frame"
            n888 = Increment(x=w2592) -> (x+1=w2585:u32)
            n889 = Dequeue Element(queue=w2595) -> (element=w2605:u64[])  [unwired: 2 in, 3 out]
            n890 = Equal?(x=w2585, y=w2589) -> (x = y?=w2594:bool)
            n891 = Greater?(x=w2585, y=w2590) -> (0:w2587:bool)
            n892 = Greater?(x=w2585, y=w2584) -> (0:w2583:bool)
            n893 = Split Number(x=w2605) -> (hi(x)=w2606:u32[], lo(x)=w2604:u32[])
            n894 = Split Number(x=w2606) -> (hi(x)=w2579:u16[], lo(x)=w2578:u16[])
            n895 = Split Number(x=w2604) -> (hi(x)=w2580:u16[])  [unwired: 1 out]
            n896 = Select(t=u32 0, s=w2594, f=w2585) -> (s? t:f=w2591:u32)
            n897 = Increment(x=w2600) -> (x+1=w2601:i32)
            n898 = Equal?(x=w2599, y=w2600) -> (x = y?=w2573:bool)
            n899 = To Single Precision Float(number=w2579) -> (single precision float=w2577:sgl[])
            n900 = To Single Precision Float(number=w2578) -> (single precision float=w2575:sgl[])
            n901 = To Single Precision Float(number=w2580) -> (single precision float=w2576:sgl[])
            n902 = Select(t=0, s=w2573, f=w2601) -> (s? t:f=w2598:i32)
            n903 = Compound Arithmetic op=ADD(w2577, w2575, w2576) -> (w2574:sgl[])
            n904 = Build Array(0, w2600, w2599, w2600) -> (w2570:i32[])
            n905 = case shown="False" w2583 {
              tunnel: [w2625 w2631] -> w2571
              tunnel: w2570 -> [_ w2629]
              tunnel: w2596 -> [w2624 w2628]
              tunnel: w2582 -> [w2623 w2627]
              tunnel: [w2623 w2627] -> w2572
              tunnel: w2574 -> [w2622 w2626]
              frame False {
                n906 = Divide(x=w2622, y=w2624) -> (x/y=w2625:sgl[])
              }
              frame True {
                n907 = call "IMAQ GetPixelLine"("Line Coordinates"=w2629, "Image"=w2627) -> ("Pixels Line (Float)"=w2630:sgl[])  [unwired: 2 in, 4 out]
                n908 = Divide(x=w2626, y=w2628) -> (x/y=w2632:sgl[])
                n909 = Add(x=w2630, y=w2632) -> (x+y=w2631:sgl[])
              }
            }
            n910 = stacked-sequence {
              tunnel: w2570 -> [w2609 _]
              tunnel: w2571 -> [w2608 _]
              tunnel: w2572 -> [w2607 _]
              tunnel: w2573 -> [_ w2613]
              frame #0 {
                n911 = call "IMAQ SetPixelLine"("Pixels Line (Float)"=w2608, "Line Coordinates"=w2609, "Image"=w2607) -> ()  [unwired: 7 in, 2 out]
              }
              frame #1 {
                n912 = case shown="True" w2613 {
                  tunnel: [w2614 w2616] -> w2611
                  frame False {
                    n913 = call "Frame Counter.vi"("Action"=Counter_Action."Read") -> ("Num"=w2614:i32)
                  }
                  frame True {
                    n914 = call "Frame Counter.vi"("Action"=Counter_Action."Plus One") -> ("Num"=w2616:i32)
                  }
                }
                n915 = call "FPGA-7842R-Control V2.vi"("Current Frame"=w2611, "Action"=FPGA-7842R-Reference."Current Frame for Capture", "Initialize"=TRUE) -> ()  [unwired: 11 in, 2 out]
              }
            }
            n916 = And(x=w2587, y=w2586) -> (x .and. y?=w2588:bool)
            n917 = case shown="True" w2588 {
              tunnel: w2571 -> [_ w2621]
              tunnel: w2597 -> [_ w2619]
              tunnel: w2581 -> [_ w2618]
              frame False {
              }
              frame True {
                n918 = Write to Binary File(file (use dialog)=w2618, data=w2621, 5:FALSE ("prepend array or string size? (T)"), 9:w2619) -> ()  [unwired: 2 in, 3 out]
              }
            }
          }
        }
      }
    }
    frame 25 {
      n919 = while {
        shift-right: [w2668] -> _
        shift-left: 0 -> [w2669]
        tunnel: w2647 -> [w2670]
        tunnel: w2646 -> [w2667]
        tunnel: w2645 -> [w2666]
        tunnel: w2644 -> [w2665]
        tunnel: w2633 -> [w2661]
        shift-right: [w2658] -> _
        shift-left: u32 0 -> [w2659]
        tunnel: w2642 -> [w2657]
        tunnel: w2641 -> [w2656]
        tunnel: w2640 -> [w2655]
        tunnel: w2639 -> [w2654]
        tunnel: w2634 -> [w2653]
        tunnel: w2638 -> [w2652]
        tunnel: w2637 -> [w2651]
        tunnel: w2636 -> [w2650]
        tunnel: w2635 -> [w2649]
        stop <- w2660 stop-if-true
        n920 = Get Queue Status(queue=w2654) -> (queue out=w2662:refnum<queue>, # elements in queue=w2664:i32)  [unwired: 2 in, 6 out]
        n921 = Get Notifier Status(notifier=w2661) -> (current notification=w2660:bool)  [unwired: 1 in, 4 out]
        n922 = Greater Than 0?(x=w2664) -> (x > 0?=w2663:bool)
        n923 = case shown="True" w2663 {
          tunnel: w2670 -> [_ w2700]
          tunnel: w2669 -> [w2672 w2701]
          tunnel: [w2672 w2699] -> w2668
          tunnel: w2667 -> [_ w2698]
          tunnel: w2666 -> [_ w2697]
          tunnel: w2665 -> [_ w2687]
          tunnel: w2662 -> [_ w2696]
          tunnel: w2659 -> [w2671 w2693]
          tunnel: [w2671 w2692] -> w2658
          tunnel: w2657 -> [_ w2691]
          tunnel: w2656 -> [_ w2690]
          tunnel: w2655 -> [_ w2685]
          tunnel: w2653 -> [_ w2683]
          tunnel: w2652 -> [_ w2682]
          tunnel: w2651 -> [_ _]
          tunnel: w2650 -> [_ _]
          tunnel: w2649 -> [_ _]
          frame False {
          }
          frame True {
            # "True: Last Frame of frame accum"
            # "Current Line in Frame Accum"
            # "Current Line In Frame"
            n924 = Increment(x=w2693) -> (x+1=w2686:u32)
            n925 = Dequeue Element(queue=w2696) -> (element=w2706:u64[])  [unwired: 2 in, 3 out]
            n926 = Equal?(x=w2686, y=w2690) -> (x = y?=w2695:bool)
            n927 = Greater?(x=w2686, y=w2691) -> (0:w2688:bool)
            n928 = Greater?(x=w2686, y=w2685) -> (0:w2684:bool)
            n929 = Split Number(x=w2706) -> (hi(x)=w2707:u32[], lo(x)=w2705:u32[])
            n930 = Split Number(x=w2707) -> (hi(x)=w2677:u16[])  [unwired: 1 out]
            n931 = Split Number(x=w2705) -> (lo(x)=w2678:u16[])  [unwired: 1 out]
            n932 = Select(t=u32 0, s=w2695, f=w2686) -> (s? t:f=w2692:u32)
            n933 = Increment(x=w2701) -> (x+1=w2702:i32)
            n934 = Equal?(x=w2700, y=w2701) -> (x = y?=w2676:bool)
            n935 = To Single Precision Float(number=w2677) -> (single precision float=w2681:sgl[])
            n936 = To Single Precision Float(number=w2678) -> (single precision float=w2680:sgl[])
            n937 = Select(t=0, s=w2676, f=w2702) -> (s? t:f=w2699:i32)
            n938 = Add(x=w2681, y=w2680) -> (x+y=w2679:sgl[])
            n939 = Build Array(0, w2701, w2700, w2701) -> (w2673:i32[])
            n940 = case shown="False" w2684 {
              tunnel: [w2726 w2732] -> w2674
              tunnel: w2673 -> [_ w2730]
              tunnel: w2697 -> [w2725 w2729]
              tunnel: w2683 -> [w2724 w2728]
              tunnel: [w2724 w2728] -> w2675
              tunnel: w2679 -> [w2723 w2727]
              frame False {
                n941 = Divide(x=w2723, y=w2725) -> (x/y=w2726:sgl[])
              }
              frame True {
                n942 = call "IMAQ GetPixelLine"("Line Coordinates"=w2730, "Image"=w2728) -> ("Pixels Line (Float)"=w2731:sgl[])  [unwired: 2 in, 4 out]
                n943 = Divide(x=w2727, y=w2729) -> (x/y=w2733:sgl[])
                n944 = Add(x=w2731, y=w2733) -> (x+y=w2732:sgl[])
              }
            }
            n945 = stacked-sequence {
              tunnel: w2673 -> [w2710 _]
              tunnel: w2674 -> [w2709 _]
              tunnel: w2675 -> [w2708 _]
              tunnel: w2676 -> [_ w2714]
              frame #0 {
                n946 = call "IMAQ SetPixelLine"("Pixels Line (Float)"=w2709, "Line Coordinates"=w2710, "Image"=w2708) -> ()  [unwired: 7 in, 2 out]
              }
              frame #1 {
                n947 = case shown="True" w2714 {
                  tunnel: [w2715 w2717] -> w2712
                  frame False {
                    n948 = call "Frame Counter.vi"("Action"=Counter_Action."Read") -> ("Num"=w2715:i32)
                  }
                  frame True {
                    n949 = call "Frame Counter.vi"("Action"=Counter_Action."Plus One") -> ("Num"=w2717:i32)
                  }
                }
                n950 = call "FPGA-7842R-Control V2.vi"("Current Frame"=w2712, "Action"=FPGA-7842R-Reference."Current Frame for Capture", "Initialize"=TRUE) -> ()  [unwired: 11 in, 2 out]
              }
            }
            n951 = And(x=w2688, y=w2687) -> (x .and. y?=w2689:bool)
            n952 = case shown="True" w2689 {
              tunnel: w2674 -> [_ w2722]
              tunnel: w2698 -> [_ w2720]
              tunnel: w2682 -> [_ w2719]
              frame False {
              }
              frame True {
                n953 = Write to Binary File(file (use dialog)=w2719, data=w2722, 5:FALSE ("prepend array or string size? (T)"), 9:w2720) -> ()  [unwired: 2 in, 3 out]
              }
            }
          }
        }
      }
    }
    frame 26 {
      n954 = while {
        shift-right: [w2769] -> _
        shift-left: 0 -> [w2770]
        tunnel: w2748 -> [w2771]
        tunnel: w2747 -> [w2768]
        tunnel: w2746 -> [w2767]
        tunnel: w2745 -> [w2766]
        tunnel: w2734 -> [w2762]
        shift-right: [w2759] -> _
        shift-left: u32 0 -> [w2760]
        tunnel: w2743 -> [w2758]
        tunnel: w2742 -> [w2757]
        tunnel: w2741 -> [w2756]
        tunnel: w2740 -> [w2755]
        tunnel: w2735 -> [w2754]
        tunnel: w2739 -> [w2753]
        tunnel: w2738 -> [w2752]
        tunnel: w2737 -> [w2751]
        tunnel: w2736 -> [w2750]
        stop <- w2761 stop-if-true
        n955 = Get Queue Status(queue=w2755) -> (queue out=w2763:refnum<queue>, # elements in queue=w2765:i32)  [unwired: 2 in, 6 out]
        n956 = Get Notifier Status(notifier=w2762) -> (current notification=w2761:bool)  [unwired: 1 in, 4 out]
        n957 = Greater Than 0?(x=w2765) -> (x > 0?=w2764:bool)
        n958 = case shown="True" w2764 {
          tunnel: w2771 -> [_ w2801]
          tunnel: w2770 -> [w2773 w2802]
          tunnel: [w2773 w2800] -> w2769
          tunnel: w2768 -> [_ w2799]
          tunnel: w2767 -> [_ w2798]
          tunnel: w2766 -> [_ w2788]
          tunnel: w2763 -> [_ w2797]
          tunnel: w2760 -> [w2772 w2794]
          tunnel: [w2772 w2793] -> w2759
          tunnel: w2758 -> [_ w2792]
          tunnel: w2757 -> [_ w2791]
          tunnel: w2756 -> [_ w2786]
          tunnel: w2754 -> [_ w2784]
          tunnel: w2753 -> [_ w2783]
          tunnel: w2752 -> [_ _]
          tunnel: w2751 -> [_ _]
          tunnel: w2750 -> [_ _]
          frame False {
          }
          frame True {
            # "True: Last Frame of frame accum"
            # "Current Line in Frame Accum"
            # "Current Line In Frame"
            n959 = Increment(x=w2794) -> (x+1=w2787:u32)
            n960 = Dequeue Element(queue=w2797) -> (element=w2807:u64[])  [unwired: 2 in, 3 out]
            n961 = Equal?(x=w2787, y=w2791) -> (x = y?=w2796:bool)
            n962 = Greater?(x=w2787, y=w2792) -> (0:w2789:bool)
            n963 = Greater?(x=w2787, y=w2786) -> (0:w2785:bool)
            n964 = Split Number(x=w2807) -> (hi(x)=w2808:u32[], lo(x)=w2806:u32[])
            n965 = Split Number(x=w2808) -> (lo(x)=w2779:u16[])  [unwired: 1 out]
            n966 = Split Number(x=w2806) -> (lo(x)=w2778:u16[])  [unwired: 1 out]
            n967 = Select(t=u32 0, s=w2796, f=w2787) -> (s? t:f=w2793:u32)
            n968 = Increment(x=w2802) -> (x+1=w2803:i32)
            n969 = Equal?(x=w2801, y=w2802) -> (x = y?=w2777:bool)
            n970 = To Single Precision Float(number=w2779) -> (single precision float=w2782:sgl[])
            n971 = To Single Precision Float(number=w2778) -> (single precision float=w2781:sgl[])
            n972 = Select(t=0, s=w2777, f=w2803) -> (s? t:f=w2800:i32)
            n973 = Add(x=w2782, y=w2781) -> (x+y=w2780:sgl[])
            n974 = Build Array(0, w2802, w2801, w2802) -> (w2774:i32[])
            n975 = case shown="False" w2785 {
              tunnel: [w2827 w2833] -> w2775
              tunnel: w2774 -> [_ w2831]
              tunnel: w2798 -> [w2826 w2830]
              tunnel: w2784 -> [w2825 w2829]
              tunnel: [w2825 w2829] -> w2776
              tunnel: w2780 -> [w2824 w2828]
              frame False {
                n976 = Divide(x=w2824, y=w2826) -> (x/y=w2827:sgl[])
              }
              frame True {
                n977 = call "IMAQ GetPixelLine"("Line Coordinates"=w2831, "Image"=w2829) -> ("Pixels Line (Float)"=w2832:sgl[])  [unwired: 2 in, 4 out]
                n978 = Divide(x=w2828, y=w2830) -> (x/y=w2834:sgl[])
                n979 = Add(x=w2832, y=w2834) -> (x+y=w2833:sgl[])
              }
            }
            n980 = stacked-sequence {
              tunnel: w2774 -> [w2811 _]
              tunnel: w2775 -> [w2810 _]
              tunnel: w2776 -> [w2809 _]
              tunnel: w2777 -> [_ w2815]
              frame #0 {
                n981 = call "IMAQ SetPixelLine"("Pixels Line (Float)"=w2810, "Line Coordinates"=w2811, "Image"=w2809) -> ()  [unwired: 7 in, 2 out]
              }
              frame #1 {
                n982 = case shown="True" w2815 {
                  tunnel: [w2816 w2818] -> w2813
                  frame False {
                    n983 = call "Frame Counter.vi"("Action"=Counter_Action."Read") -> ("Num"=w2816:i32)
                  }
                  frame True {
                    n984 = call "Frame Counter.vi"("Action"=Counter_Action."Plus One") -> ("Num"=w2818:i32)
                  }
                }
                n985 = call "FPGA-7842R-Control V2.vi"("Current Frame"=w2813, "Action"=FPGA-7842R-Reference."Current Frame for Capture", "Initialize"=TRUE) -> ()  [unwired: 11 in, 2 out]
              }
            }
            n986 = And(x=w2789, y=w2788) -> (x .and. y?=w2790:bool)
            n987 = case shown="True" w2790 {
              tunnel: w2775 -> [_ w2823]
              tunnel: w2799 -> [_ w2821]
              tunnel: w2783 -> [_ w2820]
              frame False {
              }
              frame True {
                n988 = Write to Binary File(file (use dialog)=w2820, data=w2823, 5:FALSE ("prepend array or string size? (T)"), 9:w2821) -> ()  [unwired: 2 in, 3 out]
              }
            }
          }
        }
      }
    }
    frame 27 {
      n989 = while {
        shift-right: [w2870] -> _
        shift-left: 0 -> [w2871]
        tunnel: w2849 -> [w2872]
        tunnel: w2848 -> [w2869]
        tunnel: w2847 -> [w2868]
        tunnel: w2846 -> [w2867]
        tunnel: w2835 -> [w2863]
        shift-right: [w2860] -> _
        shift-left: u32 0 -> [w2861]
        tunnel: w2844 -> [w2859]
        tunnel: w2843 -> [w2858]
        tunnel: w2842 -> [w2857]
        tunnel: w2841 -> [w2856]
        tunnel: w2836 -> [w2855]
        tunnel: w2840 -> [w2854]
        tunnel: w2839 -> [w2853]
        tunnel: w2838 -> [w2852]
        tunnel: w2837 -> [w2851]
        stop <- w2862 stop-if-true
        n990 = Get Queue Status(queue=w2856) -> (queue out=w2864:refnum<queue>, # elements in queue=w2866:i32)  [unwired: 2 in, 6 out]
        n991 = Get Notifier Status(notifier=w2863) -> (current notification=w2862:bool)  [unwired: 1 in, 4 out]
        n992 = Greater Than 0?(x=w2866) -> (x > 0?=w2865:bool)
        n993 = case shown="True" w2865 {
          tunnel: w2872 -> [_ w2904]
          tunnel: w2871 -> [w2874 w2905]
          tunnel: [w2874 w2903] -> w2870
          tunnel: w2869 -> [_ w2902]
          tunnel: w2868 -> [_ w2901]
          tunnel: w2867 -> [_ w2891]
          tunnel: w2864 -> [_ w2900]
          tunnel: w2861 -> [w2873 w2897]
          tunnel: [w2873 w2896] -> w2860
          tunnel: w2859 -> [_ w2895]
          tunnel: w2858 -> [_ w2894]
          tunnel: w2857 -> [_ w2889]
          tunnel: w2855 -> [_ w2887]
          tunnel: w2854 -> [_ w2886]
          tunnel: w2853 -> [_ _]
          tunnel: w2852 -> [_ _]
          tunnel: w2851 -> [_ _]
          frame False {
          }
          frame True {
            # "True: Last Frame of frame accum"
            # "Current Line in Frame Accum"
            # "Current Line In Frame"
            n994 = Increment(x=w2897) -> (x+1=w2890:u32)
            n995 = Dequeue Element(queue=w2900) -> (element=w2910:u64[])  [unwired: 2 in, 3 out]
            n996 = Equal?(x=w2890, y=w2894) -> (x = y?=w2899:bool)
            n997 = Greater?(x=w2890, y=w2895) -> (0:w2892:bool)
            n998 = Greater?(x=w2890, y=w2889) -> (0:w2888:bool)
            n999 = Split Number(x=w2910) -> (hi(x)=w2911:u32[], lo(x)=w2909:u32[])
            n1000 = Split Number(x=w2911) -> (hi(x)=w2885:u16[], lo(x)=w2884:u16[])
            n1001 = Split Number(x=w2909) -> (lo(x)=w2879:u16[])  [unwired: 1 out]
            n1002 = Select(t=u32 0, s=w2899, f=w2890) -> (s? t:f=w2896:u32)
            n1003 = Increment(x=w2905) -> (x+1=w2906:i32)
            n1004 = Equal?(x=w2904, y=w2905) -> (x = y?=w2878:bool)
            n1005 = To Single Precision Float(number=w2885) -> (single precision float=w2883:sgl[])
            n1006 = To Single Precision Float(number=w2884) -> (single precision float=w2881:sgl[])
            n1007 = To Single Precision Float(number=w2879) -> (single precision float=w2882:sgl[])
            n1008 = Select(t=0, s=w2878, f=w2906) -> (s? t:f=w2903:i32)
            n1009 = Compound Arithmetic op=ADD(w2883, w2881, w2882) -> (w2880:sgl[])
            n1010 = Build Array(0, w2905, w2904, w2905) -> (w2877:i32[])
            n1011 = case shown="False" w2888 {
              tunnel: [w2930 w2936] -> w2875
              tunnel: w2877 -> [_ w2934]
              tunnel: w2901 -> [w2929 w2933]
              tunnel: w2887 -> [w2928 w2932]
              tunnel: [w2928 w2932] -> w2876
              tunnel: w2880 -> [w2927 w2931]
              frame False {
                n1012 = Divide(x=w2927, y=w2929) -> (x/y=w2930:sgl[])
              }
              frame True {
                n1013 = call "IMAQ GetPixelLine"("Line Coordinates"=w2934, "Image"=w2932) -> ("Pixels Line (Float)"=w2935:sgl[])  [unwired: 2 in, 4 out]
                n1014 = Divide(x=w2931, y=w2933) -> (x/y=w2937:sgl[])
                n1015 = Add(x=w2935, y=w2937) -> (x+y=w2936:sgl[])
              }
            }
            n1016 = stacked-sequence {
              tunnel: w2877 -> [w2914 _]
              tunnel: w2875 -> [w2913 _]
              tunnel: w2876 -> [w2912 _]
              tunnel: w2878 -> [_ w2918]
              frame #0 {
                n1017 = call "IMAQ SetPixelLine"("Pixels Line (Float)"=w2913, "Line Coordinates"=w2914, "Image"=w2912) -> ()  [unwired: 7 in, 2 out]
              }
              frame #1 {
                n1018 = case shown="True" w2918 {
                  tunnel: [w2919 w2921] -> w2916
                  frame False {
                    n1019 = call "Frame Counter.vi"("Action"=Counter_Action."Read") -> ("Num"=w2919:i32)
                  }
                  frame True {
                    n1020 = call "Frame Counter.vi"("Action"=Counter_Action."Plus One") -> ("Num"=w2921:i32)
                  }
                }
                n1021 = call "FPGA-7842R-Control V2.vi"("Current Frame"=w2916, "Action"=FPGA-7842R-Reference."Current Frame for Capture", "Initialize"=TRUE) -> ()  [unwired: 11 in, 2 out]
              }
            }
            n1022 = And(x=w2892, y=w2891) -> (x .and. y?=w2893:bool)
            n1023 = case shown="True" w2893 {
              tunnel: w2875 -> [_ w2926]
              tunnel: w2902 -> [_ w2924]
              tunnel: w2886 -> [_ w2923]
              frame False {
              }
              frame True {
                n1024 = Write to Binary File(file (use dialog)=w2923, data=w2926, 5:FALSE ("prepend array or string size? (T)"), 9:w2924) -> ()  [unwired: 2 in, 3 out]
              }
            }
          }
        }
      }
    }
    frame 28 {
      n1025 = while {
        shift-right: [w2973] -> _
        shift-left: 0 -> [w2974]
        tunnel: w2952 -> [w2975]
        tunnel: w2951 -> [w2972]
        tunnel: w2950 -> [w2971]
        tunnel: w2949 -> [w2970]
        tunnel: w2938 -> [w2966]
        shift-right: [w2963] -> _
        shift-left: u32 0 -> [w2964]
        tunnel: w2947 -> [w2962]
        tunnel: w2946 -> [w2961]
        tunnel: w2945 -> [w2960]
        tunnel: w2944 -> [w2959]
        tunnel: w2939 -> [w2958]
        tunnel: w2943 -> [w2957]
        tunnel: w2942 -> [w2956]
        tunnel: w2941 -> [w2955]
        tunnel: w2940 -> [w2954]
        stop <- w2965 stop-if-true
        n1026 = Get Queue Status(queue=w2959) -> (queue out=w2967:refnum<queue>, # elements in queue=w2969:i32)  [unwired: 2 in, 6 out]
        n1027 = Get Notifier Status(notifier=w2966) -> (current notification=w2965:bool)  [unwired: 1 in, 4 out]
        n1028 = Greater Than 0?(x=w2969) -> (x > 0?=w2968:bool)
        n1029 = case shown="True" w2968 {
          tunnel: w2975 -> [_ w3005]
          tunnel: w2974 -> [w2977 w3006]
          tunnel: [w2977 w3004] -> w2973
          tunnel: w2972 -> [_ w3003]
          tunnel: w2971 -> [_ w3002]
          tunnel: w2970 -> [_ w2992]
          tunnel: w2967 -> [_ w3001]
          tunnel: w2964 -> [w2976 w2998]
          tunnel: [w2976 w2997] -> w2963
          tunnel: w2962 -> [_ w2996]
          tunnel: w2961 -> [_ w2995]
          tunnel: w2960 -> [_ w2990]
          tunnel: w2958 -> [_ w2988]
          tunnel: w2957 -> [_ w2987]
          tunnel: w2956 -> [_ _]
          tunnel: w2955 -> [_ _]
          tunnel: w2954 -> [_ _]
          frame False {
          }
          frame True {
            # "True: Last Frame of frame accum"
            # "Current Line in Frame Accum"
            # "Current Line In Frame"
            n1030 = Increment(x=w2998) -> (x+1=w2991:u32)
            n1031 = Dequeue Element(queue=w3001) -> (element=w3011:u64[])  [unwired: 2 in, 3 out]
            n1032 = Equal?(x=w2991, y=w2995) -> (x = y?=w3000:bool)
            n1033 = Greater?(x=w2991, y=w2996) -> (0:w2993:bool)
            n1034 = Greater?(x=w2991, y=w2990) -> (0:w2989:bool)
            n1035 = Split Number(x=w3011) -> (lo(x)=w3010:u32[])  [unwired: 1 out]
            n1036 = Split Number(x=w3010) -> (hi(x)=w2982:u16[], lo(x)=w2983:u16[])
            n1037 = Select(t=u32 0, s=w3000, f=w2991) -> (s? t:f=w2997:u32)
            n1038 = Increment(x=w3006) -> (x+1=w3007:i32)
            n1039 = Equal?(x=w3005, y=w3006) -> (x = y?=w2981:bool)
            n1040 = To Single Precision Float(number=w2982) -> (single precision float=w2986:sgl[])
            n1041 = To Single Precision Float(number=w2983) -> (single precision float=w2985:sgl[])
            n1042 = Select(t=0, s=w2981, f=w3007) -> (s? t:f=w3004:i32)
            n1043 = Add(x=w2986, y=w2985) -> (x+y=w2984:sgl[])
            n1044 = Build Array(0, w3006, w3005, w3006) -> (w2980:i32[])
            n1045 = case shown="False" w2989 {
              tunnel: [w3030 w3036] -> w2978
              tunnel: w2980 -> [_ w3034]
              tunnel: w3002 -> [w3029 w3033]
              tunnel: w2988 -> [w3028 w3032]
              tunnel: [w3028 w3032] -> w2979
              tunnel: w2984 -> [w3027 w3031]
              frame False {
                n1046 = Divide(x=w3027, y=w3029) -> (x/y=w3030:sgl[])
              }
              frame True {
                n1047 = call "IMAQ GetPixelLine"("Line Coordinates"=w3034, "Image"=w3032) -> ("Pixels Line (Float)"=w3035:sgl[])  [unwired: 2 in, 4 out]
                n1048 = Divide(x=w3031, y=w3033) -> (x/y=w3037:sgl[])
                n1049 = Add(x=w3035, y=w3037) -> (x+y=w3036:sgl[])
              }
            }
            n1050 = stacked-sequence {
              tunnel: w2980 -> [w3014 _]
              tunnel: w2978 -> [w3013 _]
              tunnel: w2979 -> [w3012 _]
              tunnel: w2981 -> [_ w3018]
              frame #0 {
                n1051 = call "IMAQ SetPixelLine"("Pixels Line (Float)"=w3013, "Line Coordinates"=w3014, "Image"=w3012) -> ()  [unwired: 7 in, 2 out]
              }
              frame #1 {
                n1052 = case shown="True" w3018 {
                  tunnel: [w3019 w3021] -> w3016
                  frame False {
                    n1053 = call "Frame Counter.vi"("Action"=Counter_Action."Read") -> ("Num"=w3019:i32)
                  }
                  frame True {
                    n1054 = call "Frame Counter.vi"("Action"=Counter_Action."Plus One") -> ("Num"=w3021:i32)
                  }
                }
                n1055 = call "FPGA-7842R-Control V2.vi"("Current Frame"=w3016, "Action"=FPGA-7842R-Reference."Current Frame for Capture", "Initialize"=TRUE) -> ()  [unwired: 11 in, 2 out]
              }
            }
            n1056 = And(x=w2993, y=w2992) -> (x .and. y?=w2994:bool)
            n1057 = case shown="True" w2994 {
              tunnel: w2978 -> [_ w3026]
              tunnel: w3003 -> [_ w3024]
              tunnel: w2987 -> [_ w3023]
              frame False {
              }
              frame True {
                n1058 = Write to Binary File(file (use dialog)=w3023, data=w3026, 5:FALSE ("prepend array or string size? (T)"), 9:w3024) -> ()  [unwired: 2 in, 3 out]
              }
            }
          }
        }
      }
    }
    frame 29 {
      n1059 = while {
        shift-right: [w3073] -> _
        shift-left: 0 -> [w3074]
        tunnel: w3052 -> [w3075]
        tunnel: w3051 -> [w3072]
        tunnel: w3050 -> [w3071]
        tunnel: w3049 -> [w3070]
        tunnel: w3038 -> [w3066]
        shift-right: [w3063] -> _
        shift-left: u32 0 -> [w3064]
        tunnel: w3047 -> [w3062]
        tunnel: w3046 -> [w3061]
        tunnel: w3045 -> [w3060]
        tunnel: w3044 -> [w3059]
        tunnel: w3039 -> [w3058]
        tunnel: w3043 -> [w3057]
        tunnel: w3042 -> [w3056]
        tunnel: w3041 -> [w3055]
        tunnel: w3040 -> [w3054]
        stop <- w3065 stop-if-true
        n1060 = Get Queue Status(queue=w3059) -> (queue out=w3067:refnum<queue>, # elements in queue=w3069:i32)  [unwired: 2 in, 6 out]
        n1061 = Get Notifier Status(notifier=w3066) -> (current notification=w3065:bool)  [unwired: 1 in, 4 out]
        n1062 = Greater Than 0?(x=w3069) -> (x > 0?=w3068:bool)
        n1063 = case shown="True" w3068 {
          tunnel: w3075 -> [_ w3107]
          tunnel: w3074 -> [w3077 w3108]
          tunnel: [w3077 w3106] -> w3073
          tunnel: w3072 -> [_ w3105]
          tunnel: w3071 -> [_ w3104]
          tunnel: w3070 -> [_ w3094]
          tunnel: w3067 -> [_ w3103]
          tunnel: w3064 -> [w3076 w3100]
          tunnel: [w3076 w3099] -> w3063
          tunnel: w3062 -> [_ w3098]
          tunnel: w3061 -> [_ w3097]
          tunnel: w3060 -> [_ w3092]
          tunnel: w3058 -> [_ w3090]
          tunnel: w3057 -> [_ w3089]
          tunnel: w3056 -> [_ _]
          tunnel: w3055 -> [_ _]
          tunnel: w3054 -> [_ _]
          frame False {
          }
          frame True {
            # "True: Last Frame of frame accum"
            # "Current Line in Frame Accum"
            # "Current Line In Frame"
            n1064 = Increment(x=w3100) -> (x+1=w3093:u32)
            n1065 = Dequeue Element(queue=w3103) -> (element=w3113:u64[])  [unwired: 2 in, 3 out]
            n1066 = Equal?(x=w3093, y=w3097) -> (x = y?=w3102:bool)
            n1067 = Greater?(x=w3093, y=w3098) -> (0:w3095:bool)
            n1068 = Greater?(x=w3093, y=w3092) -> (0:w3091:bool)
            n1069 = Split Number(x=w3113) -> (hi(x)=w3114:u32[], lo(x)=w3112:u32[])
            n1070 = Split Number(x=w3114) -> (hi(x)=w3088:u16[])  [unwired: 1 out]
            n1071 = Split Number(x=w3112) -> (hi(x)=w3083:u16[], lo(x)=w3082:u16[])
            n1072 = Select(t=u32 0, s=w3102, f=w3093) -> (s? t:f=w3099:u32)
            n1073 = Increment(x=w3108) -> (x+1=w3109:i32)
            n1074 = Equal?(x=w3107, y=w3108) -> (x = y?=w3081:bool)
            n1075 = To Single Precision Float(number=w3088) -> (single precision float=w3087:sgl[])
            n1076 = To Single Precision Float(number=w3083) -> (single precision float=w3085:sgl[])
            n1077 = To Single Precision Float(number=w3082) -> (single precision float=w3086:sgl[])
            n1078 = Select(t=0, s=w3081, f=w3109) -> (s? t:f=w3106:i32)
            n1079 = Compound Arithmetic op=ADD(w3087, w3085, w3086) -> (w3084:sgl[])
            n1080 = Build Array(0, w3108, w3107, w3108) -> (w3080:i32[])
            n1081 = case shown="False" w3091 {
              tunnel: [w3133 w3139] -> w3078
              tunnel: w3080 -> [_ w3137]
              tunnel: w3104 -> [w3132 w3136]
              tunnel: w3090 -> [w3131 w3135]
              tunnel: [w3131 w3135] -> w3079
              tunnel: w3084 -> [w3130 w3134]
              frame False {
                n1082 = Divide(x=w3130, y=w3132) -> (x/y=w3133:sgl[])
              }
              frame True {
                n1083 = call "IMAQ GetPixelLine"("Line Coordinates"=w3137, "Image"=w3135) -> ("Pixels Line (Float)"=w3138:sgl[])  [unwired: 2 in, 4 out]
                n1084 = Divide(x=w3134, y=w3136) -> (x/y=w3140:sgl[])
                n1085 = Add(x=w3138, y=w3140) -> (x+y=w3139:sgl[])
              }
            }
            n1086 = stacked-sequence {
              tunnel: w3080 -> [w3117 _]
              tunnel: w3078 -> [w3116 _]
              tunnel: w3079 -> [w3115 _]
              tunnel: w3081 -> [_ w3121]
              frame #0 {
                n1087 = call "IMAQ SetPixelLine"("Pixels Line (Float)"=w3116, "Line Coordinates"=w3117, "Image"=w3115) -> ()  [unwired: 7 in, 2 out]
              }
              frame #1 {
                n1088 = case shown="True" w3121 {
                  tunnel: [w3122 w3124] -> w3119
                  frame False {
                    n1089 = call "Frame Counter.vi"("Action"=Counter_Action."Read") -> ("Num"=w3122:i32)
                  }
                  frame True {
                    n1090 = call "Frame Counter.vi"("Action"=Counter_Action."Plus One") -> ("Num"=w3124:i32)
                  }
                }
                n1091 = call "FPGA-7842R-Control V2.vi"("Current Frame"=w3119, "Action"=FPGA-7842R-Reference."Current Frame for Capture", "Initialize"=TRUE) -> ()  [unwired: 11 in, 2 out]
              }
            }
            n1092 = And(x=w3095, y=w3094) -> (x .and. y?=w3096:bool)
            n1093 = case shown="True" w3096 {
              tunnel: w3078 -> [_ w3129]
              tunnel: w3105 -> [_ w3127]
              tunnel: w3089 -> [_ w3126]
              frame False {
              }
              frame True {
                n1094 = Write to Binary File(file (use dialog)=w3126, data=w3129, 5:FALSE ("prepend array or string size? (T)"), 9:w3127) -> ()  [unwired: 2 in, 3 out]
              }
            }
          }
        }
      }
    }
    frame 30 {
      n1095 = while {
        shift-right: [w3176] -> _
        shift-left: 0 -> [w3177]
        tunnel: w3155 -> [w3178]
        tunnel: w3154 -> [w3175]
        tunnel: w3153 -> [w3174]
        tunnel: w3152 -> [w3173]
        tunnel: w3141 -> [w3169]
        shift-right: [w3166] -> _
        shift-left: u32 0 -> [w3167]
        tunnel: w3150 -> [w3165]
        tunnel: w3149 -> [w3164]
        tunnel: w3148 -> [w3163]
        tunnel: w3147 -> [w3162]
        tunnel: w3142 -> [w3161]
        tunnel: w3146 -> [w3160]
        tunnel: w3145 -> [w3159]
        tunnel: w3144 -> [w3158]
        tunnel: w3143 -> [w3157]
        stop <- w3168 stop-if-true
        n1096 = Get Queue Status(queue=w3162) -> (queue out=w3170:refnum<queue>, # elements in queue=w3172:i32)  [unwired: 2 in, 6 out]
        n1097 = Get Notifier Status(notifier=w3169) -> (current notification=w3168:bool)  [unwired: 1 in, 4 out]
        n1098 = Greater Than 0?(x=w3172) -> (x > 0?=w3171:bool)
        n1099 = case shown="True" w3171 {
          tunnel: w3178 -> [_ w3210]
          tunnel: w3177 -> [w3180 w3211]
          tunnel: [w3180 w3209] -> w3176
          tunnel: w3175 -> [_ w3208]
          tunnel: w3174 -> [_ w3207]
          tunnel: w3173 -> [_ w3197]
          tunnel: w3170 -> [_ w3206]
          tunnel: w3167 -> [w3179 w3203]
          tunnel: [w3179 w3202] -> w3166
          tunnel: w3165 -> [_ w3201]
          tunnel: w3164 -> [_ w3200]
          tunnel: w3163 -> [_ w3195]
          tunnel: w3161 -> [_ w3193]
          tunnel: w3160 -> [_ w3192]
          tunnel: w3159 -> [_ _]
          tunnel: w3158 -> [_ _]
          tunnel: w3157 -> [_ _]
          frame False {
          }
          frame True {
            # "True: Last Frame of frame accum"
            # "Current Line in Frame Accum"
            # "Current Line In Frame"
            n1100 = Increment(x=w3203) -> (x+1=w3196:u32)
            n1101 = Dequeue Element(queue=w3206) -> (element=w3216:u64[])  [unwired: 2 in, 3 out]
            n1102 = Equal?(x=w3196, y=w3200) -> (x = y?=w3205:bool)
            n1103 = Greater?(x=w3196, y=w3201) -> (0:w3198:bool)
            n1104 = Greater?(x=w3196, y=w3195) -> (0:w3194:bool)
            n1105 = Split Number(x=w3216) -> (hi(x)=w3217:u32[], lo(x)=w3215:u32[])
            n1106 = Split Number(x=w3217) -> (lo(x)=w3185:u16[])  [unwired: 1 out]
            n1107 = Split Number(x=w3215) -> (hi(x)=w3187:u16[], lo(x)=w3186:u16[])
            n1108 = Select(t=u32 0, s=w3205, f=w3196) -> (s? t:f=w3202:u32)
            n1109 = Increment(x=w3211) -> (x+1=w3212:i32)
            n1110 = Equal?(x=w3210, y=w3211) -> (x = y?=w3184:bool)
            n1111 = To Single Precision Float(number=w3185) -> (single precision float=w3191:sgl[])
            n1112 = To Single Precision Float(number=w3187) -> (single precision float=w3189:sgl[])
            n1113 = To Single Precision Float(number=w3186) -> (single precision float=w3190:sgl[])
            n1114 = Select(t=0, s=w3184, f=w3212) -> (s? t:f=w3209:i32)
            n1115 = Compound Arithmetic op=ADD(w3191, w3189, w3190) -> (w3188:sgl[])
            n1116 = Build Array(0, w3211, w3210, w3211) -> (w3183:i32[])
            n1117 = case shown="False" w3194 {
              tunnel: [w3236 w3242] -> w3181
              tunnel: w3183 -> [_ w3240]
              tunnel: w3207 -> [w3235 w3239]
              tunnel: w3193 -> [w3234 w3238]
              tunnel: [w3234 w3238] -> w3182
              tunnel: w3188 -> [w3233 w3237]
              frame False {
                n1118 = Divide(x=w3233, y=w3235) -> (x/y=w3236:sgl[])
              }
              frame True {
                n1119 = call "IMAQ GetPixelLine"("Line Coordinates"=w3240, "Image"=w3238) -> ("Pixels Line (Float)"=w3241:sgl[])  [unwired: 2 in, 4 out]
                n1120 = Divide(x=w3237, y=w3239) -> (x/y=w3243:sgl[])
                n1121 = Add(x=w3241, y=w3243) -> (x+y=w3242:sgl[])
              }
            }
            n1122 = stacked-sequence {
              tunnel: w3183 -> [w3220 _]
              tunnel: w3181 -> [w3219 _]
              tunnel: w3182 -> [w3218 _]
              tunnel: w3184 -> [_ w3224]
              frame #0 {
                n1123 = call "IMAQ SetPixelLine"("Pixels Line (Float)"=w3219, "Line Coordinates"=w3220, "Image"=w3218) -> ()  [unwired: 7 in, 2 out]
              }
              frame #1 {
                n1124 = case shown="True" w3224 {
                  tunnel: [w3225 w3227] -> w3222
                  frame False {
                    n1125 = call "Frame Counter.vi"("Action"=Counter_Action."Read") -> ("Num"=w3225:i32)
                  }
                  frame True {
                    n1126 = call "Frame Counter.vi"("Action"=Counter_Action."Plus One") -> ("Num"=w3227:i32)
                  }
                }
                n1127 = call "FPGA-7842R-Control V2.vi"("Current Frame"=w3222, "Action"=FPGA-7842R-Reference."Current Frame for Capture", "Initialize"=TRUE) -> ()  [unwired: 11 in, 2 out]
              }
            }
            n1128 = And(x=w3198, y=w3197) -> (x .and. y?=w3199:bool)
            n1129 = case shown="True" w3199 {
              tunnel: w3181 -> [_ w3232]
              tunnel: w3208 -> [_ w3230]
              tunnel: w3192 -> [_ w3229]
              frame False {
              }
              frame True {
                n1130 = Write to Binary File(file (use dialog)=w3229, data=w3232, 5:FALSE ("prepend array or string size? (T)"), 9:w3230) -> ()  [unwired: 2 in, 3 out]
              }
            }
          }
        }
      }
    }
    frame 31 {
      n1131 = while {
        shift-right: [w3279] -> _
        shift-left: 0 -> [w3280]
        tunnel: w3258 -> [w3281]
        tunnel: w3257 -> [w3278]
        tunnel: w3256 -> [w3277]
        tunnel: w3255 -> [w3276]
        tunnel: w3244 -> [w3272]
        shift-right: [w3269] -> _
        shift-left: u32 0 -> [w3270]
        tunnel: w3253 -> [w3268]
        tunnel: w3252 -> [w3267]
        tunnel: w3251 -> [w3266]
        tunnel: w3250 -> [w3265]
        tunnel: w3245 -> [w3264]
        tunnel: w3249 -> [w3263]
        tunnel: w3248 -> [w3262]
        tunnel: w3247 -> [w3261]
        tunnel: w3246 -> [w3260]
        stop <- w3271 stop-if-true
        n1132 = Get Queue Status(queue=w3265) -> (queue out=w3273:refnum<queue>, # elements in queue=w3275:i32)  [unwired: 2 in, 6 out]
        n1133 = Get Notifier Status(notifier=w3272) -> (current notification=w3271:bool)  [unwired: 1 in, 4 out]
        n1134 = Greater Than 0?(x=w3275) -> (x > 0?=w3274:bool)
        n1135 = case shown="True" w3274 {
          tunnel: w3281 -> [_ w3315]
          tunnel: w3280 -> [w3283 w3316]
          tunnel: [w3283 w3314] -> w3279
          tunnel: w3278 -> [_ w3313]
          tunnel: w3277 -> [_ w3312]
          tunnel: w3276 -> [_ w3302]
          tunnel: w3273 -> [_ w3311]
          tunnel: w3270 -> [w3282 w3308]
          tunnel: [w3282 w3307] -> w3269
          tunnel: w3268 -> [_ w3306]
          tunnel: w3267 -> [_ w3305]
          tunnel: w3266 -> [_ w3300]
          tunnel: w3264 -> [_ w3298]
          tunnel: w3263 -> [_ w3297]
          tunnel: w3262 -> [_ _]
          tunnel: w3261 -> [_ _]
          tunnel: w3260 -> [_ _]
          frame False {
          }
          frame True {
            # "True: Last Frame of frame accum"
            # "Current Line in Frame Accum"
            # "Current Line In Frame"
            n1136 = Increment(x=w3308) -> (x+1=w3301:u32)
            n1137 = Dequeue Element(queue=w3311) -> (element=w3321:u64[])  [unwired: 2 in, 3 out]
            n1138 = Equal?(x=w3301, y=w3305) -> (x = y?=w3310:bool)
            n1139 = Greater?(x=w3301, y=w3306) -> (0:w3303:bool)
            n1140 = Greater?(x=w3301, y=w3300) -> (0:w3299:bool)
            n1141 = Split Number(x=w3321) -> (hi(x)=w3322:u32[], lo(x)=w3320:u32[])
            n1142 = Split Number(x=w3322) -> (hi(x)=w3291:u16[], lo(x)=w3290:u16[])
            n1143 = Split Number(x=w3320) -> (hi(x)=w3289:u16[], lo(x)=w3288:u16[])
            n1144 = Select(t=u32 0, s=w3310, f=w3301) -> (s? t:f=w3307:u32)
            n1145 = Increment(x=w3316) -> (x+1=w3317:i32)
            n1146 = Equal?(x=w3315, y=w3316) -> (x = y?=w3287:bool)
            n1147 = To Single Precision Float(number=w3291) -> (single precision float=w3296:sgl[])
            n1148 = To Single Precision Float(number=w3290) -> (single precision float=w3294:sgl[])
            n1149 = To Single Precision Float(number=w3289) -> (single precision float=w3295:sgl[])
            n1150 = To Single Precision Float(number=w3288) -> (single precision float=w3292:sgl[])
            n1151 = Select(t=0, s=w3287, f=w3317) -> (s? t:f=w3314:i32)
            n1152 = Compound Arithmetic op=ADD(w3296, w3294, w3295, w3292) -> (w3293:sgl[])
            n1153 = Build Array(0, w3316, w3315, w3316) -> (w3286:i32[])
            n1154 = case shown="False" w3299 {
              tunnel: [w3341 w3347] -> w3284
              tunnel: w3286 -> [_ w3345]
              tunnel: w3312 -> [w3340 w3344]
              tunnel: w3298 -> [w3339 w3343]
              tunnel: [w3339 w3343] -> w3285
              tunnel: w3293 -> [w3338 w3342]
              frame False {
                n1155 = Divide(x=w3338, y=w3340) -> (x/y=w3341:sgl[])
              }
              frame True {
                n1156 = call "IMAQ GetPixelLine"("Line Coordinates"=w3345, "Image"=w3343) -> ("Pixels Line (Float)"=w3346:sgl[])  [unwired: 2 in, 4 out]
                n1157 = Divide(x=w3342, y=w3344) -> (x/y=w3348:sgl[])
                n1158 = Add(x=w3346, y=w3348) -> (x+y=w3347:sgl[])
              }
            }
            n1159 = stacked-sequence {
              tunnel: w3286 -> [w3325 _]
              tunnel: w3284 -> [w3324 _]
              tunnel: w3285 -> [w3323 _]
              tunnel: w3287 -> [_ w3329]
              frame #0 {
                n1160 = call "IMAQ SetPixelLine"("Pixels Line (Float)"=w3324, "Line Coordinates"=w3325, "Image"=w3323) -> ()  [unwired: 7 in, 2 out]
              }
              frame #1 {
                n1161 = case shown="True" w3329 {
                  tunnel: [w3330 w3332] -> w3327
                  frame False {
                    n1162 = call "Frame Counter.vi"("Action"=Counter_Action."Read") -> ("Num"=w3330:i32)
                  }
                  frame True {
                    n1163 = call "Frame Counter.vi"("Action"=Counter_Action."Plus One") -> ("Num"=w3332:i32)
                  }
                }
                n1164 = call "FPGA-7842R-Control V2.vi"("Current Frame"=w3327, "Action"=FPGA-7842R-Reference."Current Frame for Capture", "Initialize"=TRUE) -> ()  [unwired: 11 in, 2 out]
              }
            }
            n1165 = And(x=w3303, y=w3302) -> (x .and. y?=w3304:bool)
            n1166 = case shown="True" w3304 {
              tunnel: w3284 -> [_ w3337]
              tunnel: w3313 -> [_ w3335]
              tunnel: w3297 -> [_ w3334]
              frame False {
              }
              frame True {
                n1167 = Write to Binary File(file (use dialog)=w3334, data=w3337, 5:FALSE ("prepend array or string size? (T)"), 9:w3335) -> ()  [unwired: 2 in, 3 out]
              }
            }
          }
        }
      }
    }
  }
  n1168 = Flush Queue(queue=w46) -> (queue out=w86:refnum<queue>)  [unwired: 1 in, 2 out]
  n1169 = Release Queue(queue=w86) -> ()  [unwired: 2 in, 3 out]
  n1170 = while {
    tunnel: w99 -> [w3370]
    tunnel: w123 -> [w3352]
    shift-right: [w3366] -> _
    shift-left: FALSE -> [w3365]
    tunnel: w47 -> [w3364]
    shift-right: [w3362] -> _
    shift-left: u32 0 -> [w3363]
    tunnel: w118 -> [w3358]
    tunnel: w43 -> [w3355]
    tunnel: [w3353] -> w10
    shift-right: [w3354] -> w113
    shift-left: w32 -> [w3371]
    tunnel: [w3351] -> _
    shift-right: [w3349] -> _
    shift-left: u32 0 -> [w3350]
    stop <- w3361 stop-if-true
    # "Total Lines Counter"
    n1171 = xnode "Invoke Method"("FPGA VI Reference In"=w3370, "Number of Elements"=w3350, "Timeout (ms)"=0) -> ("FPGA VI Reference Out"=w3353:refnum<k20>, "error out"=w3351:errorcluster, "Data"=w3359:u64[], "Elements Remaining"=w3368:u32)  [unwired: 1 in]
    n1172 = Get Notifier Status(notifier=w3371) -> (notifier out=w3354:refnum<notifier>, current notification=w3360:bool)  [unwired: 1 in, 3 out]
    n1173 = case shown="True" w3365 {
      tunnel: w3359 -> [_ w3374]
      tunnel: w3364 -> [_ w3380]
      tunnel: w3363 -> [w3373 w3377]
      tunnel: [w3373 w3378] -> w3362
      tunnel: [w3372 w3376] -> w3357
      tunnel: w3360 -> [w3372 _]
      tunnel: w3358 -> [_ w3375]
      frame False {
      }
      frame True {
        n1174 = Increment(x=w3377) -> (x+1=w3378:u32)
        n1175 = Enqueue Element(queue=w3380, element=w3374, timeout in ms (-1)=0) -> ()  [unwired: 1 in, 3 out]
        n1176 = Equal?(x=w3378, y=w3375) -> (x = y?=w3376:bool)
      }
    }
    n1177 = Greater Or Equal?(x=w3368, y=w3352) -> (x >= y?=w3366:bool)
    n1178 = Select(t=w3352, s=w3366, f=u32 0) -> (s? t:f=w3349:u32)
    n1179 = And(x=w3355, y=w3357) -> (x .and. y?=w3356:bool)
    n1180 = Or(x=w3356, y=w3360) -> (x .or. y?=w3361:bool)
  }
  n1181 = Send Notification(notification=TRUE, notifier=w113) -> ()  [unwired: 1 in, 2 out]
  n1182 = xnode "Invoke Method"("FPGA VI Reference In"=w10, "Number of Elements"=u32 0, "Timeout (ms)"=5000) -> ("FPGA VI Reference Out"=w14:refnum<k20>, "error out"=w11:errorcluster, "Elements Remaining"=w13:u32)  [unwired: 1 in, 1 out]
  n1183 = xnode "Invoke Method"("FPGA VI Reference In"=w14, "error in"=w11, "Number of Elements"=w13, "Timeout (ms)"=5000) -> ("FPGA VI Reference Out"=w4:refnum<k20>, "error out"=w3:errorcluster)  [unwired: 2 out]
  n1184 = xnode "Close FPGA VI Reference"("FPGA VI Reference In"=w4, "error in"=w3) -> ()  [unwired: 1 out]
